vi "findmovablepath13.vi"(8 "x":dbl) -> (0 "shift":dbl, 3 "theta handle":dbl=0.15)   [LabVIEW 2012]
uses:
  G_NAV.vi
  G_VEH.vi
  G_PATH.vi
  <vilib>/Analysis/Matrix/Numeric/Conversions/Array To Matrix - RA2.vi
  <vilib>/Analysis/7linalg.llb/Real SVD Decomposition.vi
  G_SEN.vi
  <vilib>/Analysis/NI_AALPro.lvlib
  <vilib>/Analysis/Matrix/NI_Matrix.lvlib
panel:
  out "M6006 2":T1={"GPSTime"=22892800.0, "attitude[2]"=-0.6123908162117004, "lcc[0]"=-970.4720458984375, "lcc[1]"=200.52362060546875, "heading_GPS"=-0.610690712928772} {"GPSTime" format="%#_6f"}
  in  "Numeric":dbl
  out "sensor_obs":dbl[][](array[numeric])=[[-2.6493086559458767, 9.313377271515247, 0.316177936945349, -1.2], [-2.6066100840450477, 9.354542103994737, 0.3157590885476819, -1.2], [-2.579340659822815, 9.43207739327695, 0.31450254335468053, -1.2], [-2.6132527619437576, 9.439068677849818, 0.5859163050429868, 1.2000000000000006], [-2.6655003955140795, 9.41719146151926, 0.4953083793337705, 0.40000000000000013], [-2.8189313467074544, 9.344249551531279, 0.5859163050429868, 1.2000000000000006], [-2.5692189092921667, 9.480018973387281, 0.5863351534406539, 1.2000000000000006], [-2.6731933264342116, 9.434269134901442, 0.5863351534406539, 1.2000000000000006], [-2.77635346299322, 9.386711660550553, 0.5863351534406539, 1.2000000000000006], [-2.7290628288714722, 9.419794899689457, 0.5865445776394874, 1.2000000000000006], [-3.035140869949269, 9.26885391372332, 0.5865445776394874, 1.2000000000000006], [-2.550914688564252, 9.509578404068655, 0.3132459981616791, -1.2], [-2.785425991035746, 9.405948172518677, 0.495587629745689, 0.40000000000000013], [-2.7463409502228373, 9.457274042188466, 0.4957970675546278, 0.40000000000000013], [-2.90576588154835, 9.392310316924437, 0.49586688015760744, 0.40000000000000013], [-2.494747129058042, 9.597974241579312, 0.5880105470313224, 1.2000000000000006], [-2.836998990617639, 9.447892074399023, 0.4039934946364334, -0.3999999999999999], [-3.1184925197733824, 9.303796817000539, 0.5880105470313224, 1.2000000000000006], [-2.970577318209098, 9.393517402151646, 0.4960763179665463, 0.40000000000000013], [-2.9699981982750367, 9.392368449256733, 0.588219971230156, 1.2000000000000006], [-3.0729809459427746, 9.340776068194645, 0.4960763179665463, 0.40000000000000013], [-3.1996655181339673, 9.27234939560896, 0.40392368203345375, -0.3999999999999999], [-3.4973819131319495, 9.096981036828707, 0.40392368203345375, -0.3999999999999999], [-2.5289827185611418, 9.605504378157487, 0.3115706045710105, -1.2], [-3.453631348161608, 9.135814142218397, 0.4038538694304742, -0.3999999999999999], [-3.2339632015510937, 9.274656811335685, 0.5886388196278232, 1.2000000000000006], [-2.483097010676977, 9.64588076688389, 0.3111517561733434, -1.2], [-2.8803018639560647, 9.47148380231442, 0.4962857557754851, 0.40000000000000013], [-2.9317308980723027, 9.444962161904348, 0.5888482438266567, 1.2000000000000006], [-2.9582194094409178, 9.433270224287725, 0.4037142442245149, -0.3999999999999999], [-3.0350382771601945, 9.392890956174119, 0.5888482438266567, 1.2000000000000006], [-2.4599617564514022, 9.665942841266034, 0.5890576680254903, 1.2000000000000006], [-3.1930649800894275, 9.320188914278454, 0.5890576680254903, 1.2000000000000006], [-3.424919733239901, 9.200023640728578, 0.4035746190185557, -0.3999999999999999], [-3.4490855593711203, 9.183917089574846, 0.5892670922243238, 1.2000000000000006], [-2.6822275888719656, 9.595825896338217, 0.49649519358442396, 0.40000000000000013], [-3.1777999006997932, 9.352779338748892, 0.40350480641557607, -0.3999999999999999], [-3.3543988506422, 9.251882705008573, 0.5894765164231575, 1.2000000000000006], [-2.4169315260491846, 9.715129108585124, 0.589685940621991, 1.2000000000000006], [-2.4440270491484113, 9.70452412526726, 0.3103140593780091, -1.2], [-2.4445036099706936, 9.705733945395902, 0.40343499381259645, -0.3999999999999999], [-2.8187951120879293, 9.544925625371082, 0.40343499381259645, -0.3999999999999999], [-2.923864294836344, 9.494810195959495, 0.40343499381259645, -0.3999999999999999], [-3.4095769435307015, 9.230983589588824, 0.589685940621991, 1.2000000000000006], [-3.032582634559555, 9.45177853739907, 0.40336518120961684, -0.3999999999999999], [-3.2893092213922506, 9.313834366383366, 0.40336518120961684, -0.3999999999999999], [-3.313999270308597, 9.298296139668594, 0.5898953648208245, 1.2000000000000006], [-2.424651387634039, 9.734980699717582, 0.4967046313933628, 0.40000000000000013], [-2.533097518783729, 9.691715080471495, 0.4967046313933628, 0.40000000000000013], [-2.6407720438905313, 9.646563404831404, 0.4967046313933628, 0.40000000000000013], [-3.4004241638790518, 9.27277469308272, 0.4032255560036576, -0.3999999999999999], [-2.6217419806033297, 9.676437047583807, 0.403155743400678, -0.3999999999999999], [-2.6755410498513874, 9.653323143325384, 0.403155743400678, -0.3999999999999999], [-2.782523848427478, 9.605691332564723, 0.403155743400678, -0.3999999999999999], [-3.072259099823128, 9.465159649093863, 0.496844256599322, 0.40000000000000013], [-3.1500774192579093, 9.424433970288224, 0.403155743400678, -0.3999999999999999], [-3.605192513867668, 9.159018691750026, 0.403155743400678, -0.3999999999999999], [-2.5981277248582337, 9.69583138333276, 0.5907330616161588, 1.2000000000000006], [-3.102875064220138, 9.460567540591395, 0.4030859307976984, -0.3999999999999999], [-3.3599181191701257, 9.319548891673922, 0.4030859307976984, -0.3999999999999999], [-3.385278626883318, 9.304833131837459, 0.49691406920230163, 0.40000000000000013], [-2.5247869108477885, 9.749066890716904, 0.40294630559173916, -0.3999999999999999], [-2.5792234787521573, 9.726796302794572, 0.40294630559173916, -0.3999999999999999], [-3.551164984637863, 9.238618668727831, 0.5913613342126596, 1.2000000000000006], [-2.394482152160173, 9.820127604989409, 0.5915707584114931, 1.2000000000000006], [-2.7494727028492556, 9.675416799445248, 0.40280668038577994, -0.3999999999999999], [-3.681670154810481, 9.169274879714472, 0.40280668038577994, -0.3999999999999999], [-2.349619394154346, 9.868922054648976, 0.5921990310079939, 1.2000000000000006], [-2.625703441413957, 9.761592003343525, 0.497402757423159, 0.40000000000000013], [-3.2137622211581482, 9.48110235361721, 0.497402757423159, 0.40000000000000013], [-3.7275762623275384, 9.185498662423365, 0.5924084552068274, 1.2000000000000006], [-2.3569997188774257, 9.88892730018629, 0.4975423826291182, 0.40000000000000013], [-3.6331178758069624, 9.258143332791025, 0.5926178794056609, 1.2000000000000006], [-3.280263464375405, 9.479130763175284, 0.4976121952320978, 0.40000000000000013], [-2.450699178158054, 9.884289629873633, 0.30675384799783845, -1.2], [-2.4511770399787394, 9.885534502477135, 0.40224817956194303, -0.3999999999999999], [-2.5345511058394776, 9.852902522117958, 0.49775182043805705, 0.40000000000000013], [-3.824786250125524, 9.17047880734031, 0.40224817956194303, -0.3999999999999999], [-2.405397050205525, 9.933526651907876, 0.3061255754013377, -1.2], [-3.4089243051435196, 9.464380504252652, 0.4979612582469959, 0.40000000000000013], [-3.56907303823246, 9.381650335067114, 0.4980310708499755, 0.40000000000000013], [-3.532949127216187, 9.438353586460368, 0.49824050865891434, 0.40000000000000013], [-3.737313762681747, 9.3103050041449, 0.5947121213939967, 1.2000000000000006], [-2.2908474536598415, 10.059979664182297, 0.595549818189331, 1.2000000000000006], [-2.3765186719612967, 10.02943138812595, 0.3044501818106692, -1.2], [-2.462262709016492, 9.999031326649108, 0.4985197590708328, 0.40000000000000013], [-3.657097646318684, 9.409803942456133, 0.4985197590708328, 0.40000000000000013], [-3.835868568229564, 9.295365230962426, 0.40148024092916723, -0.3999999999999999], [-2.3581413988349413, 10.067967806625958, 0.5961780907858316, 1.2000000000000006], [-3.877029743260587, 9.302385055789298, 0.5961780907858316, 1.2000000000000006], [-3.9331436519651666, 9.276595165706414, 0.5963875149846652, 1.2000000000000006], [-3.425151432335213, 9.616047962173518, 0.4989386346887105, 0.40000000000000013], [-2.3143719287589564, 10.127343415537375, 0.49900844729169014, 0.40000000000000013], [-3.7975482431761254, 9.403949992407117, 0.49900844729169014, 0.40000000000000013], [-3.854407472044735, 9.378948406292697, 0.49907825989466975, 0.40000000000000013], [-2.407763132093687, 10.115274836822742, 0.4008519275023507, -0.3999999999999999], [-2.468901871015975, 10.10337801061548, 0.4007821148993711, -0.3999999999999999], [-2.3890129763037065, 10.15395227178771, 0.4993575103065882, 0.40000000000000013], [-3.777898705712374, 9.487607060347795, 0.4994273229095678, 0.40000000000000013], [-4.0346920104398265, 9.315984499311078, 0.5982723327741674, 1.2000000000000006], [-4.015722357091047, 9.342912286209264, 0.40050286448745265, -0.3999999999999999], [-2.372846250599384, 10.200711102617147, 0.30109939462933205, -1.2], [-2.3833228936159903, 10.23029622982958, 0.4001538014725545, -0.3999999999999999], [-3.9666747963375277, 9.4365483588187, 0.4998461985274455, 0.40000000000000013], [-2.30100181314674, 10.278532756817912, 0.5999477263648358, 1.2000000000000006], [-4.109576508398126, 9.423930057048132, 0.5003348867483028, 0.40000000000000013], [-2.35334151682133, 10.334600032038626, 0.2985863042433292, -1.2], [-4.074608378760497, 9.48436394539886, 0.5005443245572416, 0.40000000000000013], [-2.3368079650044735, 10.384014278769136, 0.5007537623661805, 0.40000000000000013], [-2.370078405901655, 10.38320748736416, 0.39917642503083994, -0.3999999999999999], [-4.204212822255533, 9.504238162023881, 0.3988273620159418, -0.3999999999999999], [-2.2707767805352264, 10.48873231405309, 0.2960732138573263, -1.2], [-2.3200348724405737, 10.53572713543776, 0.6051833313356751, 1.2000000000000006], [-2.245779677656643, 10.622703152908741, 0.29356012347132354, -1.2], [-2.279884830624796, 10.622358187824348, 0.6066493007275101, 1.2000000000000006], [-2.358065997017253, 10.651060149761754, 0.5025688900436505, 0.40000000000000013], [-2.206922249961846, 10.718517420078616, 0.29188472988065495, -1.2], [-2.310815072326706, 10.718984235455277, 0.5029179530585486, 0.40000000000000013], [-2.250256927274077, 10.7470116403635, 0.6089529669146794, 1.2000000000000006], [-2.4078141528407944, 10.696197951674801, 0.2910470330853207, -1.2], [-2.2625570787999116, 10.786624601979373, 0.5032670160734467, 0.40000000000000013], [-2.37319268235858, 10.803936049039782, 0.3963839209116553, -0.3999999999999999], [-2.4400133449020482, 10.792431192800741, 0.3963141083086757, -0.3999999999999999], [-2.3484550625403937, 10.948347869936686, 0.3954763570729203, -0.3999999999999999], [-2.2532005442925973, 10.986565753726355, 0.6137697234878515, 1.2000000000000006], [-2.2241527610867795, 11.130722431723722, 0.6164922380726879, 1.2000000000000006], [-2.3272220554510197, 11.112000353866012, 0.3944291680282261, -0.3999999999999999], [-2.2968682826047866, 11.131657762965752, 0.5056406445747536, 0.40000000000000013], [-2.2805508875817773, 11.32421563798276, 0.5068972714283867, 0.40000000000000013], [-2.3203488195890745, 11.3333663356091, 0.39296310336565415, -0.3999999999999999], [-2.2253235316083524, 11.390402063747686, 0.6217278430435271, 1.2000000000000006], [-2.23390046248441, 11.420813566670208, 0.5074557722522236, 0.40000000000000013], [-2.315297365324197, 11.574401473618405, 0.391357413497123, -0.3999999999999999], [-2.2168668356954866, 11.63137340411444, 0.6265445996166993, 1.2000000000000006], [-2.3994033185138965, 11.600249851280598, 0.2730365519856337, -1.2], [-2.233080590823236, 11.690844769333019, 0.5092708999296937, 0.40000000000000013], [-2.3589382981537037, 11.726595493110718, 0.27073288579846444, -1.2], [-2.3008663461775223, 11.796656013544418, 0.38989134883455107, -0.3999999999999999], [-2.209460232985442, 11.892117815907735, 0.6317802045875385, 1.2000000000000006], [-2.2516708194251622, 11.903349900014954, 0.3892630354077345, -0.3999999999999999], [-2.324463966690179, 11.881746284197003, 0.26780094701479445, -1.2], [-2.2175289279374653, 11.922764866099948, 0.5108067771952451, 0.40000000000000013], [-2.2538194745555633, 11.911368790129554, 0.2675915228159609, -1.2], [-2.178403555854863, 12.077484518563601, 0.5117841536369597, 0.40000000000000013], [-2.1829008579162608, 12.095192687788384, 0.6357592643653763, 1.2000000000000006], [-2.2383426880850124, 12.155028982889158, 0.3875875329362237, -0.3999999999999999], [-2.2804615843118747, 12.317890670472249, 0.25921455486261813, -1.2], [-2.2227746224162255, 12.415062075134333, 0.2575391612719496, -1.2], [-2.186230627716147, 12.434387153701119, 0.6426702629268841, 1.2000000000000006], [-2.196164124819029, 12.474982005763925, 0.5145068451531648, 0.40000000000000013], [-2.1425536546232067, 12.599100045840768, 0.6458116259093877, 1.2000000000000006], [-2.2643337612516414, 12.581746676789589, 0.3846554036110799, -0.3999999999999999], [-2.198573038349574, 12.65771577116447, 0.2527224046987775, -1.2], [-2.1750587039156537, 12.73714405461915, 0.5162521602276552, 0.40000000000000013], [-2.238686482838199, 12.824800292270476, 0.38304971374254876, -0.3999999999999999], [-2.1747996213790666, 12.920092091405744, 0.24748679972793824, -1.2], [-2.1535345564869504, 13.01725329936264, 0.6543980180615641, 1.2000000000000006], [-2.187058282696622, 13.165406851352257, 0.519184289552799, 0.40000000000000013], [-2.0682676188644926, 13.230434114169201, 0.24162292216059827, -1.2], [-2.249455724453499, 13.24346320074072, 0.3801873970203845, -0.3999999999999999], [-2.168249294443763, 13.280340530506738, 0.2401569527687633, -1.2], [-2.1361605605328022, 13.338559010168616, 0.6608901682254047, 1.2000000000000006], [-2.1577943406236098, 13.438198159944571, 0.520999417230269, 0.40000000000000013], [-2.1011219599138715, 13.601533356858653, 0.6661257731962439, 1.2000000000000006], [-2.2400954133839512, 13.604417430165359, 0.377743955916098, -0.3999999999999999], [-2.1622288912277443, 13.672487145254262, 0.3773948929011999, -0.3999999999999999], [-2.0809447496291567, 13.728170217410458, 0.23136113641775338, -1.2], [-2.148368119037393, 13.828678025980699, 0.5236522961434944, 0.40000000000000013], [-2.1431530665836362, 14.033933863880375, 0.37495145179691336, -0.3999999999999999], [-2.106513383233814, 14.090157922222986, 0.6761781347402553, 1.2000000000000006], [-2.116678410658171, 14.141260966031997, 0.5257466742328829, 0.40000000000000013], [-2.0736923856429295, 14.42245242291376, 0.6828797091029295, 1.2000000000000006], [-2.0946138788714483, 14.532649102029193, 0.5283995531461083, 0.40000000000000013], [-2.152273017194013, 14.572484794069997, 0.3712513838389937, -0.3999999999999999], [-2.0231688076393577, 14.688270075344283, 0.5293769295878229, 0.40000000000000013], [-2.0756120529212976, 14.699000478760663, 0.37048344520621795, -0.3999999999999999], [-2.0476810196035475, 14.823824383301131, 0.6910472528574387, 1.2000000000000006], [8.784462172926562, 11.47924364037722, 0.6985865240154472, 1.2000000000000006], [8.643867253715156, 11.631338367097312, 0.6985865240154472, 1.2000000000000006], [-2.01182307782236, 15.20812065601524, 0.5329373723397832, 0.40000000000000013], [8.86867671544905, 11.41559660678595, 0.6990053724131143, 1.2000000000000006], [8.58702381954077, 11.72028699299172, 0.6990053724131143, 1.2000000000000006], [8.952448256526495, 11.35108640713428, 0.6994242208107815, 1.2000000000000006], [8.751204607664915, 11.589530329880938, 0.699633645009615, 1.2000000000000006], [-2.0698358361213067, 15.238622346987988, 0.36678337724829835, -0.3999999999999999], [8.78228318958885, 11.618259075505645, 0.5334958731636202, 0.40000000000000013], [9.066064089233228, 11.311820599800757, 0.7006807660037829, 1.2000000000000006], [8.586576710391817, 11.864672700124274, 0.7010996144014501, 1.2000000000000006], [8.904607069385332, 11.588375580628155, 0.5339845613844775, 0.40000000000000013], [8.9823118978036, 11.517019884769494, 0.5340543739874571, 0.40000000000000013], [-2.038520846959818, 15.363492520347437, 0.7021467353956179, 1.2000000000000006], [8.791223365347536, 11.769957155305526, 0.5342638117963959, 0.40000000000000013], [8.577157812432615, 12.002632694506751, 0.7029844321909522, 1.2000000000000006], [9.089521761789143, 11.471296644949536, 0.5344034370023552, 0.40000000000000013], [8.747614402156172, 11.874019031613333, 0.5345430622083145, 0.40000000000000013], [9.196614789945517, 11.42431028033962, 0.5347525000172533, 0.40000000000000013], [8.702856524966558, 11.977947480441758, 0.5348223126202329, 0.40000000000000013], [8.551902917074258, 12.126859885849031, 0.7044504015827872, 1.2000000000000006], [9.301763328727434, 11.37452391977877, 0.7052880983781215, 1.2000000000000006], [8.546058430068586, 12.272774370500398, 0.7065446435711229, 1.2000000000000006], [8.713762205484503, 12.13805016075561, 0.5356600638559883, 0.40000000000000013], [9.379898466547676, 11.440670196564861, 0.5357996890619475, 0.40000000000000013], [8.680290014842434, 12.256372289618902, 0.536078939473866, 0.40000000000000013], [-1.9947666269032363, 15.748326418663561, 0.5366374402977029, 0.40000000000000013], [5.4033137061696035, 14.702228724352713, 0.7105237033489606, 1.2000000000000006], [5.31065139179097, 14.760192151279867, 0.5369166907096213, 0.40000000000000013], [5.318145573506214, 14.776082090179019, 0.7111519759454614, 1.2000000000000006], [5.372647557345696, 14.763989846509837, 0.36287387148143985, -0.3999999999999999], [5.430433378499369, 14.758453624273042, 0.5372657537245195, 0.40000000000000013], [5.282599535397169, 14.828571261939807, 0.3627342462754806, -0.3999999999999999], [-2.0630447970868317, 15.828269580660534, 0.3627342462754806, -0.3999999999999999], [-2.0425899368277762, 16.04197255374355, 0.7161781567174671, 1.2000000000000006], [8.986023479525567, 16.697743175440838, 0.7844504455372108, 1.2000000000000006], [8.870510744967275, 16.775657498704163, 0.7844504455372108, 1.2000000000000006], [8.776249405862337, 16.886004939029128, 0.7852881423325451, 1.2000000000000006], [9.255378545456706, 16.596057732863006, 0.7859164149290457, 1.2000000000000006], [9.146441633836046, 16.684541131912827, 0.7861258391278794, 1.2000000000000006], [9.094705994581439, 16.85736482840408, 0.5628171664150587, 0.40000000000000013], [9.445245140600367, 16.620273164434607, 0.7886389295138823, 1.2000000000000006], [8.745638718171325, 17.096618222434593, 0.7886389295138823, 1.2000000000000006], [9.250822015437112, 16.835004830220694, 0.563305854635916, 0.40000000000000013], [8.898582257650931, 17.072593546817984, 0.563305854635916, 0.40000000000000013], [9.372609476756939, 16.761935663932476, 0.5633756672388956, 0.40000000000000013], [9.022240713238299, 17.00273744358763, 0.5633756672388956, 0.40000000000000013], [9.671704217358442, 16.690540187776413, 0.79261798929172, 1.2000000000000006], [8.733353836557999, 17.341528099528503, 0.7928274134905535, 1.2000000000000006], [9.575618663038583, 16.801373411419853, 0.5644228562835899, 0.40000000000000013], [8.86635551362631, 17.284293500790973, 0.5644228562835899, 0.40000000000000013], [-11.730647795102412, 15.437193920648374, 0.09942389115260453, -1.2], [-11.753961919567294, 15.46091854606451, 0.3329242648031848, -0.3999999999999999], [-2.6376199176507695, 22.880864643377365, 0.586553451428128, 0.40000000000000013], [-2.8095170709695823, 22.87690194098971, 0.5866930766340872, 0.40000000000000013], [-2.472177558679492, 22.932903386537202, 0.5867628892370669, 0.40000000000000013], [-2.1457138125258957, 23.092372962417727, 0.5876006404728222, 0.40000000000000013], [-1.975660428365826, 23.120301035359756, 0.5876704530758019, 0.40000000000000013], [-2.830488522803034, 23.021539526550544, 0.8631939442986329, 1.2000000000000006], [-2.321307029798844, 23.112624067398425, 0.5878798908847407, 0.40000000000000013], [-2.664069979468923, 23.075216022238337, 0.8638222168951337, 1.2000000000000006], [-2.4981915740055283, 23.137390254704062, 0.864659913690468, 1.2000000000000006], [-2.3314305321547493, 23.198157106933053, 0.8654976104858023, 1.2000000000000006], [-1.8217528316749911, 23.325992950774253, 0.5889968925324145, 0.40000000000000013], [-2.1768599709453524, 23.37676650480826, 0.8688483976671393, 1.2000000000000006], [-15.001217509405912, 16.7719561296704, 0.31016535623183017, -0.3999999999999999], [-15.131558329077535, 16.65366297795977, 0.31002573102587094, -0.3999999999999999], [-14.921984448489132, 16.935815146369087, 0.30981629321693205, -0.3999999999999999], [-15.241790010790758, 16.749485916960253, 0.026963118356189475, -1.2], [-15.133075455565274, 16.88861418597005, 0.0267536941573559, -1.2], [-15.017973364486107, 17.261437164441947, 0.3077917277305232, -0.3999999999999999], [9.64601974480163, 21.452115753566822, 0.5922780848724565, 0.40000000000000013], [9.496453028675626, 21.54978831901161, 0.8772253656204823, 1.2000000000000006], [9.33857931433906, 21.631972172843444, 0.8772253656204823, 1.2000000000000006], [9.17999443103193, 21.712775206793534, 0.8772253656204823, 1.2000000000000006], [-15.156829567346312, 17.1472706411717, 0.022774634379518044, -1.2], [9.377029264437805, 21.70662736414938, 0.5929762109022526, 0.40000000000000013], [9.544865059367709, 21.641804454240944, 0.5931158361082118, 0.40000000000000013], [9.710389454590258, 21.571913609233842, 0.8797384560064849, 1.2000000000000006], [-1.8772014233671248, 23.929435618135358, 0.8797384560064849, 1.2000000000000006], [9.095883042737146, 21.944626194626313, 0.8807855770006529, 1.2000000000000006], [9.271801932592034, 21.894917952170292, 0.5938139621380081, 0.40000000000000013], [-15.236180272734178, 17.461386956855613, 0.017120181011011648, -1.2], [9.194957789557106, 22.145529906980062, 0.5951404015946207, 0.40000000000000013], [5.3379716006680615, 24.14040468850077, 0.30115953044745974, -0.3999999999999999], [5.346343602955266, 24.94301298686431, 0.29571414741504976, -0.3999999999999999], [-16.03827076279453, 20.400810973707614, 0.28733663505749585, -0.3999999999999999], [-15.917453817284267, 20.56937941691859, 0.2870573846455774, -0.3999999999999999], [-15.794914133758107, 20.737124067829413, 0.28677813423365894, -0.3999999999999999], [-14.857892347507073, 21.847969012040384, 0.2851724443651278, -0.3999999999999999], [-15.023801434595246, 21.725328510394597, 0.2851026317621482, -0.3999999999999999], [-15.339589077483758, 21.460351215716504, 0.2851026317621482, -0.3999999999999999], [-15.650704132941332, 21.189903024072276, 0.2851026317621482, -0.3999999999999999], [-15.201556508849778, 21.61650958244562, 0.28489319395320933, -0.3999999999999999], [-14.728337374906722, 22.016057756865447, 0.2848233813502297, -0.3999999999999999], [-15.626945243640977, 21.4767441096572, 0.28370637970255586, -0.3999999999999999], [9.50763508171292, 26.73975570562619, 0.6252994460818146, 0.40000000000000013], [-1.4252219468434035, 28.59895493907886, 0.6255088838907534, 0.40000000000000013], [9.725543674751258, 26.692789231824694, 0.6255786964937331, 0.40000000000000013], [9.943355423856874, 26.64378657215293, 0.6258579469056516, 0.40000000000000013], [9.334114379546264, 26.89614247546073, 0.6258579469056516, 0.40000000000000013], [9.216574706656742, 27.200382540182076, 0.6275334493771623, 0.40000000000000013], [10.040081267648652, 26.868922071117122, 0.9827751618326013, 1.2000000000000006], [-1.4946609322957394, 29.821814277404098, 1.0022516123241232, 1.2000000000000006], [9.883884675811041, 31.803099088007194, 0.6592981837328874, 0.40000000000000013], [9.665449175747526, 31.97349509801759, 0.659926497159704, 0.40000000000000013], [10.174424429491456, 31.838119222564067, 0.6602057475716224, 0.40000000000000013], [10.17244090528941, 31.83259465007272, 1.0805762626878783, 1.2000000000000006], [-1.0364518801246452, 37.42334336490329, 0.6869439745128152, 0.40000000000000013], [10.026103833352638, 36.8130958059697, 0.6928780457660825, 0.40000000000000013], [9.743408822772697, 36.92812129013003, 0.6930874835750214, 0.40000000000000013], [10.347031193921643, 36.82288619877287, 1.1808904539291583, 1.2000000000000006], [-21.069030510629236, 31.45954783569295, 0.20558607696836614, -0.3999999999999999], [-21.391355310423045, 31.377757000004777, 0.20467851312963112, -0.3999999999999999], [10.4210427571751, 41.72394225688742, 0.7265975330052368, 0.40000000000000013], [10.107451026305094, 41.89078819565647, 0.7271560338290737, 0.40000000000000013], [10.474235594988285, 41.919051326913184, 1.284136583954108, 1.2000000000000006], [10.13857155297352, 42.00899223589921, 1.284136583954108, 1.2000000000000006], [10.830210018606069, 41.90102810572798, 0.7285522858886659, 0.40000000000000013], [-0.709038750028526, 57.66347671663537, 1.5846603092802805, 1.2000000000000006], [11.120605021860856, 56.96437033164037, 0.8312466248716806, 0.40000000000000013], [-0.7151980727209852, 58.133987434462625, 0.8314560626806193, 0.40000000000000013], [1.5195348183779678, 61.52869356204023, 0.04473783970333195, -0.3999999999999999], [5.073212151726797, 61.48708023724171, 0.04362083805565814, -0.3999999999999999], [11.439817695944253, 61.011847285540675, 0.8593811038724656, 0.40000000000000013], [11.689176472740309, 65.06866600393317, 0.8875155828732506, 0.40000000000000013], [14.49832831315618, 65.07219891982305, 1.7750269060199955, 1.2000000000000006], [8.818111571073048, 72.81602044955893, 1.9136657256478184, 1.2000000000000006], [12.551831810983316, 72.91253923612891, 0.9424581014182081, 0.40000000000000013], [13.768405529858791, 72.71844886386302, 1.9283254195661683, 1.2000000000000006], [1.2476421313017925, 74.97736983119862, -0.04909029870127124, -0.3999999999999999], [0.9387629168292289, 75.21210795753403, 0.9506959885698028, 0.40000000000000013], [17.77975821366545, 76.1598746565128, 2.0169118556727685, 1.2000000000000006], [47.35648972259149, 63.571420836353425, 2.052304545275642, 1.2000000000000006], [13.031972557350265, 79.3416128979354, 2.061938058421986, 1.2000000000000006], [24.83184721270082, 81.07466865802802, 2.156178947897092, 1.2000000000000006], [13.551875448365177, 86.71163580640813, 1.0385900557211387, 0.40000000000000013], [52.872675769586, 69.37798867554798, 2.2194250559448303, 1.2000000000000006], [8.915518332671137, 92.0400907270114, 1.0712623539155988, 0.40000000000000013], [9.692181670683942, 91.99867908899289, 1.0715416043275172, 0.40000000000000013], [20.71894414488982, 95.06455786989261, 2.4164932270472192, 1.2000000000000006], [19.150342204408794, 95.56882049865551, 2.4198440142285564, 1.2000000000000006], [23.490178905085354, 95.9928006820069, 2.448953977866423, 1.2000000000000006], [26.036285319817722, 95.81770414584793, 2.4592157636092677, 1.2000000000000006], [14.717578948116746, 99.12164584891, 1.1254369338277803, 0.40000000000000013], [20.65463162219833, 155.2673630873944, 3.658378726130288, 1.2000000000000006], [12.312708261276875, 191.3556263648354, 4.393457664036117, 1.2000000000000006], [14.978259637770336, 232.0240814937235, 2.048848233439155, 0.40000000000000013], [33.73593705129936, 288.53349296533526, 2.4538311433239053, 0.40000000000000013], [8.92096999050232, 17.23708913161584, 0.3356469563193898, -0.3999999999999999], [-2.5256202703736608, 22.68399055587274, 0.31491261323444397, -0.3999999999999999], [-1.8996165215080512, 23.228271875851924, 0.3116314208944021, -0.3999999999999999], [-3.0296332585078587, 23.183843349397314, 0.8671730040764709, 1.2000000000000006], [5.104128617356655, 23.236200962780366, 0.022984058578351618, -1.2], [-1.2548826959515347, 24.01715071826592, 0.01942384719818102, -1.2], [5.221948215230284, 24.444090337557157, -0.0021468452816766903, -1.2], [-2.224688830349968, 25.593404278777417, 0.9151311456093583, 1.2000000000000006], [5.209357772395169, 25.198536731676327, -0.017434811796527283, -1.2], [-1.1725915542855405, 25.874379726198075, -0.019319629586029397, -1.2], [-15.005798944565672, 21.383214801932546, -0.039005504276384995, -1.2], [-14.976356804490646, 21.66777357175441, -0.04319398825305637, -1.2], [-14.955664951264778, 21.9687081224078, -0.04780132062739484, -1.2], [9.275033221452706, 26.45651279141699, 0.277143995022472, -0.3999999999999999], [9.363878146139614, 27.271589550954324, 0.2716287993870824, -0.3999999999999999], [9.371321144452127, 28.564736959442584, 0.26318147442654893, -0.3999999999999999], [10.747513637749273, 30.43885569655537, 1.0575396008161857, 1.2000000000000006], [11.012472531760006, 30.418068389611857, 1.0592149944068543, 1.2000000000000006], [11.266285997376329, 30.367042635463775, 1.060262115401022, 1.2000000000000006], [-20.735017036098906, 31.521767273772653, 0.20663326601306034, -0.3999999999999999], [-20.49557227262787, 31.709735125755284, 0.20656345341008076, -0.3999999999999999], [10.724864676049275, 37.00446773130826, 0.6956007372822874, 0.40000000000000013], [-21.806198041420327, 31.41066071306105, 0.20272376024620187, -0.3999999999999999], [10.97816933233072, 46.72664514439962, 0.7613642092890853, 0.40000000000000013], [-33.95444016665767, 37.454440166657676, 0.11475988049188635, -0.3999999999999999], [-33.46782468155926, 38.15694699438283, 0.11364287884421248, -0.3999999999999999], [-32.258000408687934, 39.32613895725404, 0.11343344103527364, -0.3999999999999999], [-34.39923085728631, 37.30403001674005, 0.11329381582931441, -0.3999999999999999], [11.618566184124763, 57.01187131155995, 0.8322938139163747, 0.40000000000000013], [16.615400312068406, 60.50485600252477, 1.6937703168725702, 1.2000000000000006], [13.205163345895427, 64.3192947748755, 1.7536656377389712, 1.2000000000000006], [20.538690765112868, 64.00503191176435, 1.7884300547453438, 1.2000000000000006], [13.026046392769018, 79.30712465157343, 0.9869985421192027, 0.40000000000000013], [27.29899080749756, 81.67230442986731, 2.1844512147396244, 1.2000000000000006], [33.69042505267091, 80.06731529671714, 2.2022522716404778, 1.2000000000000006], [29.157427120978678, 82.5346645544511, 2.2146082993716583, 1.2000000000000006], [27.17382907061827, 93.78874887901951, 2.425079619199396, 1.2000000000000006], [34.761055666251615, 92.88790635480824, 2.4590063394104344, 1.2000000000000006], [-2.729118001525531, 22.918683596868465, 0.31309748555697403, -0.3999999999999999], [9.124522914489708, 21.80096170236561, 0.3072332269066863, -0.3999999999999999], [-1.5170192378515415, 28.303045293335575, 0.2765156815956554, -0.3999999999999999], [-1.3900091234452605, 30.022954081648294, 0.2645777264861412, -0.3999999999999999], [4.034616118215339, 61.19769858054814, 0.04620390436590388, -0.3999999999999999], [26.121526235859253, 82.71602090547535, 2.197226090868472, 1.2000000000000006]]
  out "xplot":cluster{dbl[]}[](array[cluster])
  out "yplot":cluster{dbl[]}[](array[cluster])
  out "thetaseed":dbl[](array[numeric])
  out "center":i16
  out "right":i16
  out "left":i16
  out "XY Graph":cluster{"Y":dbl[], "Y":dbl[]}[](graph)=[{"Y"=[0.0], "Y"=[1000.0]}, {"Y"=[], "Y"=[]}, {"Y"=[], "Y"=[]}, {"Y"=[55.79381017995934], "Y"=[-143.41137512848826]}, {"Y"=[1.8243630881955273], "Y"=[-0.6091599202647308]}, {"Y"=[60.825233010671326, 56.37330625127248, 55.349089235151354, 59.801015994550255, 60.825233010671326], "Y"=[-144.72018116547483, -142.44414335187238, -144.44751039360185, -146.72354820720435, -144.72018116547483]}, {"Y"=[0.0, 2.210107140854234e-06, 8.840428449730098e-06, 1.9890964154001267e-05, 3.536171391260723e-05, 5.5252677611861145e-05, 7.956385525176302e-05, 0.00010829524660493917, 0.00014144685155770276, 0.0001790186695416196, 0.00022101070067037654, 0.00026742294460291305, 0.00031825540077079495, 0.00037350806894664856, 0.0004331809489031002, 0.0004972740399580289, 0.0005657873416566872, 0.0006387208537717015, 0.0007160745756209508, 0.0007978485066360008, 0.0008840426462484174, 0.0009746569938897665, 0.0010696915488779268, 0.0011691463105307776, 0.0012730212781661976, 0.001381316451102066, 0.0014940318285425747, 0.0016111674095782291, 0.0017327231935269083, 0.0018586991794791174, 0.001989095366525362, 0.00212391175364246, 0.002263148340148291, 0.0024068051247922995, 0.002554882106551304, 0.0027073792846294964, 0.002864296657776322, 0.003025634224741225, 0.003191391984614711, 0.0033615699362599116, 0.003536168078198898, 0.0037151864094084885, 0.003898624928524441, 0.004086483634296201, 0.004278762525359525, 0.004475461600350172, 0.0046765808579039, 0.004882120296656467, 0.0050920799150162566, 0.00530645971150534, 0.005525259684645789, 0.005748479832959674, 0.005976120154741693, 0.006208180648513917, 0.006444661312457356, 0.006685562145094082, 0.006930883144491418, 0.007180624309171435, 0.007434785636974084, 0.007693367126535122, 0.007956368775921874, 0.008223790583087975, 0.008495632546100751, 0.008771894663368585, 0.009052576932504053, 0.00933767935191554, 0.009627201919329309, 0.009921144632812684, 0.010219507490205615, 0.010522290489461739, 0.010829493628421005, 0.011141116904923365, 0.011457160316581394, 0.011777623861462416, 0.012102507536951634, 0.012431811341116372, 0.012765535271228146, 0.013103679325240591, 0.0134462435006526, 0.013793227794963059, 0.014144632205784546, 0.014500456730615952, 0.014860701366956164, 0.015225366112190386, 0.015594450963703821, 0.015967955919109045, 0.0163458809754502, 0.016728226130226176, 0.017114991380822175, 0.017506176724168654, 0.0179017821577645, 0.018301807678767545, 0.018706253284335617, 0.019115118971512857, 0.019528404737457095, 0.01994611057932616, 0.02036823649393682, 0.02079478247856059, 0.021225748530014243, 0.02166113464522823, 0.022100940821246695], "Y"=[0.0, 0.05249999993797367, 0.10499999950378934, 0.15749999832528905, 0.2099999960303148, 0.26249999224670867, 0.31499998660231265, 0.3674999787249688, 0.41999996824251923, 0.472499954782806, 0.5249999379736712, 0.577499917442957, 0.6299998928185055, 0.682499863728159, 0.7349998297997596, 0.7874997906611497, 0.8399997459401715, 0.8924996952646672, 0.9449996382624795, 0.9974995745614504, 1.0499995037894228, 1.1024994255742389, 1.1549993395437415, 1.2074992453257731, 1.2599991425481762, 1.3124990308387938, 1.3649989098254687, 1.4174987791360436, 1.4699986383983614, 1.5224984872402658, 1.574998325289599, 1.6274981521742047, 1.6799979675219257, 1.7324977709606055, 1.784997562118088, 1.837497340622216, 1.8899971061008334, 1.9424968581817836, 1.994996596492911, 2.047496320662059, 2.099996030317072, 2.152495725085793, 2.204995404596067, 2.2574950684757384, 2.309994716352652, 2.3624943478546507, 2.414993962609581, 2.467493560245286, 2.519993140389611, 2.5724927026704023, 2.6249922467155042, 2.6774917721527607, 2.7299912786100196, 2.7824907657151243, 2.834990233095921, 2.887489680380256, 2.939989107195975, 2.9924885131709242, 3.0449878979329497, 3.0974872611098974, 3.1499866023296144, 3.2024859212199472, 3.2549852174087435, 3.3074844905238483, 3.3599837401931105, 3.412482966044377, 3.464982167705495, 3.5174813448043127, 3.5699804969686775, 3.6224796238264374, 3.6749787250054404, 3.7274778001335362, 3.7799768488385714, 3.8324758707483966, 3.884974865490859, 3.9374738326938097, 3.989972771985096, 4.042471682992569, 4.094970565344078, 4.147469418667473, 4.199968242590603, 4.2524670367413195, 4.304965800747474, 4.3574645342369145, 4.409963236837495, 4.4624619081770645, 4.514960547883476, 4.567459155584579, 4.6199577309082285, 4.672456273482274, 4.724954782934569, 4.777453258892966, 4.829951700985317, 4.882450108839476, 4.934948482083297, 4.987446820344632, 5.039945123251335, 5.09244339043126, 5.144941621512262, 5.197439816122197, 5.249937973888915]}, {"Y"=[55.85492946607054, 56.300112183962334, 56.74529490185413, 57.19047761974598, 57.635660337637766, 58.08084305552956, 58.52602577342136, 58.97120849131315, 59.416391209205, 59.8615739270968, 60.306756644988596, 60.75193936288038, 61.197122080772175, 61.64230479866403, 62.087487516555825, 62.532670234447615, 62.97785295233941, 63.423035670231265, 63.86821838812306, 64.31340110601485, 64.75858382390665, 65.20376654179844, 65.64894925969023, 66.09413197758208, 66.53931469547388, 66.98449741336567, 67.42968013125746, 67.87486284914931, 68.3200455670411, 68.7652282849329, 69.2104110028247, 69.65559372071655, 70.10077643860835, 70.54595915650015, 70.99114187439193, 71.43632459228371, 71.88150731017556, 72.32669002806736, 72.77187274595916, 73.21705546385095], "Y"=[-143.26925304077835, -143.49687629901547, -143.72449955725253, -143.95212281548962, -144.17974607372668, -144.40736933196374, -144.63499259020085, -144.8626158484379, -145.090239106675, -145.3178623649121, -145.54548562314918, -145.7731088813862, -146.00073213962332, -146.22835539786038, -146.45597865609744, -146.68360191433456, -146.91122517257162, -147.1388484308087, -147.36647168904577, -147.59409494728285, -147.82171820551994, -148.04934146375703, -148.27696472199406, -148.50458798023115, -148.73221123846827, -148.9598344967053, -149.18745775494241, -149.4150810131795, -149.64270427141656, -149.87032752965362, -150.09795078789074, -150.3255740461278, -150.55319730436486, -150.78082056260195, -151.00844382083903, -151.23606707907612, -151.46369033731318, -151.6913135955503, -151.91893685378736, -152.14656011202442]}, {"Y"=[46.95734422441421, 47.0463827596022, 47.13542129479015, 47.224459829978144, 47.31349836516614, 47.40253690035408, 47.49157543554208, 47.58061397073008, 47.669652505918016, 47.75869104110601, 47.84772957629395, 47.936768111481946, 48.02580664666995, 48.11484518185789, 48.20388371704588, 48.292922252233886, 48.381960787421825, 48.47099932260982, 48.56003785779782, 48.64907639298576, 48.73811492817376, 48.827153463361746, 48.91619199854969, 49.00523053373769, 49.09426906892568, 49.18330760411363, 49.272346139301625, 49.361384674489564, 49.45042320967757, 49.53946174486556, 49.6285002800535, 49.717538815241504, 49.8065773504295, 49.89561588561743, 49.984654420805434, 50.07369295599343, 50.16273149118137, 50.251770026369364, 50.34080856155737, 50.429847096745306, 50.5188856319333, 50.607924167121304, 50.69696270230924, 50.78600123749724, 50.875039772685184, 50.96407830787318, 51.05311684306117, 51.142155378249115, 51.23119391343711, 51.320232448625106, 51.40927098381305, 51.49830951900105, 51.58734805418904, 51.67638658937698, 51.765425124564985, 51.85446365975298, 51.94350219494092, 52.03254073012892, 52.12157926531691, 52.21061780050485, 52.29965633569285, 52.38869487088079, 52.477733406068786, 52.56677194125679, 52.65581047644473, 52.74484901163272, 52.833887546820726, 52.922926082008665, 53.01196461719666, 53.10100315238466, 53.190041687572595, 53.27908022276059, 53.36811875794859, 53.45715729313653, 53.54619582832453, 53.635234363512524, 53.72427289870047, 53.813311433888465, 53.902349969076404, 53.99138850426441, 54.0804270394524, 54.16946557464034, 54.25850410982834, 54.34754264501633, 54.43658118020427, 54.525619715392274, 54.61465825058027, 54.70369678576821, 54.792735320956204, 54.88177385614421, 54.970812391332146, 55.05985092652014, 55.148889461708144, 55.23792799689608, 55.32696653208408, 55.41600506727202, 55.50504360246001, 55.59408213764801, 55.683120672835955, 55.77215920802395, 55.861197743211946, 55.95023627839994, 56.03927481358789, 56.12831334877588, 56.21735188396388, 56.306390419151825, 56.39542895433982, 56.48446748952781, 56.573506024715755, 56.66254455990375, 56.75158309509169, 56.84062163027969, 56.92966016546769, 57.01869870065563, 57.10773723584363, 57.196775771031625, 57.285814306219564, 57.37485284140757, 57.46389137659556, 57.552929911783494, 57.64196844697149, 57.73100698215949, 57.82004551734743, 57.90908405253543, 58.08716112291137, 58.176199658099364, 58.26523819328731, 58.354276728475305, 58.4433152636633, 58.53235379885125, 58.62139233403924, 58.71043086922723, 58.79946940441518, 58.88850793960317, 58.97754647479111, 59.06658500997911, 59.15562354516711, 59.24466208035505, 59.333700615543044, 59.42273915073105, 59.511777685918986, 59.60081622110698, 59.689854756294984, 59.778893291482916, 59.86793182667091, 59.956970361858914, 60.04600889704685, 60.13504743223485, 60.31312450261079, 60.402163037798786, 60.491201572986725, 60.58024010817473, 60.66927864336272, 60.75831717855066, 60.84735571373866, 60.93639424892665, 61.02543278411459, 61.114471319302595, 61.203509854490534, 61.29254838967853, 61.38158692486653, 61.47062546005447, 61.55966399524247, 61.64870253043047, 61.73774106561841, 61.826779600806404, 61.91581813599439, 62.00485667118234, 62.093895206370334, 62.18293374155833, 62.271972276746276, 62.36101081193427, 62.45004934712227, 62.53908788231021, 62.62812641749821, 62.71716495268615, 62.80620348787415, 62.895242023062146, 62.984280558250084, 63.07331909343808, 63.162357628626076, 63.251396163814015, 63.34043469900201, 63.42947323419001, 63.51851176937796, 63.60755030456595, 63.69658883975394, 63.78562737494189, 63.87466591012988, 63.96370444531783, 64.05274298050581, 64.14178151569382, 64.23082005088176, 64.31985858606976, 64.40889712125775, 64.4979356564457, 64.58697419163369, 64.76505126200964, 64.85408979719762, 64.94312833238557, 65.03216686757357, 65.12120540276156, 65.2102439379495, 65.29928247313751, 65.38832100832549, 65.47735954351344, 65.56639807870144, 65.65543661388938, 65.74447514907737, 65.83351368426537, 65.92255221945331, 66.0115907546413, 66.10062928982931, 66.18966782501724, 66.27870636020525, 66.36774489539324, 66.45678343058118, 66.54582196576918, 66.63486050095719, 66.72389903614511, 66.81293757133312, 66.9019761065211, 66.99101464170904, 67.08005317689705, 67.16909171208498, 67.25813024727299, 67.34716878246098, 67.43620731764892, 67.52524585283692, 67.61428438802493, 67.70332292321285, 67.79236145840086, 67.88139999358886, 67.97043852877678, 68.05947706396479, 68.14851559915279, 68.23755413434073, 68.32659266952872, 68.41563120471668, 68.50466973990466, 68.59370827509267, 68.6827468102806, 68.7717853454686, 68.8608238806566, 68.94986241584455, 69.03890095103253, 69.12793948622053, 69.21697802140848, 69.30601655659646, 69.39505509178447, 69.48409362697241, 69.5731321621604, 69.6621706973484, 69.75120923253635, 69.84024776772434, 69.92928630291229, 70.01832483810027, 70.10736337328828, 70.19640190847622, 70.2854404436642, 70.37447897885221, 70.46351751404015, 70.55255604922814, 70.64159458441614, 70.7306331196041, 70.81967165479207, 70.90871018998008, 70.99774872516802, 71.08678726035602, 71.17582579554401, 71.26486433073195, 71.35390286591995, 71.44294140110789, 71.5319799362959, 71.62101847148388, 71.71005700667183, 71.79909554185983, 71.88813407704782, 71.97717261223576, 72.06621114742377, 72.15524968261175, 72.2442882177997, 72.3333267529877, 72.42236528817568, 72.51140382336364, 72.60044235855163, 72.68948089373963, 72.77851942892757, 72.86755796411556, 72.9565964993035, 73.04563503449151, 73.13467356967949, 73.22371210486745, 73.31275064005544, 73.40178917524342, 73.49082771043138, 73.57986624561937], "Y"=[-138.89375124553214, -138.93927200180423, -138.98479275807625, -139.0303135143483, -139.07583427062036, -139.12135502689242, -139.16687578316444, -139.21239653943653, -139.25791729570855, -139.30343805198058, -139.34895880825266, -139.3944795645247, -139.44000032079677, -139.4855210770688, -139.53104183334085, -139.5765625896129, -139.62208334588496, -139.667604102157, -139.71312485842907, -139.7586456147011, -139.80416637097318, -139.8496871272452, -139.89520788351723, -139.9407286397893, -139.98624939606134, -140.0317701523334, -140.07729090860545, -140.1228116648775, -140.16833242114956, -140.2138531774216, -140.25937393369364, -140.30489468996572, -140.35041544623775, -140.39593620250977, -140.44145695878186, -140.48697771505388, -140.53249847132597, -140.578019227598, -140.62353998387005, -140.66906074014207, -140.71458149641416, -140.76010225268618, -140.80562300895826, -140.8511437652303, -140.89666452150234, -140.9421852777744, -140.98770603404643, -141.0332267903185, -141.07874754659053, -141.1242683028626, -141.16978905913462, -141.2153098154067, -141.26083057167872, -141.3063513279508, -141.35187208422283, -141.3973928404949, -141.44291359676694, -141.48843435303897, -141.53395510931105, -141.57947586558308, -141.62499662185516, -141.67051737812716, -141.71603813439924, -141.76155889067127, -141.80707964694335, -141.85260040321535, -141.89812115948743, -141.94364191575949, -141.9891626720315, -142.0346834283036, -142.08020418457562, -142.1257249408477, -142.1712456971197, -142.21676645339178, -142.2622872096638, -142.3078079659359, -142.3533287222079, -142.39884947847997, -142.44437023475203, -142.48989099102408, -142.53541174729614, -142.58093250356816, -142.62645325984025, -142.67197401611224, -142.71749477238433, -142.76301552865635, -142.80853628492844, -142.85405704120046, -142.89957779747255, -142.94509855374454, -142.99061931001663, -143.03614006628868, -143.0816608225607, -143.1271815788328, -143.17270233510482, -143.2182230913769, -143.2637438476489, -143.30926460392098, -143.354785360193, -143.4003061164651, -143.4458268727371, -143.4913476290092, -143.5368683852812, -143.58238914155328, -143.62790989782533, -143.67343065409736, -143.71895141036944, -143.76447216664147, -143.80999292291352, -143.85551367918555, -143.90103443545763, -143.94655519172966, -143.99207594800174, -144.03759670427374, -144.08311746054582, -144.12863821681785, -144.1741589730899, -144.21967972936199, -144.265200485634, -144.3107212419061, -144.3562419981781, -144.40176275445017, -144.4472835107222, -144.49280426699428, -144.58384577953836, -144.6293665358104, -144.67488729208247, -144.72040804835453, -144.76592880462653, -144.81144956089864, -144.85697031717064, -144.90249107344272, -144.94801182971474, -144.99353258598683, -145.03905334225882, -145.0845740985309, -145.13009485480293, -145.17561561107502, -145.22113636734704, -145.2666571236191, -145.31217787989118, -145.35769863616318, -145.40321939243526, -145.4487401487073, -145.49426090497937, -145.5397816612514, -145.58530241752348, -145.63082317379548, -145.7218646863396, -145.76738544261164, -145.8129061988837, -145.85842695515572, -145.90394771142783, -145.94946846769983, -145.9949892239719, -146.04050998024394, -146.08603073651602, -146.13155149278802, -146.1770722490601, -146.22259300533213, -146.2681137616042, -146.31363451787624, -146.3591552741483, -146.40467603042035, -146.45019678669237, -146.49571754296446, -146.54123829923648, -146.58675905550857, -146.6322798117806, -146.67780056805265, -146.72332132432467, -146.76884208059676, -146.81436283686878, -146.85988359314084, -146.9054043494129, -146.95092510568492, -146.99644586195703, -147.04196661822903, -147.0874873745011, -147.13300813077313, -147.17852888704522, -147.22404964331722, -147.2695703995893, -147.31509115586132, -147.3606119121334, -147.40613266840543, -147.4516534246775, -147.49717418094954, -147.54269493722157, -147.58821569349365, -147.63373644976568, -147.67925720603776, -147.72477796230976, -147.77029871858184, -147.81581947485387, -147.86134023112595, -147.90686098739798, -147.9979024999421, -148.0434232562141, -148.08894401248617, -148.13446476875822, -148.17998552503028, -148.22550628130233, -148.27102703757438, -148.3165477938464, -148.3620685501185, -148.40758930639052, -148.45311006266255, -148.49863081893463, -148.54415157520666, -148.58967233147874, -148.63519308775076, -148.6807138440228, -148.72623460029487, -148.77175535656693, -148.81727611283895, -148.86279686911104, -148.90831762538306, -148.95383838165512, -148.99935913792717, -149.0448798941992, -149.09040065047128, -149.1359214067433, -149.18144216301536, -149.22696291928742, -149.27248367555944, -149.31800443183153, -149.36352518810358, -149.4090459443756, -149.4545667006477, -149.50008745691972, -149.54560821319174, -149.59112896946382, -149.63664972573585, -149.68217048200793, -149.72769123827996, -149.77321199455199, -149.81873275082407, -149.86425350709612, -149.90977426336815, -149.95529501964023, -150.00081577591226, -150.0463365321843, -150.09185728845637, -150.1373780447284, -150.18289880100048, -150.2284195572725, -150.27394031354456, -150.3194610698166, -150.36498182608864, -150.4105025823607, -150.45602333863278, -150.5015440949048, -150.54706485117688, -150.5925856074489, -150.63810636372094, -150.68362711999302, -150.72914787626505, -150.7746686325371, -150.82018938880915, -150.86571014508118, -150.91123090135326, -150.9567516576253, -151.00227241389734, -151.04779317016943, -151.09331392644145, -151.13883468271348, -151.18435543898556, -151.2298761952576, -151.27539695152967, -151.3209177078017, -151.36643846407375, -151.4119592203458, -151.45747997661783, -151.5030007328899, -151.54852148916194, -151.594042245434, -151.63956300170608, -151.6850837579781, -151.73060451425013, -151.77612527052221, -151.82164602679424, -151.8671667830663, -151.91268753933835, -151.95820829561038, -152.00372905188246, -152.04924980815449, -152.09477056442654, -152.14029132069862, -152.18581207697065, -152.23133283324267, -152.27685358951476, -152.32237434578678, -152.36789510205887, -152.4134158583309, -152.45893661460295, -152.504457370875]}, {"Y"=[], "Y"=[]}, {"Y"=[], "Y"=[]}, {"Y"=[], "Y"=[]}, {"Y"=[-16.5, -15.25, -15.0, -13.5, -13.25, -13.25, -13.25, -13.0, -13.0, -12.75, -12.75, -12.75, -12.75, -12.75, -12.75, -12.75, -12.5, -12.5, -12.5, -12.5, -12.5, -12.5, -12.25, -12.25, -12.25, -12.25, -12.25, -12.25, -12.0, -12.0, -12.0, -11.75, -11.75, -11.75, -11.5, -11.5, -11.5, -11.5, -11.5, -11.25, -10.75, -10.75, -10.5, -10.5, -10.25, -10.25, -10.0, -10.0, -10.0, -10.0, -10.0, -9.75, -9.75, -9.75, -9.75, -9.75, -9.75, -9.75, -9.75, -9.75, -9.75, -9.5, -9.5, -9.5, -9.5, -9.5, -9.5, -9.5, -9.5, -9.5, -9.5, -9.5, -9.5, -9.5, -9.5, -9.5, -9.5, -9.5, -9.5, -9.5, -9.25, -9.25, -9.25, -9.25, -9.25, -9.25, -9.25, -9.25, -9.25, -9.25, -9.25, -9.25, -9.25, -9.25, -9.25, -9.25, -9.25, -9.25, -9.25, -9.25, -9.25, -9.25, -9.0, -9.0, -9.0, -9.0, -9.0, -9.0, -9.0, -9.0, -9.0, -9.0, -9.0, -9.0, -9.0, -9.0, -9.0, -9.0, -9.0, -9.0, -9.0, -9.0, -9.0, -9.0, -9.0, -9.0, -9.0, -9.0, -8.75, -8.75, -8.75, -8.75, -8.75, -8.75, -8.75, -8.75, -8.75, -8.75, -8.75, -8.75, -8.75, -8.75, -8.75, -8.75, -8.75, -8.75, -8.75, -8.75, -8.75, -8.75, -8.75, -8.75, -8.75, -8.75, -8.75, -8.75, -8.75, -8.75, -8.75, -8.75, -8.75, -8.75, -8.75, -8.75, -8.75, -8.5, -8.5, -8.5, -8.5, -8.5, -8.5, -8.5, -8.5, -8.5, -8.5, -8.5, -8.5, -8.5, -8.5, -8.5, -8.5, -8.5, -8.5, -8.5, -8.5, -8.5, -8.5, -8.5, -8.5, -8.5, -8.5, -8.5, -8.5, -8.5, -8.5, -8.5, -8.5, -8.5, -8.5, -8.5, -8.5, -8.25, -8.25, -8.25, -8.25, -8.25, -8.25, -8.25, -8.25, -8.25, -8.25, -8.25, -8.25, -8.25, -8.25, -8.25, -8.25, -8.25, -8.25, -8.25, -8.25, -8.25, -8.25, -8.25, -8.25, -8.25, -8.25, -8.25, -8.25, -8.25, -8.25, -8.25, -8.25, -8.25, -8.0, -8.0, -8.0, -8.0, -8.0, -8.0, -8.0, -8.0, -8.0, -8.0, -8.0, -8.0, -8.0, -8.0, -8.0, -8.0, -8.0, -8.0, -8.0, -8.0, -8.0, -8.0, -8.0, -8.0, -8.0, -7.75, -7.75, -7.75, -7.75, -7.75, -7.75, -7.75, -7.75, -7.75, -7.75, -7.75, -7.75, -7.75, -7.75, -7.75, -7.75, -7.75, -7.75, -7.75, -7.75, -7.75, -7.75, -7.75, -7.75, -7.75, -7.75, -7.5, -7.5, -7.5, -7.5, -7.5, -7.5, -7.5, -7.5, -7.5, -7.5, -7.5, -7.5, -7.5, -7.5, -7.5, -7.5, -7.5, -7.5, -7.5, -7.5, -7.5, -7.5, -7.5, -7.5, -7.5, -7.25, -7.25, -7.25, -7.25, -7.25, -7.25, -7.25, -7.25, -7.25, -7.25, -7.25, -7.25, -7.25, -7.25, -7.25, -7.25, -7.25, -7.25, -7.25, -7.25, -7.25, -7.25, -7.25, -7.0, -7.0, -7.0, -7.0, -7.0, -7.0, -7.0, -7.0, -7.0, -7.0, -7.0, -7.0, -7.0, -7.0, -7.0, -7.0, -7.0, -7.0, -7.0, -6.75, -6.75, -6.75, -6.75, -6.75, -6.75, -6.75, -6.75, -6.75, -6.75, -6.75, -6.75, -6.75, -6.75, -6.75, -6.75, -6.75, -6.75, -6.75, -6.75, -6.75, -6.75, -6.75, -6.5, -6.5, -6.5, -6.5, -6.5, -6.5, -6.5, -6.5, -6.5, -6.5, -6.5, -6.5, -6.5, -6.5, -6.5, -6.5, -6.5, -6.5, -6.5, -6.5, -6.5, -6.5, -6.5, -6.5, -6.5, -6.5, -6.5, -6.5, -6.5, -6.5, -6.25, -6.25, -6.25, -6.25, -6.25, -6.25, -6.25, -6.25, -6.25, -6.25, -6.25, -6.25, -6.25, -6.25, -6.25, -6.25, -6.25, -6.0, -6.0, -6.0, -6.0, -6.0, -6.0, -6.0, -6.0, -6.0, -6.0, -6.0, -5.75, -5.75, -5.75, -5.75, -5.75, -5.75, -5.75, -5.75, -5.75, -5.75, -5.5, -5.25, -5.0, -4.75, -4.5, -4.5, -4.25, -4.25, -4.0, -4.0, -3.75, -3.75, -3.5, -3.5, -3.25, -3.25, -3.25, -3.25, -3.0, -3.0, 2.0, 2.0, 2.0, 2.0, 2.0, 2.0, 2.0, 2.25, 2.25, 2.25, 2.25, 2.25, 2.25, 2.25, 2.25, 2.25, 2.25, 2.25, 2.25, 2.25, 2.25, 2.25, 2.25, 2.25, 2.25, 2.25, 2.25, 2.25, 2.25, 2.5, 2.5, 2.5, 2.5, 2.5, 2.5, 2.5, 2.5, 2.5, 2.5, 2.5, 2.5, 2.5, 2.5, 2.5, 2.5, 2.5, 2.5, 2.5, 2.5, 2.5, 2.5, 2.5, 2.5, 2.5, 2.5, 2.5, 2.5, 2.5, 2.5, 2.5, 2.5, 2.5, 2.5, 2.5, 2.5, 2.5, 2.5, 2.5, 2.5, 2.5, 2.5, 2.75, 2.75, 2.75, 2.75, 2.75, 2.75, 2.75, 2.75, 2.75, 2.75, 2.75, 2.75, 2.75, 2.75, 2.75, 2.75, 2.75, 2.75, 2.75, 2.75, 2.75, 2.75, 2.75, 2.75, 2.75, 2.75, 2.75, 2.75, 2.75, 2.75, 2.75, 2.75, 2.75, 2.75, 2.75, 2.75, 2.75, 2.75, 2.75, 2.75, 2.75, 2.75, 2.75, 2.75, 2.75, 2.75, 2.75, 2.75, 2.75, 2.75, 3.0, 3.0, 3.0, 3.0, 3.0, 3.0, 3.0, 3.0, 3.0, 3.0, 3.0, 3.0, 3.0, 3.0, 3.0, 3.0, 3.0, 3.0, 3.0, 3.0, 3.0, 3.0, 3.0, 3.0, 3.0, 3.0, 3.0, 3.0, 3.0, 3.0, 3.0, 3.0, 3.0, 3.0, 3.0, 3.0, 3.0, 3.0, 3.0, 3.0, 3.0, 3.0, 3.0, 3.0, 3.0, 3.0, 3.0, 3.25, 3.25, 3.25, 3.25, 3.25, 3.25, 3.25, 3.25, 3.25, 3.25, 3.25, 3.25, 3.25, 3.25, 3.25, 3.25, 3.25, 3.25, 3.25, 3.25, 3.25, 3.25, 3.25, 3.25, 3.25, 3.25, 3.25, 3.25, 3.25, 3.25, 3.25, 3.25, 3.25, 3.25, 3.25, 3.25, 3.25, 3.25, 3.25, 3.25, 3.25, 3.25, 3.25, 3.25, 3.25, 3.25, 3.25, 3.25, 3.25, 3.25, 3.25, 3.25, 3.25, 3.5, 3.5, 3.5, 3.5, 3.5, 3.5, 3.5, 3.5, 3.5, 3.5, 3.5, 3.5, 3.5, 3.5, 3.5, 3.5, 3.5, 3.5, 3.5, 3.5, 3.5, 3.5, 3.5, 3.5, 3.5, 3.5, 3.5, 3.5, 3.5, 3.5, 3.5, 3.5, 3.5, 3.5, 3.5, 3.5, 3.5, 3.5, 3.5, 3.5, 3.5, 3.5, 3.5, 3.5, 3.5, 3.5, 3.5, 3.5, 3.5, 3.5, 3.5, 3.5, 3.5, 3.5, 3.5, 3.5, 3.5, 3.75, 3.75, 3.75, 3.75, 3.75, 3.75, 3.75, 3.75, 3.75, 3.75, 3.75, 3.75, 3.75, 3.75, 3.75, 3.75, 3.75, 3.75, 3.75, 3.75, 3.75, 3.75, 3.75, 3.75, 3.75, 3.75, 3.75, 3.75, 3.75, 3.75, 3.75, 3.75, 3.75, 3.75, 3.75, 3.75, 3.75, 4.0, 4.0, 4.0, 4.0, 4.0, 4.0, 4.0, 4.0, 4.0, 4.0, 4.0, 4.0, 4.0, 4.0, 4.0, 4.0, 4.0, 4.0, 4.0, 4.0, 4.0, 4.0, 4.0, 4.0, 4.0, 4.0, 4.0, 4.0, 4.0, 4.0, 4.0, 4.0, 4.0, 4.0, 4.0, 4.0, 4.25, 4.25, 4.25, 4.25, 4.25, 4.25, 4.25, 4.25, 4.25, 4.25, 4.25, 4.25, 4.25, 4.25, 4.25, 4.25, 4.25, 4.25, 4.25, 4.25, 4.25, 4.25, 4.25, 4.25, 4.25, 4.25, 4.25, 4.25, 4.25, 4.25, 4.25, 4.25, 4.25, 4.25, 4.25, 4.25, 4.25, 4.25, 4.25, 4.25, 4.25, 4.25, 4.25, 4.5, 4.5, 4.5, 4.5, 4.5, 4.5, 4.5, 4.5, 4.5, 4.5, 4.5, 4.5, 4.5, 4.5, 4.5, 4.5, 4.5, 4.5, 4.5, 4.5, 4.5, 4.5, 4.5, 4.5, 4.5, 4.5, 4.5, 4.75, 4.75, 4.75, 4.75, 4.75, 4.75, 4.75, 4.75, 4.75, 4.75, 4.75, 4.75, 4.75, 4.75, 4.75, 4.75, 4.75, 4.75, 4.75, 4.75, 4.75, 4.75, 4.75, 4.75, 4.75, 4.75, 4.75, 4.75, 4.75, 5.0, 5.0, 5.0, 5.0, 5.0, 5.0, 5.0, 5.0, 5.0, 5.0, 5.0, 5.0, 5.0, 5.0, 5.0, 5.0, 5.0, 5.0, 5.0, 5.0, 5.0, 5.25, 5.25, 5.25, 5.25, 5.25, 5.25, 5.25, 5.25, 5.25, 5.25, 5.25, 5.25, 5.25, 5.25, 5.5, 5.5, 5.5, 5.5, 5.5, 5.5, 5.5, 5.5, 5.5, 5.5, 5.5, 5.5, 5.75, 5.75, 5.75, 5.75, 5.75, 5.75, 5.75, 5.75, 5.75, 5.75, 5.75, 5.75, 5.75, 5.75, 5.75, 5.75, 5.75, 6.0, 6.0, 6.0, 6.0, 6.0, 6.0, 6.0, 6.0, 6.0, 6.0, 6.0, 6.25, 6.25, 6.25, 6.25, 6.25, 6.25, 6.25, 6.25, 6.5, 6.5, 6.5, 6.5, 6.5, 6.5, 6.5, 6.5, 6.5, 6.75, 6.75, 6.75, 6.75, 7.0, 7.0, 7.0, 7.25, 7.25, 7.25, 7.25, 7.25, 7.25, 7.25, 7.5, 7.5, 8.0, 8.0, 8.0, 8.0, 8.0, 8.25, 8.25, 8.5, 8.5, 8.5, 8.75, 8.75, 8.75, 8.75, 8.75, 9.0, 9.0, 9.0, 9.0, 9.0, 9.0, 9.25, 9.25, 9.25, 9.25, 9.25, 9.25, 9.5, 9.5, 9.5, 9.5, 9.5, 9.5, 9.75, 9.75, 9.75, 10.0, 10.0, 10.0, 10.0, 10.25, 10.25, 10.5, 10.5, 10.5, 10.75, 10.75, 10.75, 10.75, 11.0, 11.0, 11.0, 11.0, 11.0, 11.25, 11.25, 11.25, 11.25, 11.25, 11.25, 11.25, 11.25, 11.25, 11.25, 11.5, 11.5, 11.5, 11.5, 11.5, 11.5, 11.5, 11.5, 11.5, 11.5, 11.5, 11.5, 11.5, 11.5, 11.5, 11.75, 11.75, 11.75, 11.75, 11.75, 11.75, 11.75, 11.75, 11.75, 11.75, 11.75, 11.75, 11.75, 11.75, 11.75, 11.75, 11.75, 11.75, 11.75, 11.75, 12.0, 12.0, 12.0, 12.0, 12.0, 12.0, 12.0, 12.0, 12.0, 12.0, 12.0, 12.0, 12.0, 12.0, 12.0, 12.0, 12.0, 12.0, 12.0, 12.0, 12.0, 12.0, 12.0, 12.0, 12.0, 12.0, 12.0, 12.25, 12.25, 12.25, 12.25, 12.25, 12.25, 12.25, 12.25, 12.25, 12.25, 12.25, 12.25, 12.25, 12.25, 12.25, 12.25, 12.5, 12.5, 12.5, 12.5, 12.5, 12.5, 12.5, 12.5, 12.5, 12.5, 12.5, 12.5, 12.5, 12.75, 12.75, 12.75, 12.75, 12.75, 12.75, 12.75, 12.75, 12.75, 12.75, 13.0, 13.0, 13.0, 13.0, 13.0, 13.0, 13.0, 13.0, 13.0, 13.0, 13.0, 13.0, 13.0, 13.0, 13.0, 13.0, 13.0, 13.0, 13.0, 13.0, 13.0, 13.0, 13.0, 13.25, 13.25, 13.25, 13.25, 13.25, 13.25, 13.25, 13.25, 13.25, 13.25, 13.25, 13.25, 13.25, 13.25, 13.25, 13.25, 13.25, 13.25, 13.25, 13.5, 13.5, 13.5, 13.5, 13.5, 13.5, 13.5, 13.5, 13.5, 13.5, 13.75, 13.75, 13.75, 13.75, 13.75, 13.75, 13.75, 13.75, 13.75, 14.0, 14.0, 14.0, 14.0, 14.5, 14.75, 15.5, 15.75, 16.0, 19.25, 19.25, 19.25, 19.5, 19.5, 19.75, 22.25, 22.25, 22.25, 22.5, 22.5, 22.5, 22.75, 22.75, 22.75, 22.75, 23.0, 23.0, 23.0, 23.25, 23.25, 23.25, 23.5, 23.5, 23.5, 23.5, 23.5, 23.5, 23.75, 23.75, 23.75, 23.75, 23.75, 23.75, 23.75, 23.75, 23.75, 23.75, 23.75, 24.0, 24.0, 24.0, 24.0, 24.0, 24.0, 24.0, 24.25, 24.25, 24.5], "Y"=[46.5, 46.5, 46.5, 2.75, 0.5, 2.75, 17.0, 0.75, 17.25, -6.5, -2.25, -1.75, 0.5, 0.75, 1.0, 3.75, -6.5, 0.75, 4.0, 4.25, 17.25, 21.5, -6.75, -6.5, -1.75, 17.25, 21.5, 22.25, -6.75, 21.75, 22.0, -6.5, 11.25, 22.0, 10.5, 10.75, 11.0, 11.5, 11.75, -6.0, 3.75, 8.25, -1.0, 8.25, -1.25, -1.0, -7.0, -1.25, 2.75, 3.0, 3.5, -10.75, -10.5, -10.0, -9.5, -9.25, -8.25, -6.75, -1.25, 3.0, 3.25, -20.5, -15.5, -15.25, -14.75, -10.5, -10.25, -10.0, -9.75, -9.25, -9.0, -8.75, -8.25, -8.0, -7.75, -7.5, -1.0, 0.5, 1.5, 2.75, -20.25, -18.25, -17.75, -17.5, -17.0, -15.75, -15.5, -10.75, -10.25, -9.5, -9.0, -8.75, -8.25, -8.0, -7.75, 0.75, 1.0, 1.25, 2.25, 3.5, 7.25, 7.5, -19.0, -17.5, -17.25, -10.5, -10.25, -10.0, -9.25, -9.0, -8.75, -8.25, -8.0, -7.25, -7.0, -6.75, -4.75, -4.5, -4.25, 0.75, 1.0, 1.25, 1.75, 2.25, 2.5, 2.75, 3.5, 7.5, -17.5, -12.75, -12.0, -11.75, -10.5, -9.75, -9.5, -9.25, -9.0, -8.75, -8.5, -8.25, -8.0, -7.75, -7.5, -7.0, -6.75, -4.75, -4.5, -3.75, -3.25, -3.0, -1.5, -0.5, -0.25, 0.0, 0.25, 1.75, 2.5, 2.75, 4.25, 4.75, 5.5, 5.75, 6.25, 7.5, 7.75, -13.25, -13.0, -12.75, -12.0, -11.75, -8.25, -8.0, -7.0, -6.75, -5.5, -5.0, -4.75, -4.5, -4.0, -3.75, -3.25, -3.0, -2.75, -2.0, -1.75, -1.5, -1.0, -0.5, -0.25, 0.0, 0.25, 0.5, 0.75, 1.75, 2.0, 4.0, 4.25, 4.75, 5.75, 6.0, 6.25, -17.5, -12.75, -12.0, -11.5, -10.25, -8.25, -8.0, -7.75, -5.5, -4.75, -4.0, -3.75, -3.5, -3.25, -3.0, -2.75, -2.5, -2.25, -2.0, -1.75, -1.5, -0.75, -0.5, -0.25, 0.0, 0.25, 0.5, 2.25, 4.5, 4.75, 5.75, 6.0, 6.25, -13.5, -13.25, -13.0, -7.75, -5.75, -5.5, -5.25, -5.0, -4.75, -4.5, -3.75, -3.5, -3.25, -2.25, -2.0, -1.75, -1.5, -1.25, -0.75, -0.5, -0.25, 0.0, 0.25, 0.5, 0.75, -13.25, -12.5, -6.0, -5.75, -5.25, -5.0, -4.75, -4.5, -4.25, -3.25, -2.5, -2.25, -2.0, -1.75, -1.5, -1.25, -0.75, -0.5, -0.25, 0.0, 0.25, 0.5, 4.0, 4.25, 7.75, 8.0, -14.0, -13.25, -13.0, -8.0, -5.25, -5.0, -4.75, -3.75, -3.0, -2.0, -1.75, -1.5, -1.25, -0.5, -0.25, 0.25, 0.5, 0.75, 1.0, 1.25, 1.5, 2.25, 2.5, 3.75, 9.25, -7.75, -7.25, -7.0, -6.75, -6.5, -6.25, -6.0, -5.75, -5.5, -5.25, -5.0, -3.5, -1.75, -1.5, -1.25, -0.5, -0.25, 1.0, 1.25, 1.75, 2.5, 5.75, 8.5, -9.0, -8.0, -7.75, -7.0, -6.75, -6.5, -5.5, -5.25, -5.0, -2.0, -1.75, 1.25, 1.5, 2.5, 4.0, 4.25, 4.5, 6.0, 8.5, -9.25, -9.0, -7.5, -7.25, -5.75, -5.5, -2.75, -2.5, -1.0, -0.75, -0.5, -0.25, 0.0, 1.0, 1.25, 1.75, 2.75, 3.0, 4.5, 4.75, 5.75, 6.0, 6.25, -20.0, -8.0, -7.5, -7.25, -4.5, -4.25, -3.25, -3.0, -2.75, -2.5, -1.25, -1.0, -0.75, -0.5, 2.25, 2.5, 2.75, 3.0, 3.25, 3.5, 3.75, 4.0, 4.25, 4.5, 4.75, 5.0, 5.25, 5.5, 5.75, 6.0, -20.25, -20.0, -14.0, -13.75, -8.0, -7.75, -7.25, -5.0, -4.75, -4.5, -3.5, -3.25, -3.0, -2.0, -1.75, -1.5, 3.0, -20.0, -14.0, -13.75, -8.0, -7.75, -7.5, -7.25, -5.0, -2.0, -1.75, -1.5, -20.5, -20.25, -14.25, -8.0, -7.75, -7.5, -2.0, -1.75, -1.5, 3.0, 3.0, 3.0, 3.0, 3.0, 3.0, 20.75, 3.0, 20.75, 3.0, 20.75, 3.0, 20.75, 3.0, 20.75, 3.0, 21.0, 22.0, 22.25, 3.0, 22.25, -8.25, -8.0, -7.25, -2.75, -2.5, -2.25, -2.0, -20.5, -14.5, -14.25, -8.5, -8.25, -8.0, -7.75, -7.25, -4.5, -4.0, -3.5, -3.25, -3.0, -2.5, -2.25, -2.0, -1.5, -1.25, -1.0, 4.75, 6.0, 6.25, -20.5, -20.25, -14.25, -8.25, -8.0, -7.75, -5.0, -4.5, -4.25, -4.0, -3.75, -3.5, -3.25, -3.0, -2.75, -2.5, -2.25, -2.0, -1.75, -1.5, -1.25, -1.0, -0.75, 0.75, 1.75, 2.0, 2.25, 2.5, 2.75, 3.0, 3.25, 3.5, 3.75, 4.0, 5.0, 5.25, 5.5, 5.75, 6.25, 6.5, 6.75, 7.0, -20.5, -20.25, -14.25, -8.25, -7.75, -4.75, -4.5, -4.25, -4.0, -3.75, -3.5, -3.25, -3.0, -2.75, -2.5, -2.0, -1.75, -1.5, -1.25, -1.0, -0.75, -0.5, 0.25, 0.5, 0.75, 1.0, 1.25, 1.5, 1.75, 2.0, 2.25, 2.5, 2.75, 3.25, 3.5, 3.75, 4.0, 4.25, 4.5, 4.75, 5.0, 5.25, 5.5, 5.75, 6.0, 6.25, 6.5, 6.75, 7.0, 7.25, -20.25, -7.75, -5.25, -4.5, -4.25, -4.0, -3.75, -3.5, -3.25, -2.75, -2.5, -2.25, -2.0, -1.75, -1.5, -1.25, -1.0, -0.75, -0.5, -0.25, 0.0, 0.25, 0.5, 0.75, 1.0, 1.25, 1.5, 1.75, 2.0, 2.25, 2.5, 2.75, 4.25, 4.5, 4.75, 5.0, 5.25, 5.5, 5.75, 6.0, 6.25, 6.5, 6.75, 7.0, 7.5, 9.5, 10.75, -20.5, -7.5, -6.75, -6.0, -5.75, -5.0, -4.75, -4.5, -4.25, -4.0, -3.25, -3.0, -2.75, -2.5, -2.0, -1.75, -1.5, -1.25, -1.0, -0.75, -0.5, -0.25, 0.0, 0.25, 0.5, 0.75, 1.0, 1.25, 1.5, 1.75, 2.0, 2.25, 2.5, 2.75, 3.0, 4.5, 4.75, 5.0, 5.25, 5.5, 5.75, 6.0, 6.25, 6.5, 6.75, 7.0, 7.25, 9.25, 9.5, 10.75, 11.0, 12.25, 12.75, -7.75, -7.5, -6.75, -6.5, -5.75, -5.5, -5.25, -4.75, -4.25, -4.0, -3.5, -3.0, -2.75, -2.25, -2.0, -1.75, -1.5, -1.25, -1.0, -0.75, -0.5, -0.25, 0.0, 0.25, 0.5, 0.75, 1.0, 1.25, 1.5, 1.75, 2.0, 2.25, 2.5, 2.75, 3.0, 4.75, 5.0, 5.25, 5.5, 5.75, 6.0, 6.5, 6.75, 7.0, 8.75, 9.0, 9.25, 10.25, 10.75, 11.0, 11.25, 12.25, 12.5, 12.75, 13.0, 13.25, 13.75, -8.75, -7.5, -6.5, -6.25, -5.5, -5.0, -4.75, -4.5, -4.25, -4.0, -2.25, -1.75, -1.5, -1.25, -1.0, -0.75, -0.5, -0.25, 0.0, 0.25, 0.5, 1.0, 1.25, 1.5, 1.75, 2.0, 2.25, 2.5, 2.75, 3.0, 3.25, 9.75, 11.0, 11.25, 12.25, 12.5, 13.0, -8.5, -7.5, -6.75, -6.5, -5.5, -5.25, -4.25, -4.0, -3.25, -3.0, -2.75, -2.5, -2.25, -1.75, -1.5, -1.25, -1.0, -0.75, -0.5, -0.25, 0.0, 0.25, 0.5, 0.75, 1.0, 1.25, 1.5, 1.75, 2.0, 2.25, 2.5, 2.75, 3.0, 12.5, 13.0, 13.25, -9.75, -9.5, -9.25, -8.75, -8.5, -8.25, -7.75, -7.5, -7.25, -7.0, -6.75, -6.5, -6.25, -6.0, -5.75, -5.0, -4.25, -3.0, -2.75, -2.5, -2.25, -1.75, -1.5, 0.0, 0.25, 0.5, 0.75, 1.0, 1.25, 1.5, 1.75, 2.0, 2.5, 2.75, 3.0, 3.25, 11.0, 11.25, 11.5, 12.0, 12.25, 12.5, 13.0, -10.0, -9.0, -8.75, -8.5, -8.25, -7.5, -7.25, -6.5, -6.0, -5.75, -4.5, -4.25, -4.0, -3.0, 0.25, 0.5, 0.75, 1.0, 2.5, 2.75, 3.0, 3.5, 11.5, 11.75, 12.0, 12.25, 12.75, -11.25, -10.75, -10.0, -9.5, -9.25, -9.0, -8.75, -8.0, -7.25, -7.0, -6.5, -6.25, -6.0, -5.75, -5.5, -4.75, -4.5, -4.25, -4.0, -3.75, 2.25, 2.5, 2.75, 3.0, 3.5, 6.75, 11.25, 11.5, 12.0, -12.25, -9.0, -8.75, -6.5, -6.25, -6.0, -5.75, -5.5, -5.25, -5.0, -4.75, -4.25, -4.0, -3.75, -3.5, 1.25, 2.5, 2.75, 3.25, 6.75, 12.0, -9.0, -8.75, -8.5, -7.0, -5.75, -5.5, -4.25, -3.5, -3.25, -3.0, -0.75, 2.0, 2.25, 12.0, -10.75, -9.0, -8.25, -3.25, -3.0, 2.0, 2.25, 2.5, 4.25, 5.75, 12.0, 13.0, -9.0, -3.5, 1.0, 1.25, 1.5, 1.75, 2.25, 2.5, 2.75, 3.25, 5.5, 5.75, 8.25, 8.5, 8.75, 9.0, 9.25, -9.0, -8.75, 1.5, 1.75, 3.25, 3.5, 5.5, 5.75, 6.25, 8.25, 9.0, -9.0, -8.75, 1.75, 3.25, 3.75, 5.75, 9.0, 9.5, -17.25, 1.5, 1.75, 3.25, 4.75, 5.5, 6.0, 6.25, 6.75, 4.5, 4.75, 5.5, 6.25, 4.5, 4.75, 5.75, 4.5, 6.25, 8.75, 9.0, 10.25, 10.5, 17.0, 4.0, 17.0, 1.5, 6.75, 10.75, 11.0, 17.5, 0.0, 17.5, 3.25, 17.25, 17.5, 0.25, 3.0, 3.25, 11.25, 11.5, -0.5, 6.75, 11.25, 11.5, 12.25, 35.5, -11.25, 12.0, 12.25, 12.75, 17.0, 35.5, -13.0, -12.25, -10.75, 12.0, 12.25, 17.0, 16.5, 16.75, 28.5, 16.25, 16.5, 28.25, 28.75, 28.0, 28.5, 2.25, 28.0, 28.25, 2.0, 2.5, 3.25, 8.0, 2.75, 3.25, 8.0, 8.25, 15.75, -7.75, -7.5, -5.25, -4.75, -2.25, 5.25, 8.0, 8.25, 15.25, 15.5, -9.25, -7.25, -4.75, -3.5, -3.0, -2.5, 2.5, 4.0, 4.25, 4.5, 4.75, 7.0, 7.75, 8.75, 9.0, -7.75, 1.0, 1.5, 2.25, 2.5, 2.75, 3.0, 3.25, 3.5, 3.75, 4.0, 4.25, 4.5, 4.75, 5.0, 5.25, 6.25, 8.0, 10.5, 28.75, -11.25, -7.25, 1.5, 1.75, 2.0, 2.25, 2.5, 2.75, 3.0, 3.25, 3.5, 3.75, 4.0, 4.25, 4.75, 5.0, 5.25, 5.5, 5.75, 6.0, 6.25, 6.5, 7.0, 7.25, 7.5, 7.75, 14.25, 1.75, 2.0, 2.5, 3.25, 3.75, 4.0, 5.75, 6.0, 6.25, 6.5, 6.75, 7.5, 9.25, 13.0, 13.25, 14.0, 1.75, 2.0, 2.5, 3.0, 3.25, 3.5, 6.0, 8.0, 8.25, 9.25, 10.25, 13.5, 13.75, -1.75, -1.5, -1.25, 3.25, 3.5, 4.0, 7.0, 8.0, 9.0, 13.0, -9.5, -5.0, -4.5, -4.25, -4.0, -3.75, -2.0, -1.75, -1.5, -1.25, -1.0, -0.75, -0.5, -0.25, 0.0, 0.25, 6.0, 7.5, 8.75, 9.5, 10.25, 12.25, 12.5, -5.5, -5.25, -5.0, -4.75, -4.5, -4.0, -3.75, -3.5, -2.0, -1.75, -1.0, -0.25, 0.25, 1.0, 1.25, 1.5, 7.5, 10.5, 10.75, -6.75, -6.5, -6.25, -6.0, -5.75, -5.5, 1.0, 1.25, 5.75, 10.5, -7.5, -7.25, -7.0, -6.75, -6.5, -3.5, -3.25, 1.25, 10.25, -7.0, -6.75, -3.5, 9.0, -4.0, -4.25, 17.25, 17.0, 17.0, 3.0, 3.25, 16.5, 16.5, 16.75, 3.0, 13.0, 13.25, 13.5, 13.75, 14.0, 14.25, 14.5, 14.75, 15.0, 15.25, 15.25, 15.5, 15.75, 16.0, 16.25, 16.5, 4.75, 5.0, 10.25, 16.75, 17.0, 17.25, 4.25, 4.5, 4.75, 5.0, 5.25, 5.5, 5.75, 6.0, 6.25, 6.5, 10.25, 4.25, 6.5, 6.75, 7.0, 7.25, 7.5, 7.75, 8.0, 10.0, 10.0]}, {"Y"=[-1.75], "Y"=[8.75]}, {"Y"=[-23.75, -23.5, -23.5, -22.0, -21.75, -17.5, -13.0, -13.0, -12.75, -12.5, -12.25, -11.5, -10.75, -10.75, -10.5, -10.5, -10.5, -10.5, -10.25, -10.25, -10.25, -10.0, -9.75, -9.5, -9.5, -9.5, -9.25, -9.25, -9.0, -9.0, -9.0, -9.0, -8.75, -8.75, -8.75, -8.75, -8.75, -8.75, -8.75, -8.75, -8.75, -8.5, -8.5, -8.5, -8.5, -8.5, -8.5, -8.5, -8.25, -8.25, -8.25, -8.25, -8.25, -8.25, -8.25, -8.25, -8.25, -8.25, -8.25, -8.0, -8.0, -8.0, -8.0, -7.75, -7.75, -7.75, -7.75, -7.75, -7.75, -7.75, -7.75, -7.75, -7.5, -7.5, -7.5, -7.5, -7.5, -7.5, -7.5, -7.5, -7.5, -7.5, -7.5, -7.5, -7.25, -7.25, -7.25, -7.25, -7.25, -7.25, -7.25, -7.25, -7.25, -7.25, -7.25, -7.25, -7.25, -7.25, -7.0, -7.0, -7.0, -7.0, -7.0, -7.0, -7.0, -7.0, -7.0, -7.0, -6.75, -6.75, -6.75, -6.75, -6.75, -6.75, -6.75, -6.75, -6.75, -6.75, -6.75, -6.5, -6.5, -6.5, -6.5, -6.5, -6.25, -6.25, -6.25, -6.25, -6.25, -6.25, -6.25, -6.25, -6.25, -6.25, -6.25, -6.25, -6.0, -6.0, -5.75, -5.75, -5.75, -5.75, -5.75, -5.75, -5.75, -5.75, -5.75, -5.75, -5.75, -5.75, -5.75, -5.75, -5.75, -2.25, -2.25, -2.25, -2.25, -2.25, -2.25, -2.25, -2.25, -2.25, -2.25, -2.25, -2.25, -2.25, -2.25, -2.25, -2.25, -2.25, -2.25, -2.0, -2.0, -2.0, -2.0, -2.0, -2.0, -2.0, -2.0, -2.0, -2.0, -2.0, -2.0, -2.0, -2.0, -2.0, -2.0, -2.0, -2.0, -2.0, -2.0, -2.0, -2.0, -2.0, -2.0, -1.75, -1.75, -1.75, -1.75, -1.75, -1.75, -1.75, -1.75, -1.75, -1.75, -1.75, -1.75, -1.75, -1.75, -1.75, -1.75, -1.75, -1.5, -1.5, -1.5, -1.5, -1.5, -1.5, -1.5, -1.5, -1.5, -1.5, -1.5, -1.5, -1.5, -1.25, -1.25, 1.75, 1.75, 1.75, 1.75, 1.75, 1.75, 1.75, 1.75, 1.75, 1.75, 1.75, 1.75, 1.75, 2.0, 2.0, 2.0, 2.0, 2.0, 2.0, 2.0, 2.0, 2.0, 2.0, 2.25, 2.25, 2.5, 2.5, 2.5, 2.5, 2.5, 2.5, 2.75, 2.75, 2.75, 2.75, 2.75, 2.75, 2.75, 2.75, 2.75, 3.0, 3.0, 3.0, 3.0, 3.0, 3.0, 3.0, 3.0, 3.25, 3.25, 3.25, 3.25, 3.25, 3.25, 3.25, 3.25, 3.5, 3.5, 3.5, 3.5, 3.5, 3.75, 4.0, 4.0, 4.0, 4.0, 4.25, 4.25, 4.25, 4.5, 4.5, 4.5, 4.5, 4.75, 4.75, 4.75, 5.0, 5.0, 5.5, 6.5, 7.0, 7.0, 7.25, 7.5, 7.5, 7.75, 7.75, 8.0, 8.25, 8.5, 8.75, 8.75, 10.5, 10.75, 11.0, 11.0, 11.0, 11.0, 11.0, 11.0, 11.25, 11.25, 11.25, 11.25, 11.25, 11.25, 11.25, 11.25, 11.5, 11.5, 11.5, 11.5, 11.5, 11.5, 11.5, 11.5, 11.5, 11.5, 11.5, 11.5, 11.75, 11.75, 11.75, 11.75, 11.75, 12.0, 12.0, 12.0, 12.0, 12.0, 12.0, 12.0, 12.25, 12.25, 12.5, 12.75, 13.5, 13.5, 13.5, 13.5, 13.5, -2.25, -2.25, -1.75], "Y"=[24.75, 24.75, 25.0, 24.75, 24.75, 15.25, 1.0, 4.5, 20.0, 19.75, 0.5, 14.25, 14.25, 14.5, 6.0, 14.5, 14.75, 15.5, 14.75, 15.0, 15.25, 9.5, 3.5, -3.0, 3.0, 3.25, 8.25, 16.75, 0.5, 1.5, 8.25, 12.25, 1.0, 1.25, 1.5, 2.0, 2.25, 6.0, 8.0, 8.5, 12.75, -11.5, -5.75, 1.0, 2.25, 3.0, 9.0, 12.75, -13.25, -11.0, -4.5, -1.25, 3.0, 3.25, 4.0, 6.5, 8.75, 9.0, 9.25, -15.0, 8.75, 9.0, 9.25, -13.5, -8.0, -6.25, -3.0, -2.75, 1.75, 2.0, 2.25, 9.75, -11.5, -4.5, -2.75, -1.0, -0.75, 0.0, 2.0, 2.75, 3.0, 7.0, 7.25, 7.5, -14.25, -11.5, -8.5, -8.0, -4.75, -4.25, -3.25, -3.0, -0.75, 0.25, 0.75, 2.75, 3.0, 7.75, -14.75, -14.5, -11.5, -8.25, -1.5, -1.25, 1.0, 8.0, 8.25, 10.5, -11.75, 0.25, 0.5, 0.75, 1.5, 2.0, 2.25, 2.5, 6.5, 6.75, 8.25, -19.0, 0.25, 0.5, 0.75, 6.25, -5.75, -2.5, -0.25, 0.0, 0.25, 0.5, 0.75, 1.0, 1.25, 1.5, 1.75, 2.0, 5.0, 6.25, -12.25, -10.0, -5.25, -4.25, -4.0, -3.0, -0.75, -0.5, -0.25, 2.0, 2.25, 2.5, 3.75, 4.0, 5.0, -3.25, -3.0, -2.5, -2.25, 3.0, 3.25, 3.5, 3.75, 4.0, 4.25, 4.5, 4.75, 5.0, 5.25, 5.5, 6.0, 6.5, 7.25, -12.75, -10.75, -9.25, -9.0, -8.0, -7.0, -6.25, -5.5, -5.0, -4.5, -4.0, -3.5, -3.25, -3.0, -2.75, -2.5, -2.25, 3.0, 3.25, 3.5, 3.75, 4.25, 4.5, 15.25, -15.5, -12.75, -10.75, 3.5, 3.75, 4.0, 4.25, 4.5, 4.75, 5.0, 5.25, 5.75, 6.25, 6.75, 7.25, 8.0, 15.25, -12.75, -10.75, -9.25, -8.0, -7.0, -6.25, -5.75, -5.25, -5.0, -4.5, -4.25, -3.75, -3.5, -15.75, -12.75, 3.25, 3.5, 3.75, 4.0, 4.25, 4.5, 4.75, 5.0, 5.25, 5.75, 6.25, 6.75, 7.25, -13.0, -4.5, -4.25, -3.75, 6.0, 6.25, 6.75, 7.25, 8.0, 8.75, 3.75, 10.0, 4.25, 4.5, 4.75, 6.0, 7.75, 11.25, -7.0, -6.0, -5.25, 7.5, 7.75, 8.5, 9.5, 9.75, 12.75, -12.5, -12.25, -6.75, -6.0, -5.75, 8.25, 8.5, 9.25, -10.5, -8.75, -8.5, 9.0, 10.25, 10.5, 12.5, 15.25, -15.5, -15.0, -10.5, -8.75, 10.5, -3.25, -12.5, -12.25, -10.0, -6.25, -8.0, -5.5, 2.25, -9.75, -8.0, -6.25, -4.75, -12.75, -5.25, -5.0, -12.5, 1.5, 1.5, 3.75, 1.25, 5.5, 5.5, 3.5, 5.75, 1.75, 3.5, 3.5, 8.0, 3.75, -1.5, 8.25, 3.5, 3.0, 2.5, 4.0, 4.25, 4.75, 5.25, 9.25, -5.5, -3.75, -2.0, 1.75, 3.25, 3.5, 8.5, 10.75, -7.5, -5.25, 1.25, 3.0, 3.25, 3.5, 8.0, 8.5, 9.5, 9.75, 10.25, 10.5, -7.5, -5.25, 1.75, 2.0, 7.5, -4.5, -4.25, -3.75, 6.75, 8.0, 13.75, 14.0, -3.5, 13.5, 12.25, 12.5, -0.75, -0.5, -0.25, 0.0, 0.25, 8.75, 12.75, 8.75]}, {"Y"=[0.85, 0.95, 0.95, 0.6, 0.6, 0.85, 0.85, -0.85, -0.85, -0.95, -0.95, -0.6, -0.6, -0.85, -0.6, -0.6, -0.85, -0.85, 0.85, 0.85], "Y"=[-0.6, -0.6, -1.4, -1.4, -0.6, -0.6, 2.4, 2.4, -0.6, -0.6, -1.4, -1.4, -0.6, -0.6, -0.6, -1.4, -1.4, -1.6, -1.6, -1.4]}]
  out "rd":dbl
  out "bb":dbl
  out "aa":dbl
  out "xx":dbl[](array[numeric])
  out "yy":dbl[](array[numeric])
  in  "a":dbl=0.7
  out "stack":bool=TRUE
  out "track_shift":dbl[][](array[numeric])
  out "R":dbl[](array[numeric])
  out "theta":dbl[](array[numeric])
  out "RXY":dbl[](array[numeric])=[73.97207949000635, 12.402968176654849, 69.25942811748455]
  out "lw":dbl=0.4
  out "tic":u32=313769281
  out "reverse":bool
  out "map_track":dbl[][](array[numeric])=[[-0.6687401515638595, -3.551350516814976], [-1.1601880006125764, -3.4580278333550782], [-1.6512488590649952, -3.3629580799680854], [-2.1418835557610314, -3.265964418362822], [-2.6320529195405924, -3.1668700102479344], [-3.12171777924361, -3.0654980173321356], [-3.6108389637099756, -2.961671601324125], [-4.250355012057505, -2.8217269001890974], [-4.733554194697693, -2.693195492254268]]
  out "track":dbl[][](array[numeric])=[[-0.6687401515638595, -3.551350516814976], [-1.1601880006125764, -3.4580278333550782], [-1.6512488590649952, -3.3629580799680854], [-2.1418835557610314, -3.265964418362822], [-2.6320529195405924, -3.1668700102479344], [-3.12171777924361, -3.0654980173321356], [-3.6108389637099756, -2.961671601324125], [-4.250355012057505, -2.8217269001890974], [-4.733554194697693, -2.693195492254268], [-5.215089885143842, -2.558342659026822], [-5.693483406062963, -2.4115492889016945], [-6.167256080122039, -2.24719627027381], [-6.634929229988109, -2.059664491538052], [-7.095024178328142, -1.8433348410893422], [-7.546062247809149, -1.5925882073226139], [-7.98656476109811, -1.301805478632852], [-8.415053040862054, -0.9653675434148765], [-8.830048409767974, -0.5776552900636165], [-9.230072190482858, -0.133049606974057], [-9.61364570567371, 0.3740686174589265], [-9.97929027800753, 0.949318494840405], [-10.386059580111024, 1.7242186788508236], [-10.53357405922493, 2.2019628347040774], [-10.66851200140239, 2.6835902739278463], [-10.772007434080049, 3.1749262819640283], [-10.825194384694537, 3.6817961442544633], [-10.809206880682517, 4.210025146240928], [-10.705178949480636, 4.765438573365376], [-10.494244618525542, 5.353861711069529], [-10.157537915253862, 5.981119844795286], [-9.676192867102248, 6.653038259984428], [-8.946295802610212, 7.461572105302583], [-8.539313408094966, 7.752602995705581], [-8.110420661696207, 8.015244834208291], [-7.660232732059987, 8.25029468946181], [-7.189364787832295, 8.458549630117131], [-6.698431997659123, 8.640806724825243], [-6.188049530186491, 8.797863042237132], [-5.658832554060375, 8.930515651003796], [-5.11139623792681, 9.039561619776274], [-4.546355750431802, 9.12579801720561], [-3.9643262602213256, 9.190021911942688], [-3.3659229359414162, 9.233030372638604], [-2.7517609462380523, 9.25562046794435], [-2.122455459757251, 9.258589266510917], [-1.4786216451450183, 9.242733836989292], [-0.8208746710473604, 9.208851248030518], [-0.1498297061102689, 9.157738568285591], [0.5338980810202378, 9.090192866405497], [1.229693521698167, 9.007011211041284], [1.9369414472775146, 8.908990670843883], [2.6550266891122614, 8.796928314464337], [3.383334078556428, 8.671621210553642], [4.121248446963983, 8.53386642776284], [4.868154625688948, 8.384461034742866], [5.623437446085289, 8.224202100144819], [6.386481739507029, 8.053886692619635], [7.156672337308164, 7.874311880818305], [7.838146127104554, 7.70968069378327], [8.321781606815595, 7.582803343212244], [8.805290536895978, 7.45544776805299], [9.287663918083021, 7.323801011645703], [9.76789275111402, 7.18405011733063], [10.244968036726283, 7.032382128447967], [10.717880775657084, 6.864984088337955], [11.18562196864372, 6.678043040340844], [11.647182616423507, 6.4677460277968315], [12.101553719733744, 6.230280094046104], [12.547726279311707, 5.961832282428966], [12.984691295894704, 5.658589636285609], [13.411439770220039, 5.3167391989562285], [13.939637565704926, 4.818324597988705], [14.177469695018669, 4.377621822306417], [14.370305638929839, 3.9092831916317614], [14.522185803389362, 3.415790251277338], [14.637150594348116, 2.8996245465557346], [14.719240417757044, 2.363267622779441], [14.77249567956704, 1.8092010252611073], [14.800956785728996, 1.2399062993133256], [14.808664142193827, 0.6578649902486369], [14.799658154912459, 0.06555864337958095], [14.777979229835777, -0.5345311959811911]]
  out "xyhc":T2={"c_idx"=71, "xc"=-91.48037348905598, "yc"=-434.27857700428615, "hc"=-0.4484199308552679, "xc_path"=12.43286899562552}
  in  "margin":dbl
  out "vr":dbl=0.75
  out "vf":dbl=3.5
  out "vw":dbl=0.9025
  out "ymax":dbl=12.0
  out "ymin":dbl=-6.0
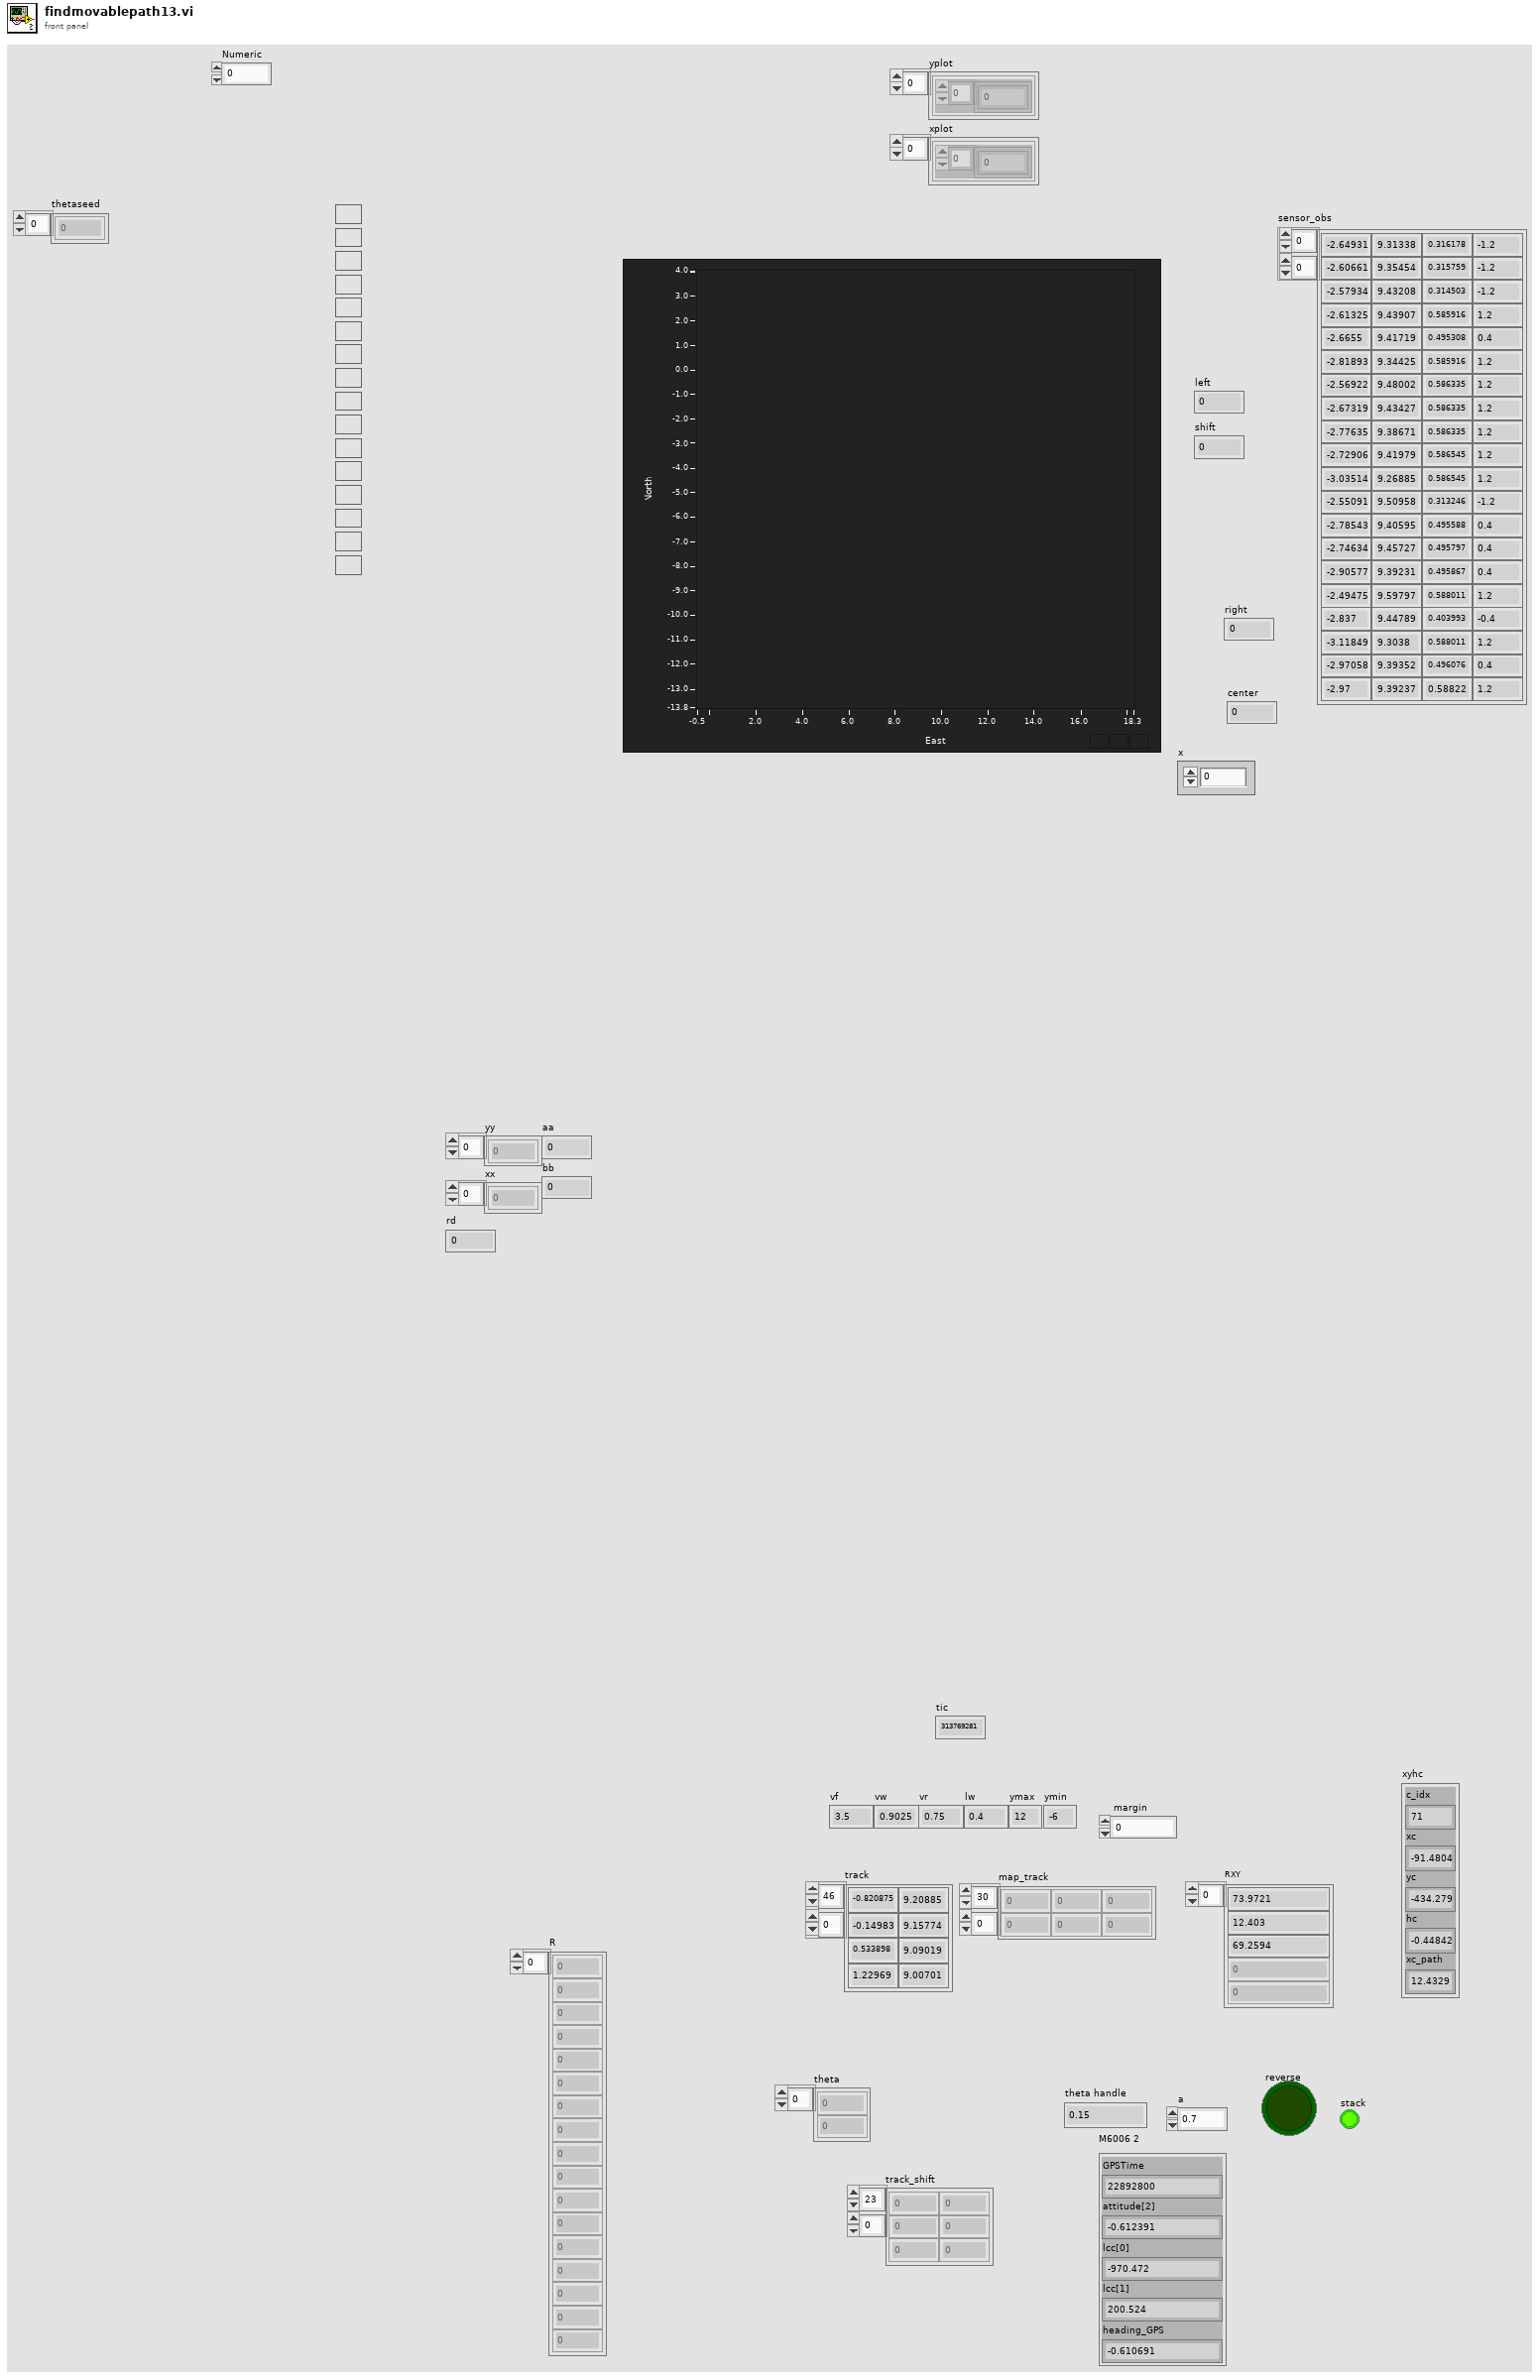
[diagram p1: front panel]
types:
  T1 = cluster{"GPSTime":dbl, "attitude[2]":dbl, "lcc[0]":dbl, "lcc[1]":dbl, "heading_GPS":dbl}
  T2 = cluster{"c_idx":i32, "xc":dbl, "yc":dbl, "hc":dbl, "xc_path":dbl}
  T3 = cluster{"Steer_input":dbl, "Steer_output":dbl, "VS_des":dbl, "VS_can":dbl, "heading":dbl, "auto":bool, "run":bool, "x":dbl, "y":dbl}
  T4 = cluster{"idx":i32, "x":dbl, "y":dbl, "h":dbl, "x_path":dbl}
  T5 = typedef "NI_Matrix.lvlib/RealMatrix.ctl" = dbl[][]
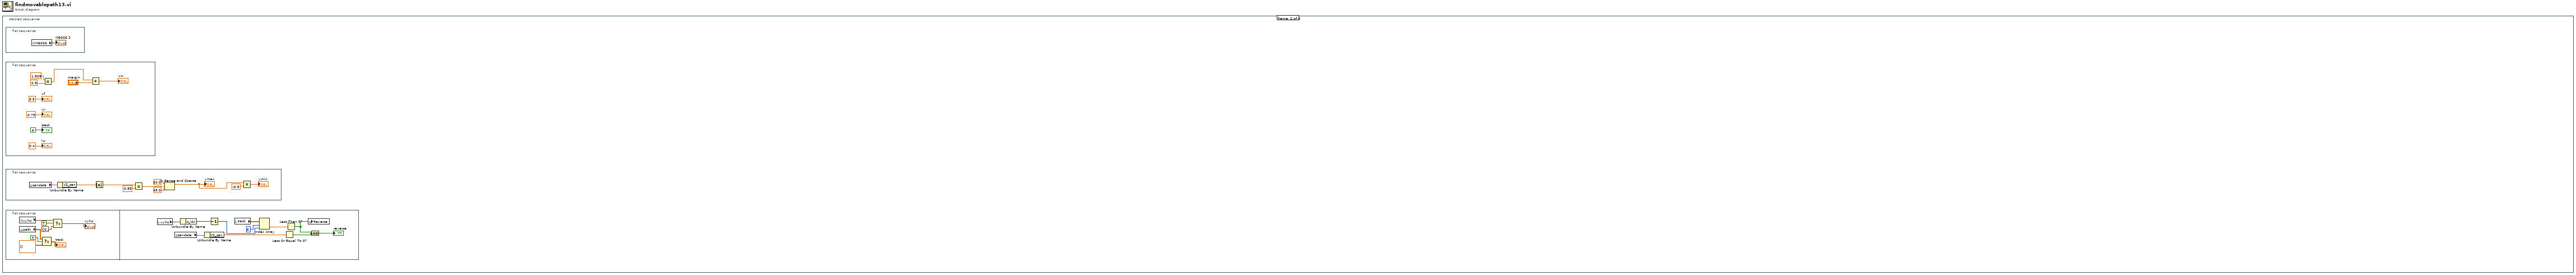
[diagram p0: block diagram]
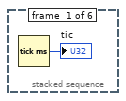
[diagram p2: hidden frame]
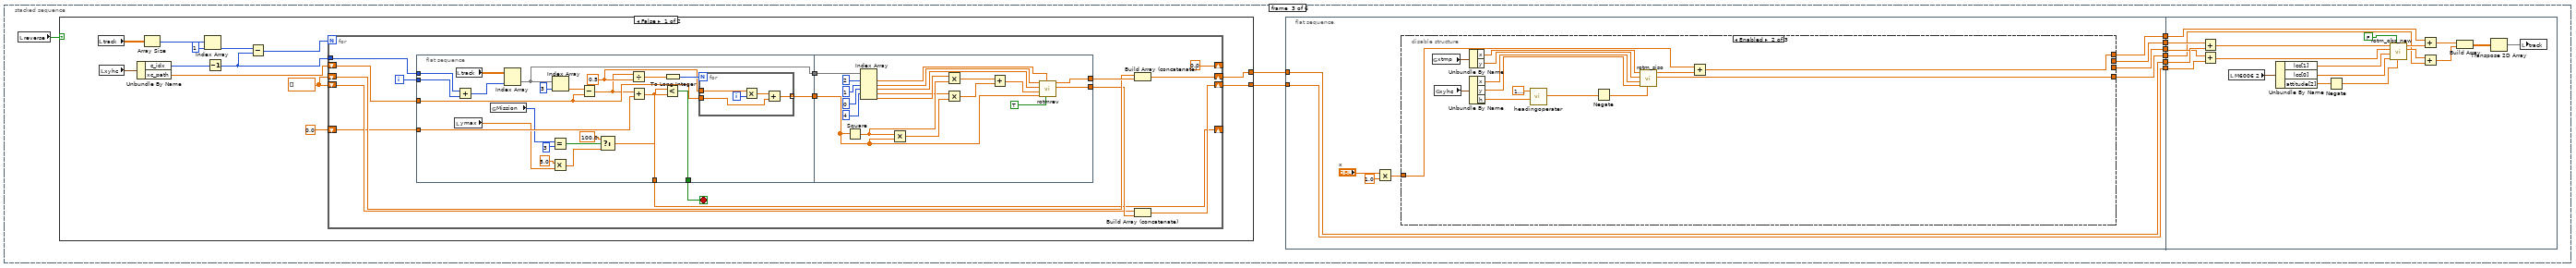
[diagram p3: hidden frame]
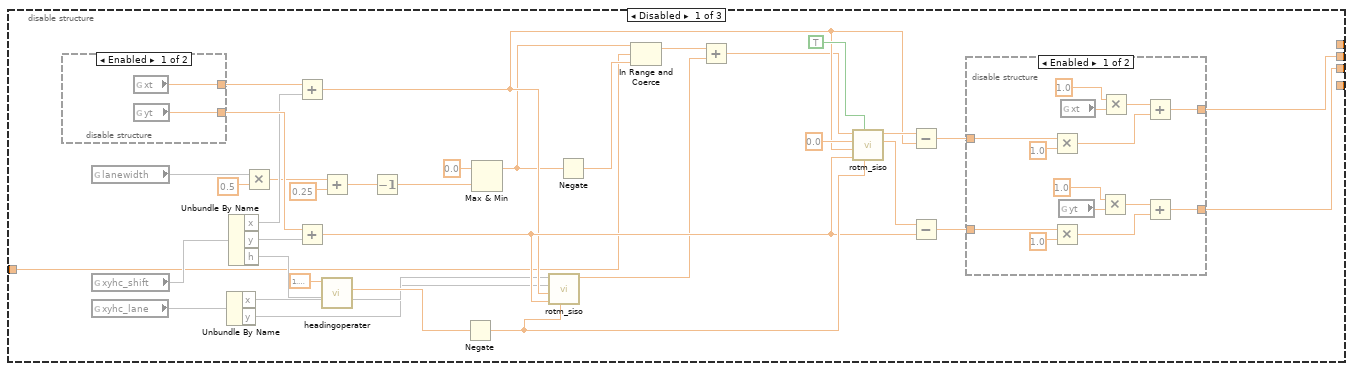
[diagram p4: hidden frame]
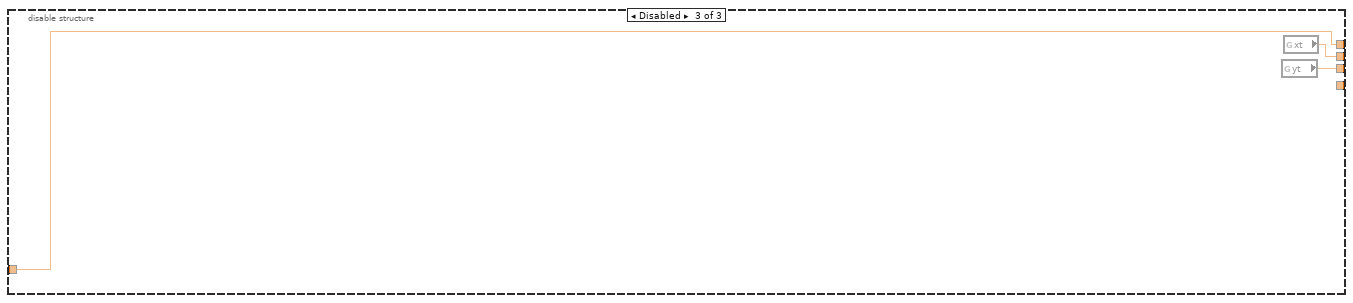
[diagram p7: hidden frame]
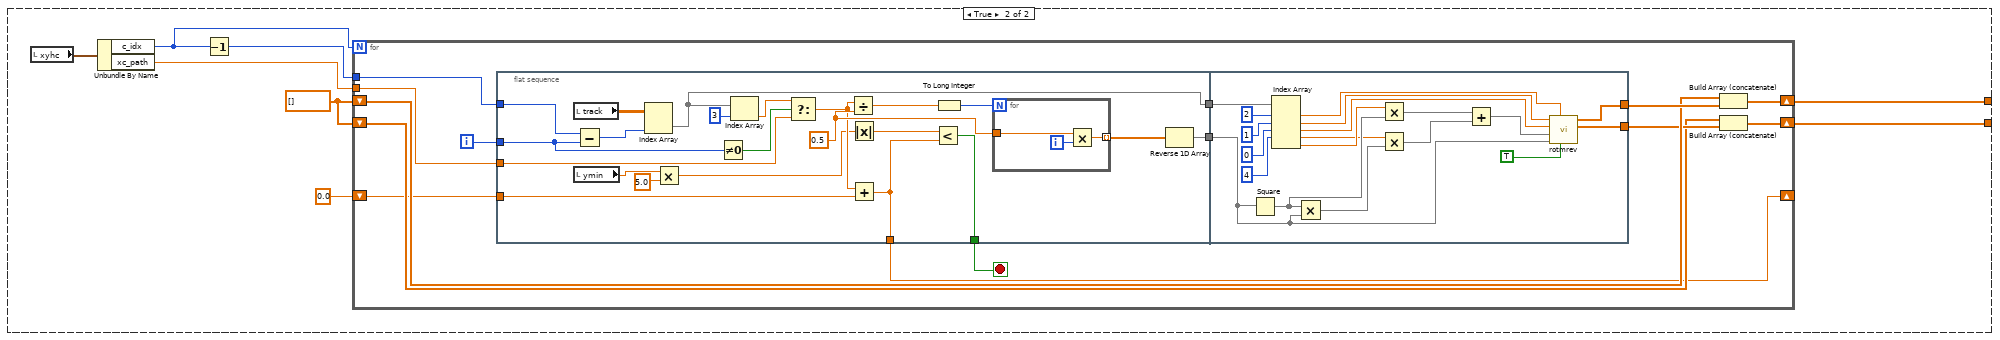
[diagram p8: hidden frame]
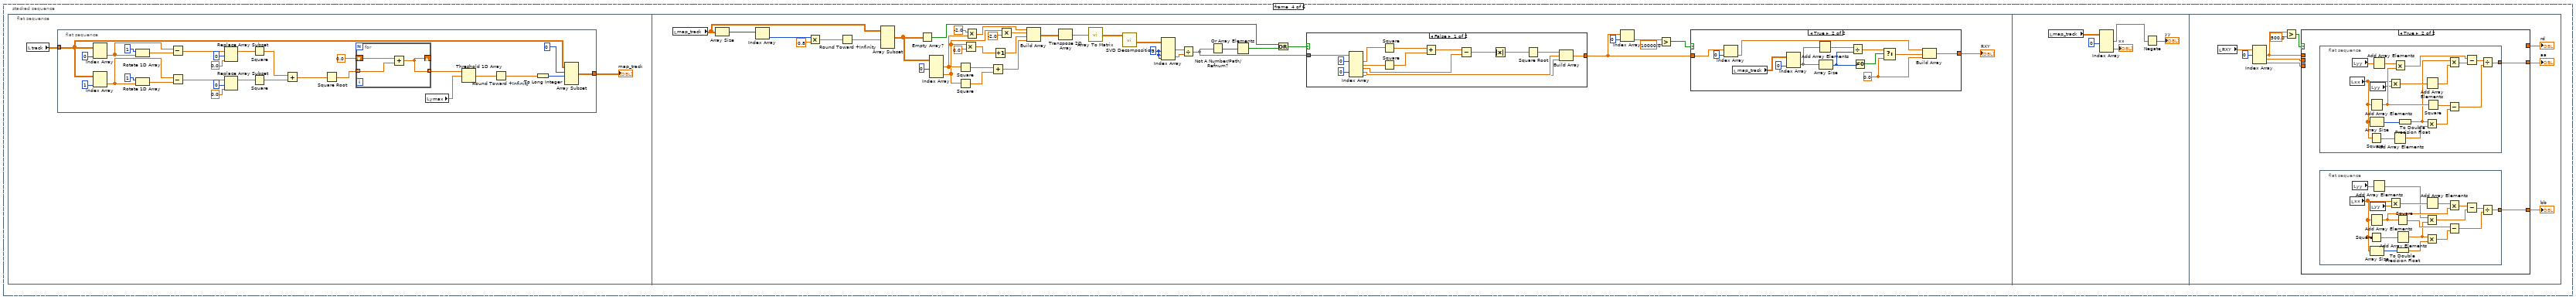
[diagram p9: hidden frame]
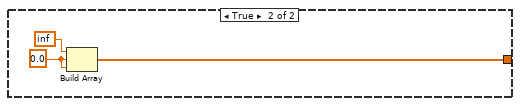
[diagram p10: hidden frame]
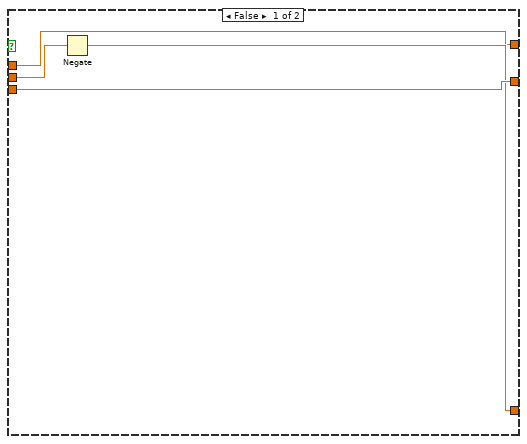
[diagram p12: hidden frame]
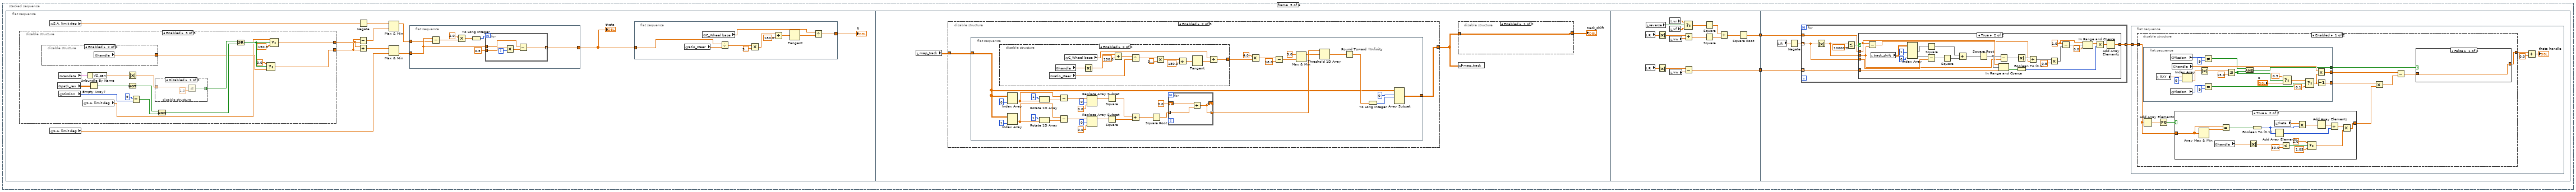
[diagram p13: hidden frame]
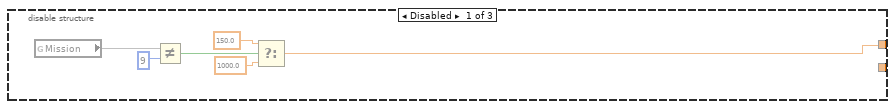
[diagram p14: hidden frame]
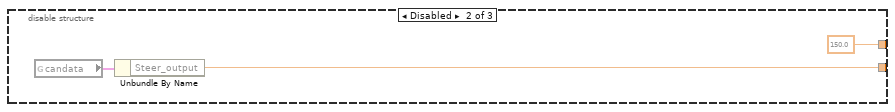
[diagram p15: hidden frame]
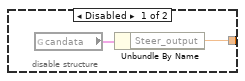
[diagram p16: hidden frame]
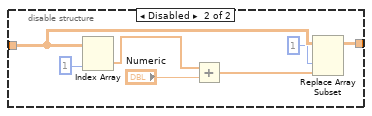
[diagram p18: hidden frame]
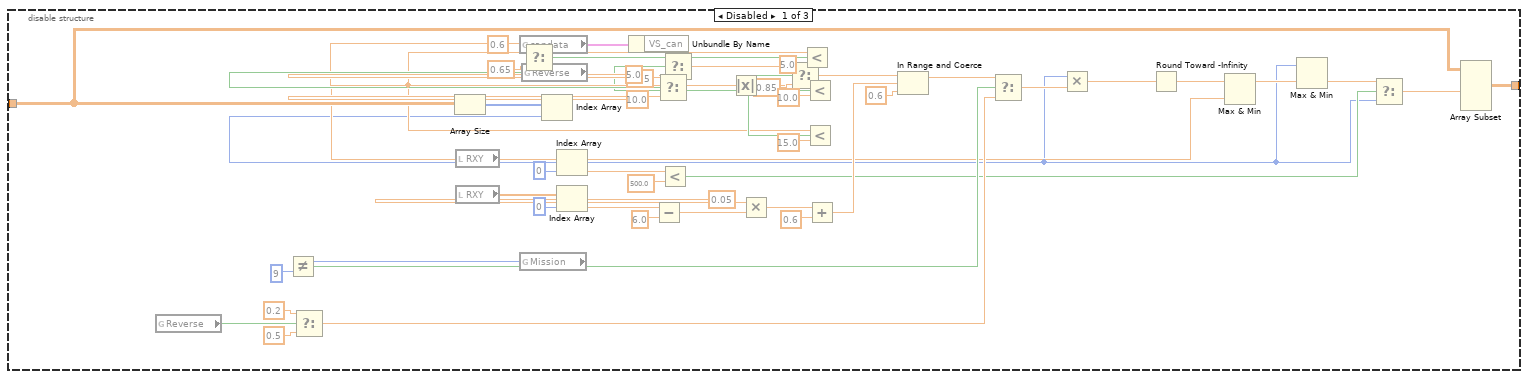
[diagram p19: hidden frame]
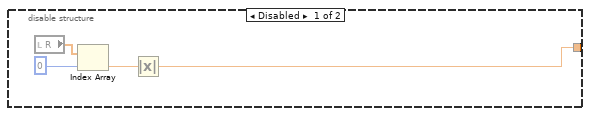
[diagram p20: hidden frame]
diagram:
  n1 = stacked-sequence {
    frame #0 {
      n2 = Tick Count (ms)() -> (millisecond timer value=→"tic":u32)
    }
    frame #1 {
      n3 = flat-sequence {
        frame #0 {
          n4 = global read "G_NAV.vi" "M6006"() -> (→"M6006 2":T1)
        }
      }
      n5 = flat-sequence {
        frame #0 {
          n6 = Multiply(x=1.805 ("width"), y=0.5) -> (x*y=w22:dbl)
          n7 = Add(x=w22, y="margin") -> (x+y=→"vw":dbl)
          "lw" <- 0.4 ("width")
          "vf" <- 3.5 ("af")
          "vr" <- 0.75 ("ar")
          "stack" <- FALSE
        }
      }
      n8 = flat-sequence {
        frame #0 {
          n9 = global read "G_VEH.vi" "candata"() -> (w39:T3)
          n10 = Unbundle By Name(w39) -> ("VS_can"=w36:dbl)
          n11 = Absolute Value(x=w36) -> (abs(x)=w32:dbl)
          n12 = Multiply(x=w32, y=0.85 ("vgain")) -> (x*y=w31:dbl)
          n13 = In Range and Coerce(upper limit=60.0, x=w31, lower limit=45.0 ("y")) -> (coerced(x)=w35:dbl)  [unwired: 1 out]
          "ymax" <- w35
          n14 = Multiply(x=w35, y=-0.5) -> (x*y=→"ymin":dbl)
        }
      }
      n15 = flat-sequence {
        frame #0 {
          n16 = global read "G_VEH.vi" "xyhc"() -> (w7:T4)
          n17 = global read "G_PATH.vi" "path"() -> (w2:dbl[][])
          n18 = Select(t=w2, s=TRUE ("B_track"), f=dbl[][] []) -> (s? t:f=→"track":dbl[][])
          n19 = Select(t=w7, s=TRUE ("B_track"), f=T2 {"c_idx"=0, "xc"=0.0, "yc"=0.0, "hc"=0.0, "xc_path"=0.0}) -> (s? t:f=→"xyhc":T2)
        }
        frame #1 {
          n20 = local read "xyhc"() -> (w19:T2)
          n21 = global read "G_VEH.vi" "candata"() -> (w13:T3)
          n22 = Unbundle By Name(w19) -> ("c_idx"=w17:i32)
          n23 = Unbundle By Name(w13) -> ("VS_can"=w14:dbl)
          n24 = Decrement(x=w17) -> (x-1=w18:i32)
          n25 = local read "track"() -> (w20:dbl[][])
          n26 = Index Array(array=w20, index (row)=6, index (col)=w18) -> (element=w15:dbl)
          n27 = Less Or Equal To 0?(x=w14) -> (x <= 0?=w11:bool)
          n28 = Less Than 0?(x=w15) -> (x < 0?=w12:bool)
          n29 = global write "G_VEH.vi" "Reverse"(w12) -> ()
          n30 = And(x=w12, y=w11) -> (x .and. y?=→"reverse":bool)
        }
      }
    }
    frame #2 {
      n31 = local read "reverse"() -> (w47:bool)
      n32 = case shown="False" w47 {
        tunnel: [w151 w227] -> w49
        tunnel: [w150 w226] -> w48
        frame False {
          w153 = dbl[] [] ("x")
          n33 = local read "track"() -> (w148:dbl[][])
          n34 = local read "xyhc"() -> (w147:T2)
          n35 = Unbundle By Name(w147) -> ("c_idx"=w159:i32, "xc_path"=w154:dbl)
          n36 = Array Size(array=w148) -> (size(s)=w158:i32[])
          n37 = Index Array(array=w158, index=1) -> (element=w156:i32)
          n38 = Decrement(x=w159) -> (x-1=w155:i32)
          n39 = Subtract(x=w156, y=w155) -> (x-y=w152:i32)
          n40 = for {
            N: w152 -> [_]
            tunnel: w155 -> [w173]
            shift-right: [0.0 ("xc_path")] -> _
            shift-left: w154 -> [w171]
            shift-right: [w166] -> w151
            shift-left: w153 -> [w167]
            shift-right: [w163] -> w150
            shift-left: w153 -> [w164]
            shift-right: [w161] -> _
            shift-left: 0.0 -> [w162]
            i -> [w174]
            stop <- w160 stop-if-true
            n41 = flat-sequence {
              tunnel: w174 -> [w198]
              tunnel: w173 -> [w197]
              tunnel: w171 -> [w191]
              tunnel: [w189] -> w170
              tunnel: [w188] -> w169
              tunnel: w162 -> [w186]
              tunnel: [w185] -> w161
              tunnel: [w184] -> w160
              tunnel: w170 -> [w214]
              tunnel: w169 -> [w215]
              tunnel: [w206] -> w168
              tunnel: [w205] -> w165
              frame #0 {
                w190 = 0.5 ("y")
                n42 = local read "ymax"() -> (w182:dbl)
                n43 = local read "track"() -> (w183:dbl[][])
                n44 = Add(x=w197, y=w198) -> (x+y=w196:i32)
                n45 = global read "G_PATH.vi" "Mission"() -> (w175:i32)
                n46 = Index Array(array=w183, index (col)=w196) -> (element=w188:dbl[])  [unwired: 1 in]
                n47 = Equal?(x=w175, y=3) -> (x = y?=w180:bool)
                n48 = Multiply(x=5.0 ("f"), y=w182) -> (x*y=w177:dbl)
                n49 = Index Array(array=w188, index=3) -> (element=w194:dbl)
                n50 = Subtract(x=w194, y=w191) -> (x-y=w187:dbl)
                n51 = Select(t=100.0 ("x"), s=w180, f=w177) -> (s? t:f=w176:dbl)
                n52 = Divide(x=w187, y=w190) -> (x/y=w193:dbl)
                n53 = Add(x=w187, y=w186) -> (x+y=w185:dbl)
                n54 = Less?(x=w176, y=w185) -> (x < y?=w184:bool)
                n55 = To Long Integer(number=w193) -> (32bit integer=w192:i32)
                n56 = for {
                  N: w192 -> [_]
                  tunnel: w191 -> [w199]
                  tunnel: w190 -> [w202]
                  tunnel: [w201] -> w189 mode=indexing
                  i -> [w203]
                  n57 = Multiply(x=w202, y=w203) -> (x*y=w200:dbl)
                  n58 = Add(x=w200, y=w199) -> (x+y=w201:dbl)
                }
              }
              frame #1 {
                n59 = Square(x=w214) -> (x^2=w220:dbl[])
                n60 = Index Array(array=w215, index #1=2 ("index"), index #2=1 ("index"), index #3=0 ("index"), index #4=4 ("index")) -> (element #1=w209:dbl, element #2=w208:dbl, element #3=w207:dbl, element #4=w219:dbl, element #5=w221:dbl)  [unwired: 1 in]
                n61 = Multiply(x=w220, y=w214) -> (x*y=w218:dbl[])
                n62 = Multiply(x=w221, y=w220) -> (x*y=w217:dbl[])
                n63 = Multiply(x=w219, y=w218) -> (x*y=w216:dbl[])
                n64 = Add(x=w217, y=w216) -> (x+y=w213:dbl[])
                n65 = call "rotmrev.vi"("reverse"=TRUE, "angle[rad]"=w209, "x"=w214, "y"=w213, "x0"=w207, "y0"=w208) -> ("y"=w205:dbl[], "x"=w206:dbl[])  [unwired: 4 in]
              }
            }
            n66 = Build Array (concatenate)(w167, w168) -> (w166:dbl[])
            n67 = Build Array (concatenate)(w164, w165) -> (w163:dbl[])
          }
        }
        frame True {
          w228 = dbl[] [] ("x")
          n68 = local read "xyhc"() -> (w223:T2)
          n69 = Unbundle By Name(w223) -> ("c_idx"=w225:i32, "xc_path"=w229:dbl)
          n70 = Decrement(x=w225) -> (x-1=w230:i32)
          n71 = for {
            N: w225 -> [_]
            tunnel: w230 -> [w243]
            shift-right: [w237] -> w227
            shift-left: w228 -> [w238]
            shift-right: [w234] -> w226
            shift-left: w228 -> [w235]
            tunnel: w229 -> [w242]
            shift-right: [w232] -> _
            shift-left: 0.0 -> [w233]
            i -> [w244]
            stop <- w231 stop-if-true
            n72 = flat-sequence {
              tunnel: w244 -> [w259]
              tunnel: w243 -> [w266]
              tunnel: w242 -> [w256]
              tunnel: [w254] -> w241
              tunnel: [w260] -> w240
              tunnel: w233 -> [w252]
              tunnel: [w251] -> w232
              tunnel: [w250] -> w231
              tunnel: w241 -> [w280]
              tunnel: w240 -> [w281]
              tunnel: [w272] -> w239
              tunnel: [w271] -> w236
              frame #0 {
                w261 = 0.5 ("y")
                n73 = local read "track"() -> (w249:dbl[][])
                n74 = local read "ymin"() -> (w247:dbl)
                n75 = Subtract(x=w266, y=w259) -> (x-y=w265:i32)
                n76 = Index Array(array=w249, index (col)=w265) -> (element=w260:dbl[])  [unwired: 1 in]
                n77 = Multiply(x=w247, y=5.0) -> (x*y=w246:dbl)
                n78 = Not Equal To 0?(x=w259) -> (x != 0?=w258:bool)
                n79 = Index Array(array=w260, index=3) -> (element=w257:dbl)
                n80 = Select(t=w257, s=w258, f=w256) -> (s? t:f=w253:dbl)
                n81 = Divide(x=w253, y=w261) -> (x/y=w263:dbl)
                n82 = Absolute Value(x=w246) -> (abs(x)=w248:dbl)
                n83 = Add(x=w253, y=w252) -> (x+y=w251:dbl)
                n84 = Less?(x=w248, y=w251) -> (x < y?=w250:bool)
                n85 = To Long Integer(number=w263) -> (32bit integer=w262:i32)
                n86 = for {
                  N: w262 -> [_]
                  tunnel: w261 -> [w268]
                  tunnel: [w267] -> w255 mode=indexing
                  i -> [w269]
                  n87 = Multiply(x=w268, y=w269) -> (x*y=w267:dbl)
                }
                n88 = Reverse 1D Array(array=w255) -> (reversed array=w254:dbl[])
              }
              frame #1 {
                n89 = Square(x=w280) -> (x^2=w286:dbl[])
                n90 = Index Array(array=w281, index #1=2 ("index"), index #2=1 ("index"), index #3=0 ("index"), index #4=4 ("index")) -> (element #1=w275:dbl, element #2=w274:dbl, element #3=w273:dbl, element #4=w285:dbl, element #5=w287:dbl)  [unwired: 1 in]
                n91 = Multiply(x=w286, y=w280) -> (x*y=w284:dbl[])
                n92 = Multiply(x=w287, y=w286) -> (x*y=w283:dbl[])
                n93 = Multiply(x=w285, y=w284) -> (x*y=w282:dbl[])
                n94 = Add(x=w283, y=w282) -> (x+y=w279:dbl[])
                n95 = call "rotmrev.vi"("reverse"=TRUE, "angle[rad]"=w275, "x"=w280, "y"=w279, "x0"=w273, "y0"=w274) -> ("y"=w271:dbl[], "x"=w272:dbl[])  [unwired: 4 in]
              }
            }
            n96 = Build Array (concatenate)(w238, w239) -> (w237:dbl[])
            n97 = Build Array (concatenate)(w235, w236) -> (w234:dbl[])
          }
        }
      }
      n98 = flat-sequence {
        tunnel: w48 -> [w57]
        tunnel: w49 -> [w58]
        tunnel: [w58] -> w46
        tunnel: [w57] -> w45
        tunnel: [w56] -> w44
        tunnel: [w55] -> w43
        tunnel: [w51] -> w42
        tunnel: [w50] -> w41
        tunnel: w46 -> [w138]
        tunnel: w45 -> [w136]
        tunnel: w44 -> [w134]
        tunnel: w43 -> [w133]
        tunnel: w42 -> [w131]
        tunnel: w41 -> [w127]
        frame #0 {
          n99 = Multiply(x="x", y=1.0) -> (x*y=w52:dbl)
          n100 = disable-structure shown="Enabled" {
            disable-tunnel: [w65 _ w126] -> w56
            disable-tunnel: [w64 _ w125] -> w55
            disable-tunnel: w52 -> [w60 w119 w124]
            disable-tunnel: [_ w118 w124] -> w51
            disable-tunnel: [_ w117 _] -> w50
            frame Disabled {
              n101 = disable-structure shown="Enabled" {
                disable-tunnel: [w109 _] -> w78
                disable-tunnel: [w108 _] -> w80
                frame Enabled {
                  n102 = global read "G_PATH.vi" "xt"() -> (w109:dbl)
                  n103 = global read "G_PATH.vi" "yt"() -> (w108:dbl)
                }
                frame Disabled {
                }
              }
              n104 = global read "G_PATH.vi" "lanewidth"() -> (w71)
              n105 = global read "G_VEH.vi" "xyhc_shift"() -> (w74)
              n106 = global read "G_VEH.vi" "xyhc_lane"() -> (w93)
              n107 = Unbundle By Name(w93) -> ("x"=w76, "y"=w75)
              n108 = Unbundle By Name(w74) -> ("x"=w77, "y"=w79, "h"=w83)
              n109 = Multiply(x=w71, y=0.5) -> (x*y=w63:dbl)
              n110 = Add(x=w78, y=w77) -> (x+y=w85:dbl)
              n111 = Add(x=w80, y=w79) -> (x+y=w86:dbl)
              n112 = Add(x=w63, y=0.25) -> (x+y=w61:dbl)
              n113 = call "headingoperater.vi"("h1"=w83, "h2"=1.5707963267948966) -> ("h2-h1"=w91:dbl)  [unwired: 8 in, 1 out]
              n114 = Decrement(x=w61) -> (x-1=w68:dbl)
              n115 = Negate(x=w91) -> (-x=w92:dbl)
              n116 = Max & Min(x=0.0, y=w68) -> (max(x,y)=w67:dbl)  [unwired: 1 out]
              n117 = call "rotm_siso.vi"("angle[rad]"=w92, "y0"=w86, "x0"=w85, "y"=w75, "x"=w76) -> ("x'"=w73:dbl)  [unwired: 5 in, 1 out]
              n118 = Negate(x=w67) -> (-x=w66:dbl)
              n119 = In Range and Coerce(upper limit=w67, x=w60, lower limit=w66) -> (coerced(x)=w59:dbl)  [unwired: 1 out]
              n120 = Add(x=w59, y=w73) -> (x+y=w72:dbl)
              n121 = call "rotm_siso.vi"("angle[rad]"=w92, "reverse"=TRUE, "y0"=w86, "x0"=w85, "y"=0.0, "x"=w72) -> ("y'"=w89:dbl, "x'"=w88:dbl)  [unwired: 4 in]
              n122 = Subtract(x=w88, y=w85) -> (x-y=w81:dbl)
              n123 = Subtract(x=w89, y=w86) -> (x-y=w82:dbl)
              n124 = disable-structure shown="Enabled" {
                disable-tunnel: w81 -> [w103 _]
                disable-tunnel: w82 -> [w97 _]
                disable-tunnel: [w95 _] -> w65
                disable-tunnel: [w94 _] -> w64
                frame Enabled {
                  n125 = Multiply(x=w103, y=1.0 ("x")) -> (x*y=w102:dbl)
                  n126 = Multiply(x=w97, y=1.0 ("x")) -> (x*y=w96:dbl)
                  n127 = global read "G_PATH.vi" "yt"() -> (w100:dbl)
                  n128 = global read "G_PATH.vi" "xt"() -> (w107:dbl)
                  n129 = Multiply(x=1.0, y=w100) -> (x*y=w99:dbl)
                  n130 = Multiply(x=1.0, y=w107) -> (x*y=w105:dbl)
                  n131 = Add(x=w105, y=w102) -> (x+y=w95:dbl)
                  n132 = Add(x=w99, y=w96) -> (x+y=w94:dbl)
                }
                frame Disabled {
                }
              }
            }
            frame Enabled {
              n133 = global read "G_VEH.vi" "xtmp"() -> (w123:T4)
              n134 = global read "G_VEH.vi" "xyhc"() -> (w113:T4)
              n135 = Unbundle By Name(w123) -> ("x"=w116:dbl, "y"=w115:dbl)
              n136 = Unbundle By Name(w113) -> ("x"=w122:dbl, "y"=w121:dbl, "h"=w111:dbl)
              n137 = call "headingoperater.vi"("h1"=w111, "h2"=1.5707963267948966) -> ("h2-h1"=w110:dbl)  [unwired: 8 in, 1 out]
              n138 = Negate(x=w110) -> (-x=w120:dbl)
              n139 = call "rotm_siso.vi"("angle[rad]"=w120, "y0"=w121, "x0"=w122, "y"=w115, "x"=w116) -> ("y'"=w117:dbl, "x'"=w114:dbl)  [unwired: 5 in]
              n140 = Add(x=w119, y=w114) -> (x+y=w118:dbl)
            }
            frame Disabled {
              n141 = global read "G_PATH.vi" "yt"() -> (w125:dbl)
              n142 = global read "G_PATH.vi" "xt"() -> (w126:dbl)
            }
          }
        }
        frame #1 {
          n143 = Add(x=w134, y=w138) -> (x+y=w137:dbl[])
          n144 = Add(x=w133, y=w136) -> (x+y=w135:dbl[])
          n145 = local read "M6006 2"() -> (w140:T1)
          n146 = Unbundle By Name(w140) -> ("lcc[1]"=w144:dbl, "lcc[0]"=w143:dbl, "attitude[2]"=w139:dbl)
          n147 = Negate(x=w139) -> (-x=w141:dbl)
          n148 = call "rotm_obs_new.vi"("angle[rad]"=w141, "reverse"=FALSE, "y0"=w143, "x0"=w144, "y"=w135, "x"=w137) -> ("rot*(y-y0) 2"=w129:dbl[], "rot*(x-x0)"=w132:dbl[])  [unwired: 2 in, 2 out]
          n149 = Add(x=w131, y=w132) -> (x+y=w130:dbl[])
          n150 = Add(x=w129, y=w127) -> (x+y=w128:dbl[])
          n151 = Build Array(w130, w128) -> (w145:dbl[][])
          n152 = Transpose 2D Array(2D array=w145) -> (transposed array=w146:dbl[][])
          n153 = local write "track"(w146) -> ()
        }
      }
    }
    frame #3 {
      n154 = flat-sequence {
        frame #0 {
          n155 = local read "track"() -> (w290:dbl[][])
          n156 = flat-sequence {
            tunnel: w290 -> [w292]
            tunnel: [w291] -> w289
            frame #0 {
              n157 = Index Array(array=w292, index (col)=0 ("disabled index (col)")) -> (element=w316:dbl[])  [unwired: 1 in]
              n158 = Index Array(array=w292, index (col)=1 ("disabled index (col)")) -> (element=w305:dbl[])  [unwired: 1 in]
              n159 = Rotate 1D Array(1:w316, 2:1 ("n")) -> (0:w315:dbl[])
              n160 = Rotate 1D Array(1:w305, 2:1 ("n")) -> (0:w306:dbl[])
              n161 = Subtract(x=w316, y=w315) -> (x-y=w314:dbl[])
              n162 = Subtract(x=w305, y=w306) -> (x-y=w307:dbl[])
              n163 = Replace Array Subset(array=w314, new element=0.0 ("new element/subarray"), index=0) -> (w311:dbl[])
              n164 = Replace Array Subset(array=w307, new element=0.0 ("new element/subarray"), index=0) -> (w310:dbl[])
              n165 = Square(x=w311) -> (x^2=w302:dbl[])
              n166 = Square(x=w310) -> (x^2=w301:dbl[])
              n167 = Add(x=w302, y=w301) -> (x+y=w300:dbl[])
              n168 = Square Root(x=w300) -> (sqrt(x)=w299:dbl[])
              n169 = for {
                tunnel: w299 -> [w322] mode=indexing
                shift-right: [w320] -> _
                shift-left: 0.0 -> [w321]
                tunnel: [w320] -> w293 mode=indexing
                n170 = Add(x=w321, y=w322) -> (x+y=w320:dbl)
              }
              n171 = local read "ymax"() -> (w297:dbl)
              n172 = Threshold 1D Array(2:w297, 3:w293) -> (0:w296:dbl)  [unwired: 1 in]
              n173 = Round Toward +Infinity(x=w296) -> (ceil(x): smallest int >= x=w295:dbl)
              n174 = To Long Integer(number=w295) -> (32bit integer=w319:i32)
              n175 = Array Subset(array=w292, index (row)=0 ("index"), length (row)=w319) -> (w291:dbl[][])  [unwired: 2 in]
            }
          }
          "map_track" <- w289
        }
        frame #1 {
          w337 = 3 ("disabled index (col)")
          n176 = local read "map_track"() -> (w323:dbl[][])
          n177 = Array Size(array=w323) -> (size(s)=w328:i32[])
          n178 = Index Array(array=w328) -> (element=w327:i32)  [unwired: 1 in]
          n179 = Multiply(x=w327, y=0.8) -> (x*y=w325:dbl)
          n180 = Round Toward +Infinity(x=w325) -> (ceil(x): smallest int >= x=w324:dbl)
          n181 = Array Subset(array=w323, length (row)=w324) -> (w329:dbl[][])  [unwired: 3 in]
          n182 = Empty Array?(array=w329) -> (empty?=w331:bool)
          n183 = Index Array(array=w329, index (col) #1=0 ("disabled index (col)")) -> (element #1=w346:dbl[], element #2=w345:dbl[])  [unwired: 3 in]
          n184 = Square(x=w346) -> (x^2=w344:dbl[])
          n185 = Square(x=w345) -> (x^2=w343:dbl[])
          n186 = Multiply(x=w345, y=0.0) -> (x*y=w348:dbl[])
          n187 = Multiply(x=-2.0, y=w346) -> (x*y=w351:dbl[])
          n188 = Add(x=w344, y=w343) -> (x+y=w342:dbl[])
          n189 = Increment(x=w348) -> (x+1=w347:dbl[])
          n190 = Multiply(x=w345, y=-2.0) -> (x*y=w350:dbl[])
          n191 = Build Array(w351, w350, w347, w342) -> (w341:dbl[][])
          n192 = Transpose 2D Array(2D array=w341) -> (transposed array=w340:dbl[][])
          n193 = call-poly <vilib>:"Array To Matrix.vi"("Real 2D Array"=w340) -> ("Real Matrix"=w339:T5)
          n194 = call-poly <vilib>:"SVD Decomposition.vi"("A"=w339) -> ("Matrix V"=w338:T5)  [unwired: 6 in, 4 out]
          n195 = Index Array(array=w338, index (col) #1=w337, index (row) #2=w337, index (col) #2=w337) -> (element #1=w336:dbl[], element #2=w335:dbl)  [unwired: 1 in]
          n196 = Divide(x=w336, y=w335) -> (x/y=w334:dbl[])
          n197 = Not A Number/Path/Refnum?(number/path/refnum=w334) -> (NaN/Path/Refnum?=w333:bool[])
          n198 = Or Array Elements(Boolean array=w333) -> (logical OR=w332:bool)
          n199 = Or(x=w331, y=w332) -> (x .or. y?=w330:bool)
          n200 = case shown="False" w330 {
            tunnel: [w365 w376] -> w355
            tunnel: w334 -> [w361 _]
            frame False {
              n201 = Index Array(array=w361, index #1=0 ("index"), index #4=0 ("index")) -> (element #1=w374:dbl, element #2=w373:dbl, element #3=w366:dbl, element #4=w363:dbl, element #5=w362:dbl)  [unwired: 3 in]
              n202 = Square(x=w374) -> (x^2=w372:dbl)
              n203 = Square(x=w373) -> (x^2=w371:dbl)
              n204 = Add(x=w372, y=w371) -> (x+y=w367:dbl)
              n205 = Subtract(x=w367, y=w366) -> (x-y=w369:dbl)
              n206 = Absolute Value(x=w369) -> (abs(x)=w370:dbl)
              n207 = Square Root(x=w370) -> (sqrt(x)=w368:dbl)
              n208 = Build Array(w368, w363, w362) -> (w365:dbl[])
            }
            frame True {
              w378 = 0.0 ("element")
              n209 = Build Array(inf, w378, w378) -> (w376:dbl[])
            }
          }
          n210 = Index Array(array=w355, index=0) -> (element=w359:dbl)
          n211 = Greater?(x=w359, y=10000.0) -> (0:w357:bool)
          n212 = case shown="True" w357 {
            tunnel: [w379 w385] -> w356
            tunnel: w355 -> [w379 w388]
            frame False {
            }
            frame True {
              w380 = 0.0 ("element")
              n213 = Index Array(array=w388, index=0) -> (element=w386:dbl)
              n214 = local read "map_track"() -> (w392:dbl[][])
              n215 = Index Array(array=w392, index (col)=0 ("disabled index (col)")) -> (element=w390:dbl[])  [unwired: 1 in]
              n216 = Add Array Elements(numeric array=w390) -> (sum=w389:dbl)
              n217 = Array Size(array=w390) -> (size(s)=w384:i32)
              n218 = Divide(x=w389, y=w384) -> (x/y=w382:dbl)
              n219 = Not Equal To 0?(x=w384) -> (x != 0?=w383:bool)
              n220 = Select(t=w382, s=w383, f=w380) -> (s? t:f=w381:dbl)
              n221 = Build Array(w386, w381, w380) -> (w385:dbl[])
            }
          }
          "RXY" <- w356
        }
        frame #2 {
          n222 = local read "map_track"() -> (w397:dbl[][])
          n223 = Index Array(array=w397, index (col) #1=0 ("disabled index (col)")) -> (element #1=w395:dbl[], element #2=→"xx":dbl[])  [unwired: 3 in]
          n224 = Negate(x=w395) -> (-x=→"yy":dbl[])
        }
        frame #3 {
          n225 = local read "RXY"() -> (w407:dbl[])
          n226 = Index Array(array=w407, index #1=0 ("index")) -> (element #1=w398:dbl, element #2=w403:dbl, element #3=w401:dbl)  [unwired: 2 in]
          n227 = Greater?(x=w398, y=500.0) -> (0:w404:bool)
          n228 = case shown="True" w404 {
            tunnel: w403 -> [w411 _]
            tunnel: [w410 w413] -> w402
            tunnel: w401 -> [w410 _]
            tunnel: [w409 w412] -> w400
            tunnel: [w408 _] -> w399
            tunnel: w398 -> [w408 _]
            frame False {
              n229 = Negate(x=w411) -> (-x=w409:dbl)
            }
            frame True {
              n230 = flat-sequence {
                tunnel: [w416] -> w413
                frame #0 {
                  n231 = local read "xx"() -> (w417:dbl[])
                  n232 = local read "yy"() -> (w419:dbl[])
                  n233 = Square(x=w417) -> (x^2=w420:dbl[])
                  n234 = local read "yy"() -> (w418:dbl[])
                  n235 = Add Array Elements(numeric array=w417) -> (sum=w425:dbl)
                  n236 = Array Size(array=w417) -> (size(s)=w421:i32)
                  n237 = Add Array Elements(numeric array=w419) -> (sum=w424:dbl)
                  n238 = Multiply(x=w417, y=w418) -> (x*y=w426:dbl[])
                  n239 = Multiply(x=w424, y=w425) -> (x*y=w428:dbl)
                  n240 = Add Array Elements(numeric array=w420) -> (sum=w415:dbl)
                  n241 = To Double Precision Float(number=w421) -> (double precision float=w414:dbl)
                  n242 = Add Array Elements(numeric array=w426) -> (sum=w427:dbl)
                  n243 = Multiply(x=w414, y=w415) -> (x*y=w422:dbl)
                  n244 = Square(x=w425) -> (x^2=w423:dbl)
                  n245 = Multiply(x=w414, y=w427) -> (x*y=w429:dbl)
                  n246 = Subtract(x=w423, y=w422) -> (x-y=w431:dbl)
                  n247 = Subtract(x=w428, y=w429) -> (x-y=w430:dbl)
                  n248 = Divide(x=w430, y=w431) -> (x/y=w416:dbl)
                }
              }
              n249 = flat-sequence {
                tunnel: [w432] -> w412
                frame #0 {
                  n250 = local read "xx"() -> (w449:dbl[])
                  n251 = local read "yy"() -> (w447:dbl[])
                  n252 = Square(x=w449) -> (x^2=w446:dbl[])
                  n253 = local read "yy"() -> (w448:dbl[])
                  n254 = Add Array Elements(numeric array=w449) -> (sum=w442:dbl)
                  n255 = Array Size(array=w449) -> (size(s)=w445:i32)
                  n256 = Add Array Elements(numeric array=w447) -> (sum=w434:dbl)
                  n257 = Multiply(x=w449, y=w448) -> (x*y=w440:dbl[])
                  n258 = Square(x=w442) -> (x^2=w443:dbl)
                  n259 = Add Array Elements(numeric array=w446) -> (sum=w433:dbl)
                  n260 = To Double Precision Float(number=w445) -> (double precision float=w441:dbl)
                  n261 = Add Array Elements(numeric array=w440) -> (sum=w435:dbl)
                  n262 = Multiply(x=w434, y=w433) -> (x*y=w438:dbl)
                  n263 = Multiply(x=w433, y=w441) -> (x*y=w444:dbl)
                  n264 = Multiply(x=w435, y=w442) -> (x*y=w439:dbl)
                  n265 = Subtract(x=w443, y=w444) -> (x-y=w436:dbl)
                  n266 = Subtract(x=w439, y=w438) -> (x-y=w437:dbl)
                  n267 = Divide(x=w437, y=w436) -> (x/y=w432:dbl)
                }
              }
            }
          }
          "aa" <- w402
          "bb" <- w400
          "rd" <- w399
        }
      }
    }
    frame #4 {
      n268 = flat-sequence {
        tunnel: [w654] -> w451
        tunnel: [w655] -> w450
        tunnel: w451 -> [w658]
        tunnel: w450 -> [w657]
        frame #0 {
          n269 = disable-structure shown="Enabled" {
            disable-tunnel: [w464 150.0 ("t") w488] -> w453
            disable-tunnel: [_ w469 w487] -> w452
            frame Disabled {
              n270 = global read "G_VEH.vi" "Mission"() -> (w467)
              n271 = Not Equal?(x=w467, y=9) -> (x != y?=w466:bool)
              n272 = Select(t=150.0 ("x"), s=w466, f=1000.0) -> (s? t:f=w464:dbl)
            }
            frame Disabled {
              n273 = global read "G_VEH.vi" "candata"() -> (w471:T3)
              n274 = Unbundle By Name(w471) -> ("Steer_output"=w469:dbl)
            }
            frame Enabled {
              n275 = disable-structure shown="Enabled" {
                disable-tunnel: [w490 w492] -> w473
                frame Disabled {
                  n276 = global read "G_VEH.vi" "candata"() -> (w491:T3)
                  n277 = Unbundle By Name(w491) -> ("Steer_output"=w490:dbl)
                }
                frame Enabled {
                  n278 = global read "G_VEH.vi" "handle"() -> (w492:dbl)
                }
              }
              n279 = global read "G_PATH.vi" "path_rev"() -> (w483:dbl[][])
              n280 = global read "G_VEH.vi" "candata"() -> (w489:T3)
              n281 = global read "G_PATH.vi" "Mission"() -> (w472:i32)
              n282 = global read "G_VEH.vi" "S.A. limit deg"() -> (w475:dbl)
              n283 = Unbundle By Name(w489) -> ("VS_can"=w486:dbl)
              n284 = Empty Array?(array=w483) -> (empty?=w482:bool)
              n285 = Absolute Value(x=w486) -> (abs(x)=w485:dbl)
              n286 = Not(x=w482) -> (.not. x?=w481:bool)
              n287 = Equal?(x=9 ("y"), y=w472) -> (x = y?=w480:bool)
              n288 = disable-structure shown="Disabled" {
                disable-tunnel: w485 -> [w495 _]
                disable-tunnel: [w493 _] -> w478
                frame Disabled {
                  n289 = Less Or Equal?(x=w495, y=1.0) -> (x <= y?=w493:bool)
                }
                frame Enabled {
                }
              }
              n290 = And(x=w481, y=w480) -> (x .and. y?=w479:bool)
              n291 = Or(x=w478, y=w479) -> (x .or. y?=w477:bool)
              n292 = Select(t=0.0 ("f"), s=w477, f=w473) -> (s? t:f=w487:dbl)
              n293 = Select(t=w475, s=w477, f=150.0 ("t")) -> (s? t:f=w488:dbl)
            }
          }
          n294 = global read "G_VEH.vi" "S.A. limit deg"() -> (w462:dbl)
          n295 = global read "G_VEH.vi" "S.A. limit deg"() -> (w456:dbl)
          n296 = Subtract(x=w452, y=w453) -> (x-y=w454:dbl)
          n297 = Add(x=w453, y=w452) -> (x+y=w457:dbl)
          n298 = Negate(x=w462) -> (-x=w455:dbl)
          n299 = Max & Min(x=w455, y=w454) -> (max(x,y)=w458:dbl)  [unwired: 1 out]
          n300 = Max & Min(x=w457, y=w456) -> (min(x,y)=w461:dbl)  [unwired: 1 out]
          n301 = flat-sequence {
            tunnel: w461 -> [w508]
            tunnel: [w507] -> w459
            tunnel: w458 -> [w506]
            frame #0 {
              n302 = Subtract(x=w508, y=w506) -> (x-y=w513:dbl)
              n303 = Multiply(x=2.0, y=w513) -> (x*y=w511:dbl)
              n304 = To Long Integer(number=w511) -> (32bit integer=w510:i32)
              n305 = for {
                N: w510 -> [_]
                tunnel: [w517] -> w507 mode=indexing
                tunnel: 0.5 ("x") -> [w516]
                tunnel: w508 -> [w515]
                i -> [w514]
                n306 = Multiply(x=w516, y=w514) -> (x*y=w518:dbl)
                n307 = Subtract(x=w515, y=w518) -> (x-y=w517:dbl)
              }
            }
          }
          n308 = flat-sequence {
            tunnel: w459 -> [w497]
            tunnel: [w496] -> w460
            frame #0 {
              n309 = global read "G_VEH.vi" "ratio_steer"() -> (w499:dbl)
              n310 = global read "G_VEH.vi" "C_Wheel base"() -> (w504:dbl)
              n311 = Divide(x=w497, y=w499) -> (x/y=w503:dbl[])
              n312 = Multiply(x=w503, y=3.141592653589793) -> (x*y=w501:dbl[])
              n313 = Divide(x=w501, y=180.0) -> (x/y=w498:dbl[])
              n314 = Tangent(1:w498) -> (0:w505:dbl[])
              n315 = Divide(x=w504, y=w505) -> (x/y=w496:dbl[])
            }
          }
          "theta" <- w459
          "R" <- w460
        }
        frame #1 {
          n316 = local read "map_track"() -> (w520:dbl[][])
          n317 = disable-structure shown="Enabled" {
            disable-tunnel: [w582 w583 _] -> w519
            disable-tunnel: w520 -> [w581 w584 _]
            frame Disabled {
              n318 = global read "G_VEH.vi" "Reverse"() -> (w563:bool)
              n319 = Select(t=0.2, s=w563, f=0.5) -> (s? t:f=w560:dbl)
              n320 = Array Size(array=w581) -> (size(s)=w580:i32[])
              n321 = local read "RXY"() -> (w537:dbl[])
              n322 = local read "RXY"() -> (w574:dbl[])
              n323 = global read "G_VEH.vi" "candata"() -> (w555:T3)
              n324 = global read "G_PATH.vi" "Mission"() -> (w530:i32)
              n325 = Not Equal?(x=w530, y=9) -> (x != y?=w564:bool)
              n326 = global read "G_VEH.vi" "Reverse"() -> (w559:bool)
              n327 = Index Array(array=w580) -> (element=w531:i32)  [unwired: 1 in]
              n328 = Index Array(array=w537, index=0) -> (element=w536:dbl)
              n329 = Index Array(array=w574, index=0) -> (element=w571:dbl)
              n330 = Unbundle By Name(w555) -> ("VS_can"=w554:dbl)
              n331 = Subtract(x=w571, y=6.0) -> (x-y=w569:dbl)
              n332 = Select(t=5.0 ("y"), s=w559, f=10.0 ("y")) -> (s? t:f=w556:dbl)
              n333 = Less?(x=w536, y=500.0) -> (x < y?=w534:bool)
              n334 = Absolute Value(x=w554) -> (abs(x)=w544:dbl)
              n335 = Multiply(x=0.05, y=w569) -> (x*y=w567:dbl)
              n336 = Less?(x=w544, y=5.0) -> (x < y?=w543:bool)
              n337 = Select(t=0.6, s=w543, f=0.65 ("t")) -> (s? t:f=w540:dbl)
              n338 = Less?(x=w544, y=10.0) -> (x < y?=w548:bool)
              n339 = Select(t=w540, s=w548, f=0.75) -> (s? t:f=w547:dbl)
              n340 = Less?(x=w544, y=15.0) -> (x < y?=w552:bool)
              n341 = Select(t=w547, s=w552, f=0.85 ("upper limit")) -> (s? t:f=w550:dbl)
              n342 = Add(x=w567, y=0.6 ("lower limit")) -> (x+y=w565:dbl)
              n343 = In Range and Coerce(upper limit=w550, x=w565, lower limit=0.6) -> (coerced(x)=w539:dbl)  [unwired: 1 out]
              n344 = Select(t=w539, s=w564, f=w560) -> (s? t:f=w577:dbl)
              n345 = Multiply(x=w531, y=w577) -> (x*y=w579:dbl)
              n346 = Round Toward -Infinity(1:w579) -> (0:w576:dbl)
              n347 = Max & Min(x=w576, y=w556) -> (max(x,y)=w575:dbl)  [unwired: 1 out]
              n348 = Max & Min(x=w531, y=w575) -> (min(x,y)=w533:dbl)  [unwired: 1 out]
              n349 = Select(t=w533, s=w534, f=w531) -> (s? t:f=w532:dbl)
              n350 = Array Subset(array=w581, length (row)=w532) -> (w582:dbl[][])  [unwired: 3 in]
            }
            frame Enabled {
              n351 = flat-sequence {
                tunnel: w584 -> [w593]
                tunnel: [w592] -> w583
                frame #0 {
                  n352 = disable-structure shown="Enabled" {
                    disable-tunnel: [w620 w624] -> w589
                    frame Disabled {
                      n353 = local read "R"() -> (w622:dbl[])
                      n354 = Index Array(array=w622, index=0) -> (element=w621:dbl)
                      n355 = Absolute Value(x=w621) -> (abs(x)=w620:dbl)
                    }
                    frame Enabled {
                      n356 = global read "G_VEH.vi" "ratio_steer"() -> (w635:dbl)
                      n357 = global read "G_VEH.vi" "handle"() -> (w628:dbl)
                      n358 = global read "G_VEH.vi" "C_Wheel base"() -> (w630:dbl)
                      n359 = Absolute Value(x=w628) -> (abs(x)=w627:dbl)
                      n360 = Add(x=w627, y=150.0 ("t")) -> (x+y=w625:dbl)
                      n361 = Divide(x=w625, y=w635) -> (x/y=w631:dbl)
                      n362 = Multiply(x=w631, y=3.141592653589793) -> (x*y=w633:dbl)
                      n363 = Divide(x=w633, y=180.0) -> (x/y=w636:dbl)
                      n364 = Tangent(1:w636) -> (0:w629:dbl)
                      n365 = Divide(x=w630, y=w629) -> (x/y=w624:dbl)
                    }
                  }
                  n366 = Index Array(array=w593, index (col)=0 ("disabled index (col)")) -> (element=w616:dbl[])  [unwired: 1 in]
                  n367 = Index Array(array=w593, index (col)=1 ("disabled index (col)")) -> (element=w605:dbl[])  [unwired: 1 in]
                  n368 = Rotate 1D Array(1:w616, 2:1 ("n")) -> (0:w615:dbl[])
                  n369 = Rotate 1D Array(1:w605, 2:1 ("n")) -> (0:w606:dbl[])
                  n370 = Subtract(x=w616, y=w615) -> (x-y=w614:dbl[])
                  n371 = Subtract(x=w605, y=w606) -> (x-y=w607:dbl[])
                  n372 = Replace Array Subset(array=w614, new element=0.0 ("new element/subarray"), index=0) -> (w611:dbl[])
                  n373 = Replace Array Subset(array=w607, new element=0.0 ("new element/subarray"), index=0) -> (w610:dbl[])
                  n374 = Square(x=w611) -> (x^2=w602:dbl[])
                  n375 = Square(x=w610) -> (x^2=w601:dbl[])
                  n376 = Add(x=w602, y=w601) -> (x+y=w600:dbl[])
                  n377 = Square Root(x=w600) -> (sqrt(x)=w599:dbl[])
                  n378 = for {
                    tunnel: w599 -> [w639] mode=indexing
                    shift-right: [w637] -> _
                    shift-left: 0.0 -> [w638]
                    tunnel: [w637] -> w594 mode=indexing
                    n379 = Add(x=w638, y=w639) -> (x+y=w637:dbl)
                  }
                  n380 = Multiply(x=4.0, y=w589) -> (x*y=w587:dbl)
                  n381 = Subtract(x=w587, y=18.0) -> (x-y=w585:dbl)
                  n382 = Max & Min(x=9.0, y=w585) -> (max(x,y)=w590:dbl)  [unwired: 1 out]
                  n383 = Threshold 1D Array(2:w590, 3:w594) -> (0:w597:dbl)  [unwired: 1 in]
                  n384 = Round Toward +Infinity(x=w597) -> (ceil(x): smallest int >= x=w596:dbl)
                  n385 = To Long Integer(number=w596) -> (32bit integer=w619:i32)
                  n386 = Array Subset(array=w593, index (row)=0 ("index"), length (row)=w619) -> (w592:dbl[][])  [unwired: 2 in]
                }
              }
            }
            frame Disabled {
            }
          }
          n387 = disable-structure shown="Enabled" {
            disable-tunnel: [w522 w523] -> w521
            disable-tunnel: w519 -> [w522 w526]
            frame Enabled {
            }
            frame Disabled {
              n388 = Index Array(array=w526, index (col)=1 ("disabled index (col)")) -> (element=w528:dbl[])  [unwired: 1 in]
              n389 = Add(x=w528, y="Numeric") -> (x+y=w524:dbl[])
              n390 = Replace Array Subset(array=w526, new element=w524, index (col)=1 ("disabled index (col)")) -> (w523:dbl[][])  [unwired: 1 in]
            }
          }
          "track_shift" <- w521
          n391 = global write "G_PATH.vi" "map_track"(w519) -> ()
        }
        frame #2 {
          n392 = local read "R"() -> (w653:dbl[])
          n393 = local read "R"() -> (w642:dbl[])
          n394 = local read "reverse"() -> (w650:bool)
          n395 = Absolute Value(x=w653) -> (abs(x)=w652:dbl[])
          n396 = Absolute Value(x=w642) -> (abs(x)=w643:dbl[])
          n397 = local read "vr"() -> (w649:dbl)
          n398 = local read "vf"() -> (w648:dbl)
          n399 = local read "vw"() -> (w641:dbl)
          n400 = local read "vw"() -> (w640:dbl)
          n401 = Select(t=w649, s=w650, f=w648) -> (s? t:f=w647:dbl)
          n402 = Add(x=w652, y=w641) -> (x+y=w651:dbl[])
          n403 = Subtract(x=w643, y=w640) -> (x-y=w655:dbl[])
          n404 = Square(x=w647) -> (x^2=w646:dbl)
          n405 = Square(x=w651) -> (x^2=w645:dbl[])
          n406 = Add(x=w646, y=w645) -> (x+y=w644:dbl[])
          n407 = Square Root(x=w644) -> (sqrt(x)=w654:dbl[])
        }
        frame #3 {
          n408 = local read "R"() -> (w660:dbl[])
          n409 = Negate(x=w660) -> (-x=w659:dbl[])
          n410 = for {
            tunnel: w659 -> [w752] mode=indexing
            tunnel: [w755] -> w656 mode=indexing
            tunnel: w658 -> [w754] mode=indexing
            tunnel: w657 -> [w753] mode=indexing
            n411 = Absolute Value(x=w752) -> (abs(x)=w751:dbl)
            n412 = Less Or Equal?(x=w751, y=10000.0) -> (x <= y?=w756:bool)
            n413 = case shown="True" w756 {
              tunnel: [w761 w776] -> w755
              tunnel: w754 -> [_ w788]
              tunnel: w753 -> [_ w793]
              tunnel: w752 -> [_ w800]
              tunnel: w751 -> [_ w787]
              frame False {
                w766 = 1.0
                n414 = local read "track_shift"() -> (w775:dbl[][])
                n415 = local read "vw"() -> (w758:dbl)
                n416 = Negate(x=w758) -> (-x=w760:dbl)
                n417 = local read "vw"() -> (w759:dbl)
                n418 = Index Array(array=w775, index (col)=0 ("disabled index (col)")) -> (element=w772:dbl[])  [unwired: 1 in]
                n419 = In Range and Coerce(upper limit=w759, x=w772, lower limit=w760) -> (In Range?=w773:bool[])  [unwired: 1 out]
                n420 = Absolute Value(x=w772) -> (abs(x)=w771:dbl[])
                n421 = Divide(x=w771, y=w759) -> (x/y=w770:dbl[])
                n422 = Boolean To (0,1)(Boolean=w773) -> (0, 1=w763:i16[])
                n423 = Multiply(x=w770, y=0.5) -> (x*y=w768:dbl[])
                n424 = Subtract(x=w766, y=w768) -> (x-y=w767:dbl[])
                n425 = In Range and Coerce(upper limit=w766, x=w767, lower limit=0.0) -> (coerced(x)=w764:dbl[])  [unwired: 1 out]
                n426 = Multiply(x=w764, y=w763) -> (x*y=w762:dbl[])
                n427 = Add Array Elements(numeric array=w762) -> (sum=w761:dbl)
              }
              frame True {
                w781 = 1.0
                n428 = Subtract(x=w788, y=w787) -> (x-y=w786:dbl)
                n429 = local read "track_shift"() -> (w803:dbl[][])
                n430 = Index Array(array=w803, index (col) #1=1 ("disabled index (col)"), index (col) #2=0 ("disabled index (col)")) -> (element #1=w797:dbl[], element #2=w801:dbl[])  [unwired: 2 in]
                n431 = Subtract(x=w801, y=w800) -> (x-y=w799:dbl[])
                n432 = Square(x=w797) -> (x^2=w796:dbl[])
                n433 = Square(x=w799) -> (x^2=w795:dbl[])
                n434 = Add(x=w796, y=w795) -> (x+y=w794:dbl[])
                n435 = Square Root(x=w794) -> (sqrt(x)=w791:dbl[])
                n436 = Subtract(x=w791, y=w787) -> (x-y=w790:dbl[])
                n437 = In Range and Coerce(upper limit=w788, x=w791, lower limit=w793) -> (In Range?=w792:bool[])  [unwired: 1 out]
                n438 = Absolute Value(x=w790) -> (abs(x)=w789:dbl[])
                n439 = Boolean To (0,1)(Boolean=w792) -> (0, 1=w778:i16[])
                n440 = Divide(x=w789, y=w786) -> (x/y=w785:dbl[])
                n441 = Multiply(x=w785, y=0.5) -> (x*y=w783:dbl[])
                n442 = Subtract(x=w781, y=w783) -> (x-y=w782:dbl[])
                n443 = In Range and Coerce(upper limit=w781, x=w782, lower limit=0.0) -> (coerced(x)=w779:dbl[])  [unwired: 1 out]
                n444 = Multiply(x=w779, y=w778) -> (x*y=w777:dbl[])
                n445 = Add Array Elements(numeric array=w777) -> (sum=w776:dbl)
              }
            }
          }
          n446 = flat-sequence {
            tunnel: w656 -> [w664]
            frame #0 {
              n447 = disable-structure shown="Enabled" {
                disable-tunnel: w664 -> [w672 _]
                disable-tunnel: [w665 w727] -> w663
                frame Enabled {
                  n448 = Add Array Elements(numeric array=w672) -> (sum=w674:dbl)
                  n449 = flat-sequence {
                    tunnel: [w693] -> w671
                    tunnel: [w692] -> w669
                    tunnel: [w684] -> w666
                    frame #0 {
                      n450 = local read "RXY"() -> (w690:dbl[])
                      n451 = global read "G_PATH.vi" "Mission"() -> (w676:i32)
                      n452 = global read "G_PATH.vi" "Mission"() -> (w675:i32)
                      n453 = global read "G_VEH.vi" "handle"() -> (w694:dbl)
                      n454 = Index Array(array=w690, index=0) -> (element=w688:dbl)
                      n455 = Absolute Value(x=w688) -> (abs(x)=w687:dbl)
                      n456 = Not Equal?(x=w676, y=9) -> (x != y?=w678:bool)
                      n457 = Equal?(x=w675, y=9) -> (x = y?=w682:bool)
                      n458 = Less Or Equal?(x=w687, y=15.0) -> (x <= y?=w677:bool)
                      n459 = And(x=w678, y=w677) -> (x .and. y?=w684:bool)
                      n460 = Select(t=0.5, s=w677, f="a") -> (s? t:f=w679:dbl)
                      n461 = Select(t=w679, s=w682, f=0.1) -> (s? t:f=w691:dbl)
                      n462 = Multiply(x=w694, y=w691) -> (x*y=w692:dbl)
                      n463 = Decrement(x=w691) -> (x-1=w693:dbl)
                    }
                  }
                  n464 = Not Equal To 0?(x=w674) -> (x != 0?=w673:bool)
                  n465 = case shown="True" w673 {
                    tunnel: [w707 w716] -> w670
                    tunnel: w672 -> [_ w724]
                    frame False {
                      n466 = global read "G_VEH.vi" "candata"() -> (w708:T3)
                      n467 = Unbundle By Name(w708) -> ("Steer_output"=w707:dbl)
                    }
                    frame True {
                      n468 = Array Max & Min(array=w724) -> (max value=w718:dbl)  [unwired: 3 out]
                      n469 = global read "G_VEH.vi" "handle"() -> (w715:dbl)
                      n470 = Equal?(x=w724, y=w718) -> (x = y?=w725:bool[])
                      n471 = Absolute Value(x=w715) -> (abs(x)=w714:dbl)
                      n472 = Boolean To (0,1)(Boolean=w725) -> (0, 1=w720:i16[])
                      n473 = local read "theta"() -> (w719:dbl[])
                      n474 = Add Array Elements(numeric array=w720) -> (sum=w723:i16)
                      n475 = Less?(x=w714, y=30.0) -> (x < y?=w712:bool)
                      n476 = Multiply(x=w719, y=w720) -> (x*y=w721:dbl[])
                      n477 = Select(t=1.0, s=w712, f=1.05 ("y")) -> (s? t:f=w710:dbl)
                      n478 = Add Array Elements(numeric array=w721) -> (sum=w722:dbl)
                      n479 = Divide(x=w722, y=w723) -> (x/y=w717:dbl)
                      n480 = Multiply(x=w717, y=w710) -> (x*y=w716:dbl)
                    }
                  }
                  n481 = Multiply(x=w671, y=w670) -> (x*y=w668:dbl)
                  n482 = Subtract(x=w669, y=w668) -> (x-y=w667:dbl)
                  n483 = case shown="False" w666 {
                    tunnel: [w696 w701] -> w665
                    tunnel: w667 -> [w696 w700]
                    frame False {
                    }
                    frame True {
                      n484 = local read "RXY"() -> (w705:dbl[])
                      n485 = Sign(1:w700) -> (0:w703:dbl)
                      n486 = Index Array(array=w705, index=1) -> (element=w704:dbl)
                      n487 = Sign(1:w704) -> (0:w699:dbl)
                      n488 = Equal?(x=w703, y=w699) -> (x = y?=w702:bool)
                      n489 = Multiply(x=-0.01, y=w699) -> (x*y=w697:dbl)
                      n490 = Select(t=w697, s=w702, f=w700) -> (s? t:f=w701:dbl)
                    }
                  }
                }
                frame Disabled {
                  n491 = global read "G_VEH.vi" "ratio_steer"() -> (w734:dbl)
                  n492 = global read "G_VEH.vi" "C_Wheel base"() -> (w737:dbl)
                  n493 = global read "G_SEN.vi" "lane_center 2"() -> (w749)
                  n494 = local read item#-1() -> (w747)
                  n495 = local read item#-1() -> (w746)
                  n496 = local read item#-1() -> (w745)
                  n497 = call "rotm_siso.vi"("angle[rad]"=w745, "reverse"=TRUE, "y0"=w746, "x0"=w747, "y"=4.5, "x"=w749) -> ("y'"=w744:dbl, "x'"=w741:dbl)  [unwired: 4 in]
                  n498 = Square(x=w741) -> (x^2=w743:dbl)
                  n499 = Square(x=w744) -> (x^2=w742:dbl)
                  n500 = Multiply(x=w741, y=-2.0) -> (x*y=w738:dbl)
                  n501 = Add(x=w743, y=w742) -> (x+y=w739:dbl)
                  n502 = Divide(x=w739, y=w738) -> (x/y=w736:dbl)
                  n503 = Divide(x=w737, y=w736) -> (x/y=w735:dbl)
                  n504 = Inverse Tangent(1:w735) -> (0:w733:dbl)
                  n505 = Multiply(x=w734, y=w733) -> (x*y=w732:dbl)
                  n506 = Divide(x=w732, y=3.141592653589793) -> (x/y=w730:dbl)
                  n507 = Multiply(x=w730, y=180.0) -> (x*y=w728:dbl)
                  n508 = Multiply(x=w728, y=0.97) -> (x*y=w727:dbl)
                }
              }
              n509 = Add(x=w663, y=0.0) -> (x+y=→"theta handle":dbl)
            }
          }
        }
      }
    }
    frame #5 {
      n510 = flat-sequence {
        frame #0 {
          n511 = global read "G_PATH.vi" "RXY"() -> (w808:dbl[])
          n512 = global read "G_NAV.vi" "M6006"() -> (w813:T1)
          n513 = Index Array(array=w808) -> (element=w807:dbl)  [unwired: 1 in]
          n514 = Unbundle By Name(w813) -> ("lcc[1]"=w818:dbl, "lcc[0]"=w817:dbl, "attitude[2]"=w819:dbl)
          n515 = Greater?(x=w807, y=75.0) -> (0:w805:bool)
          n516 = case shown="False" w805 {
            tunnel: [w822 w824] -> w804
            frame False {
              n517 = global read "G_SEN.vi" "sensor_obs_log"() -> (w823:dbl[][])
              n518 = Build Array (concatenate)(w823) -> (w822:dbl[][])
            }
            frame True {
              n519 = global read "G_SEN.vi" "sensor_obs_log"() -> (w824:dbl[][])
            }
          }
          n520 = Negate(x=w819) -> (-x=w816:dbl)
          n521 = Index Array(array=w804, index (col) #1=0 ("disabled index (col)")) -> (element #1=w820:dbl[], element #2=w821:dbl[])  [unwired: 3 in]
          n522 = call "rotm_obs_new.vi"("angle[rad]"=w816, "reverse"=FALSE, "y0"=w817, "x0"=w818, "y"=w821, "x"=w820) -> ("rot*(y-y0) 2"=w811:dbl[], "rot*(x-x0)"=w812:dbl[])  [unwired: 2 in, 2 out]
          n523 = Build Array(w812, w811) -> (w810:dbl[][])
          n524 = Transpose 2D Array(2D array=w810) -> (transposed array=→"sensor_obs":dbl[][])
        }
        frame #1 {
          n525 = local read "rd"() -> (w831:dbl)
          n526 = Equal To 0?(x=w831) -> (x = 0?=w830:bool)
          n527 = case shown="False" w830 {
            tunnel: [w843 w984] -> w829
            tunnel: [w845 w983] -> w828
            tunnel: [w841 w982] -> w827
            tunnel: [w835 w978] -> w825
            tunnel: [w834 w979] -> w826
            frame False {
              n528 = flat-sequence {
                tunnel: [w924] -> w836
                tunnel: w836 -> [w956]
                tunnel: [w955] -> w834
                tunnel: [w954] -> w835
                frame #0 {
                  n529 = global read "G_PATH.vi" "map_track"() -> (w909:dbl[][])
                  n530 = Index Array(array=w909, index (col) #1=1 ("disabled index (col)"), index (col) #2=0 ("index (col)")) -> (element #1=w911:dbl[], element #2=w917:dbl[])  [unwired: 2 in]
                  n531 = local read "aa"() -> (w910:dbl)
                  n532 = Negate(x=w917) -> (-x=w915:dbl[])
                  n533 = Subtract(x=w911, y=w910) -> (x-y=w914:dbl[])
                  n534 = local read "bb"() -> (w916:dbl)
                  n535 = Subtract(x=w915, y=w916) -> (x-y=w913:dbl[])
                  n536 = Re/Im To Polar(2:w913, 3:w914) -> (0:→"thetaseed":dbl[])  [unwired: 1 out]
                }
                frame #1 {
                  n537 = global read "G_PATH.vi" "lane_width"() -> (w948:dbl)
                  n538 = global read "G_PATH.vi" "lane_width"() -> (w935:dbl)
                  n539 = local read "rd"() -> (w929:dbl)
                  n540 = local read "vw"() -> (w930:dbl)
                  n541 = local read "rd"() -> (w932:dbl)
                  n542 = local read "vw"() -> (w933:dbl)
                  n543 = local read "vf"() -> (w927:dbl)
                  n544 = Add(x=w929, y=w930) -> (x+y=w928:dbl)
                  n545 = Square(x=w927) -> (x^2=w925:dbl)
                  n546 = Subtract(x=w932, y=w933) -> (x-y=w921:dbl)
                  n547 = Square(x=w928) -> (x^2=w926:dbl)
                  n548 = Multiply(x=w935, y=0.5) -> (x*y=w938:dbl)
                  n549 = Multiply(x=w948, y=-0.5) -> (x*y=w945:dbl)
                  n550 = local read "rd"() -> (w946:dbl)
                  n551 = local read "rd"() -> (w937:dbl)
                  n552 = Add(x=w926, y=w925) -> (x+y=w931:dbl)
                  n553 = Add(x=w946, y=w945) -> (x+y=w942:dbl)
                  n554 = Add(x=w937, y=w938) -> (x+y=w941:dbl)
                  n555 = Square Root(x=w931) -> (sqrt(x)=w934:dbl)
                  n556 = Subtract(x=w942, y=0.25) -> (x-y=w949:dbl)
                  n557 = Add(x=w942, y=0.25) -> (x+y=w950:dbl)
                  n558 = Subtract(x=w941, y=0.25) -> (x-y=w922:dbl)
                  n559 = Add(x=w941, y=0.25) -> (x+y=w923:dbl)
                  n560 = local read "rd"() -> (w920:dbl)
                  n561 = Build Array(w949, w950, w934, w920, w921, w922, w923) -> (w924:dbl[])
                }
                frame #2 {
                  n562 = local read "thetaseed"() -> (w953:dbl[])
                  n563 = Sine & Cosine(0:w953) -> (1:w952:dbl[], 2:w951:dbl[])
                  n564 = for {
                    tunnel: w956 -> [w967] mode=indexing
                    tunnel: [w963] -> w955 mode=indexing
                    tunnel: [w959] -> w954 mode=indexing
                    tunnel: w952 -> [w958]
                    tunnel: w951 -> [w957]
                    n565 = Multiply(x=w967, y=w958) -> (x*y=w969:dbl[])
                    n566 = Multiply(x=w967, y=w957) -> (x*y=w971:dbl[])
                    n567 = local read "bb"() -> (w968:dbl)
                    n568 = local read "aa"() -> (w970:dbl)
                    n569 = Add(x=w971, y=w970) -> (x+y=w961:dbl[])
                    n570 = Add(x=w968, y=w969) -> (x+y=w966:dbl[])
                    n571 = Build Cluster Array(w966) -> (w965:cluster{dbl[]}[])
                    n572 = Build Cluster Array(w961) -> (w960:cluster{dbl[]}[])
                    n573 = Index Array(array=w965, index=0) -> (element=w963:cluster{dbl[]})
                    n574 = Index Array(array=w960, index=0) -> (element=w959:cluster{dbl[]})
                  }
                }
              }
              n575 = global read "G_PATH.vi" "lane_width"() -> (w897:dbl)
              n576 = global read "G_PATH.vi" "lane_width"() -> (w871:dbl)
              n577 = local read "sensor_obs"() -> (w833:dbl[][])
              n578 = global read "G_PATH.vi" "map_track"() -> (w832:dbl[][])
              n579 = local read "rd"() -> (w856:dbl)
              n580 = local read "vw"() -> (w857:dbl)
              n581 = local read "rd"() -> (w860:dbl)
              n582 = local read "vw"() -> (w858:dbl)
              n583 = local read "bb"() -> (w844:dbl)
              n584 = local read "vf"() -> (w854:dbl)
              n585 = Square(x=w854) -> (x^2=w852:dbl)
              n586 = Greater Than 0?(x=w844) -> (x > 0?=w839:bool)
              n587 = Add(x=w856, y=w857) -> (x+y=w855:dbl)
              n588 = Subtract(x=w860, y=w858) -> (x-y=w859:dbl)
              n589 = Square(x=w855) -> (x^2=w853:dbl)
              n590 = Index Array(array=w833, index (col) #1=1 ("disabled index (col)"), index (col) #2=0 ("index (col)")) -> (element #1=w838:dbl[], element #2=w866:dbl[])  [unwired: 2 in]
              n591 = Index Array(array=w832, index (col) #1=1 ("disabled index (col)"), index (col) #2=0 ("index (col)")) -> (element #1=w888:dbl[], element #2=w887:dbl[])  [unwired: 2 in]
              n592 = Multiply(x=w871, y=0.5) -> (x*y=w874:dbl)
              n593 = Multiply(x=w897, y=-0.5) -> (x*y=w894:dbl)
              n594 = local read "aa"() -> (w837:dbl)
              n595 = local read "rd"() -> (w895:dbl)
              n596 = local read "rd"() -> (w873:dbl)
              n597 = Add(x=w853, y=w852) -> (x+y=w851:dbl)
              n598 = Square(x=w838) -> (x^2=w864:dbl[])
              n599 = Square(x=w866) -> (x^2=w863:dbl[])
              n600 = Square(x=w888) -> (x^2=w886:dbl[])
              n601 = Square(x=w887) -> (x^2=w885:dbl[])
              n602 = Negate(x=w866) -> (-x=w906:dbl[])
              n603 = Add(x=w895, y=w894) -> (x+y=w893:dbl)
              n604 = Add(x=w873, y=w874) -> (x+y=w875:dbl)
              n605 = Subtract(x=w838, y=w837) -> (x-y=w904:dbl[])
              n606 = local read "bb"() -> (w905:dbl)
              n607 = Add(x=w864, y=w863) -> (x+y=w865:dbl[])
              n608 = Add(x=w886, y=w885) -> (x+y=w884:dbl[])
              n609 = Subtract(x=w906, y=w905) -> (x-y=w903:dbl[])
              n610 = Square Root(x=w865) -> (sqrt(x)=w862:dbl[])
              n611 = Square Root(x=w884) -> (sqrt(x)=w883:dbl[])
              n612 = Add(x=0.25, y=w893) -> (x+y=w892:dbl)
              n613 = Subtract(x=w893, y=0.25) -> (x-y=w891:dbl)
              n614 = Add(x=0.25, y=w875) -> (x+y=w876:dbl)
              n615 = Subtract(x=w875, y=0.25) -> (x-y=w877:dbl)
              n616 = Array Max & Min(array=w883) -> (max value=w882:dbl)  [unwired: 3 out]
              n617 = Square(x=w904) -> (x^2=w902:dbl[])
              n618 = Square(x=w903) -> (x^2=w901:dbl[])
              n619 = Add(x=w902, y=w901) -> (x+y=w900:dbl[])
              n620 = Less?(x=w862, y=w882) -> (x < y?=w846:bool[])
              n621 = Square Root(x=w851) -> (sqrt(x)=w850:dbl)
              n622 = Square Root(x=w900) -> (sqrt(x)=w861:dbl[])
              n623 = In Range and Coerce(upper limit=w850, x=w861, lower limit=w859) -> (In Range?=w847:bool[])  [unwired: 1 out]
              n624 = In Range and Coerce(upper limit=w892, x=w861, lower limit=w891) -> (In Range?=w881:bool[])  [unwired: 1 out]
              n625 = In Range and Coerce(upper limit=w876, x=w861, lower limit=w877) -> (In Range?=w878:bool[])  [unwired: 1 out]
              n626 = And(x=w847, y=w846) -> (x .and. y?=w848:bool[])
              n627 = And(x=w881, y=w846) -> (x .and. y?=w880:bool[])
              n628 = And(x=w878, y=w846) -> (x .and. y?=w867:bool[])
              n629 = Boolean To (0,1)(Boolean=w848) -> (0, 1=w849:i16[])
              n630 = Boolean To (0,1)(Boolean=w880) -> (0, 1=w879:i16[])
              n631 = Boolean To (0,1)(Boolean=w867) -> (0, 1=w868:i16[])
              n632 = Add Array Elements(numeric array=w849) -> (sum=w845:i16)
              n633 = Add Array Elements(numeric array=w879) -> (sum=w842:i16)
              n634 = Add Array Elements(numeric array=w868) -> (sum=w840:i16)
              n635 = case shown="True" w839 {
                tunnel: [w972 w975] -> w843
                tunnel: w842 -> [w973 w975]
                tunnel: [w973 w974] -> w841
                tunnel: w840 -> [w972 w974]
                frame False {
                }
                frame True {
                }
              }
            }
            frame True {
              n636 = flat-sequence {
                tunnel: [w1026] -> w979
                tunnel: [w1025] -> w978
                frame #0 {
                  n637 = local read "vw"() -> (w1040:dbl)
                  n638 = global read "G_PATH.vi" "lane_width"() -> (w1045:dbl)
                  n639 = global read "G_PATH.vi" "lane_width"() -> (w1035:dbl)
                  n640 = global read "G_PATH.vi" "map_track"() -> (w1022:dbl[][])
                  n641 = Index Array(array=w1022, index (col)=1 ("disabled index (col)")) -> (element=w1023:dbl[])  [unwired: 1 in]
                  n642 = Multiply(x=w1045, y=0.5) -> (x*y=w1044:dbl)
                  n643 = Multiply(x=w1035, y=-0.5) -> (x*y=w1036:dbl)
                  n644 = local read "aa"() -> (w1028:dbl)
                  n645 = Negate(x=w1040) -> (-x=w1039:dbl)
                  n646 = Add(x=0.25, y=w1044) -> (x+y=w1043:dbl)
                  n647 = Subtract(x=w1044, y=0.25) -> (x-y=w1042:dbl)
                  n648 = Add(x=0.25, y=w1036) -> (x+y=w1031:dbl)
                  n649 = Subtract(x=w1036, y=0.25) -> (x-y=w1030:dbl)
                  n650 = Multiply(x=w1023, y=w1028) -> (x*y=w1024:dbl[])
                  n651 = Build Array(w1043, w1042, w1040, 0.0 ("element"), w1039, w1031, w1030) -> (w1038:dbl[])
                  n652 = local read "bb"() -> (w1037:dbl)
                  n653 = Add(x=w1038, y=w1037) -> (x+y=w1027:dbl[])
                  n654 = for {
                    tunnel: w1027 -> [w1051] mode=indexing
                    tunnel: [w1055] -> w1026 mode=indexing
                    tunnel: [w1052] -> w1025 mode=indexing
                    tunnel: w1024 -> [w1050]
                    tunnel: w1023 -> [w1049]
                    n655 = Add(x=w1050, y=w1051) -> (x+y=w1058:dbl[])
                    n656 = Build Cluster Array(w1049) -> (w1053:cluster{"map_track":dbl[]}[])
                    n657 = Build Cluster Array(w1058) -> (w1057:cluster{dbl[]}[])
                    n658 = Index Array(array=w1053, index=0) -> (element=w1052:cluster{"map_track":dbl[]})
                    n659 = Index Array(array=w1057, index=0) -> (element=w1055:cluster{dbl[]})
                  }
                }
              }
              n660 = local read "vw"() -> (w980:dbl)
              n661 = local read "aa"() -> (w1017:dbl)
              n662 = global read "G_PATH.vi" "lane_width"() -> (w1014:dbl)
              n663 = local read "sensor_obs"() -> (w977:dbl[][])
              n664 = global read "G_PATH.vi" "map_track"() -> (w976:dbl[][])
              n665 = Square(x=w1017) -> (x^2=w1010:dbl)
              n666 = Increment(x=w1010) -> (x+1=w1009:dbl)
              n667 = Index Array(array=w977, index (col) #1=0 ("disabled index (col)")) -> (element #1=w1019:dbl[], element #2=w1002:dbl[])  [unwired: 3 in]
              n668 = Index Array(array=w976, index (col)=1 ("disabled index (col)")) -> (element=w1004:dbl[])  [unwired: 1 in]
              n669 = Multiply(x=w1014, y=0.5) -> (x*y=w995:dbl)
              n670 = Multiply(x=w1002, y=w1017) -> (x*y=w1018:dbl[])
              n671 = Array Max & Min(array=w1004) -> (max value=w1003:dbl)  [unwired: 3 out]
              n672 = Square Root(x=w1009) -> (sqrt(x)=w1015:dbl)
              n673 = Negate(x=w995) -> (-x=w996:dbl)
              n674 = local read "bb"() -> (w1016:dbl)
              n675 = Compound Arithmetic op=ADD(w1019, w1018, w1016) -> (w1020:dbl[])
              n676 = Divide(x=w1020, y=w1015) -> (x/y=w1011:dbl[])
              n677 = Negate(x=w980) -> (-x=w981:dbl)
              n678 = Negate(x=w1011) -> (-x=w989:dbl[])
              n679 = Add(x=0.25, y=w995) -> (x+y=w1006:dbl)
              n680 = Subtract(x=w995, y=0.25) -> (x-y=w991:dbl)
              n681 = Add(x=0.25, y=w996) -> (x+y=w990:dbl)
              n682 = Subtract(x=w996, y=0.25) -> (x-y=w999:dbl)
              n683 = In Range and Coerce(upper limit=w980, x=w989, lower limit=w981) -> (In Range?=w988:bool[])  [unwired: 1 out]
              n684 = In Range and Coerce(upper limit=w1006, x=w989, lower limit=w991) -> (In Range?=w1001:bool[])  [unwired: 1 out]
              n685 = In Range and Coerce(upper limit=w990, x=w989, lower limit=w999) -> (In Range?=w994:bool[])  [unwired: 1 out]
              n686 = Less?(x=w1002, y=w1003) -> (x < y?=w987:bool[])
              n687 = And(x=w988, y=w987) -> (x .and. y?=w985:bool[])
              n688 = And(x=w1001, y=w987) -> (x .and. y?=w1000:bool[])
              n689 = And(x=w994, y=w987) -> (x .and. y?=w992:bool[])
              n690 = Boolean To (0,1)(Boolean=w985) -> (0, 1=w986:i16[])
              n691 = Boolean To (0,1)(Boolean=w1000) -> (0, 1=w1012:i16[])
              n692 = Boolean To (0,1)(Boolean=w992) -> (0, 1=w993:i16[])
              n693 = Add Array Elements(numeric array=w986) -> (sum=w983:i16)
              n694 = Add Array Elements(numeric array=w1012) -> (sum=w984:i16)
              n695 = Add Array Elements(numeric array=w993) -> (sum=w982:i16)
            }
          }
          "left" <- w829
          "right" <- w827
          "center" <- w828
          "yplot" <- w826
          "xplot" <- w825
        }
        frame #2 {
          n696 = disable-structure shown="Disabled" {
            frame Disabled {
              n697 = flat-sequence {
                tunnel: [w1100] -> w1062
                frame #0 {
                  n698 = local read "xplot"() -> (w1098:cluster{dbl[]}[])
                  n699 = Array Size(array=w1098) -> (size(s)=w1099:i32)
                  n700 = Decrement(x=w1099) -> (x-1=w1094:i32)
                  n701 = Index Array(array=w1098, index=w1094) -> (element=w1097:cluster{dbl[]})
                  n702 = Unbundle(w1097) -> (w1096:dbl[])
                  n703 = call "Convert to Dynamic Data5"("Array"=w1096) -> ("Dynamic Data Type"=w1095:dynamicdata)  [unwired: 3 in]
                  n704 = for {
                    N: w1094 -> [_]
                    tunnel: w1098 -> [w1105] mode=indexing
                    shift-right: [w1102] -> w1100
                    shift-left: w1095 -> [w1101]
                    n705 = Unbundle(w1105) -> (w1104:dbl[])
                    n706 = call "Convert to Dynamic Data7"("Array"=w1104) -> ("Dynamic Data Type"=w1103:dynamicdata)  [unwired: 3 in]
                    n707 = Merge Signals(w1101, w1103) -> (w1102:dynamicdata)
                  }
                }
              }
              n708 = flat-sequence {
                tunnel: [w1088] -> w1061
                frame #0 {
                  n709 = local read "yplot"() -> (w1086:cluster{dbl[]}[])
                  n710 = Array Size(array=w1086) -> (size(s)=w1087:i32)
                  n711 = Decrement(x=w1087) -> (x-1=w1082:i32)
                  n712 = Index Array(array=w1086, index=w1082) -> (element=w1085:cluster{dbl[]})
                  n713 = Unbundle(w1085) -> (w1084:dbl[])
                  n714 = call "Convert to Dynamic Data9"("Array"=w1084) -> ("Dynamic Data Type"=w1083:dynamicdata)  [unwired: 3 in]
                  n715 = for {
                    N: w1082 -> [_]
                    tunnel: w1086 -> [w1093] mode=indexing
                    shift-right: [w1090] -> w1088
                    shift-left: w1083 -> [w1089]
                    n716 = Unbundle(w1093) -> (w1092:dbl[])
                    n717 = call "Convert to Dynamic Data6"("Array"=w1092) -> ("Dynamic Data Type"=w1091:dynamicdata)  [unwired: 3 in]
                    n718 = Merge Signals(w1089, w1091) -> (w1090:dynamicdata)
                  }
                }
              }
              n719 = local read "sensor_obs"() -> (w1060:dbl[][])
              n720 = global read "G_PATH.vi" "map_track"() -> (w1059:dbl[][])
              n721 = Index Array(array=w1060, index (col) #1=1 ("disabled index (col)"), index (col) #2=0 ("index (col)")) -> (element #1=w1070:dbl[], element #2=w1071:dbl[])  [unwired: 4 in, 1 out]
              n722 = Index Array(array=w1059, index (col) #1=1 ("disabled index (col)"), index (col) #2=0 ("index (col)")) -> (element #1=w1080:dbl[], element #2=w1075:dbl[])  [unwired: 2 in]
              n723 = Negate(x=w1071) -> (-x=w1072:dbl[])
              n724 = Negate(x=w1075) -> (-x=w1077:dbl[])
              n725 = call "Convert to Dynamic Data"("Array"=w1070) -> ("Dynamic Data Type"=w1066:dynamicdata)  [unwired: 3 in]
              n726 = call "Convert to Dynamic Data4"("Array"=w1080) -> ("Dynamic Data Type"=w1081:dynamicdata)  [unwired: 3 in]
              n727 = call "Convert to Dynamic Data2"("Array"=w1072) -> ("Dynamic Data Type"=w1067:dynamicdata)  [unwired: 3 in]
              n728 = Merge Signals(w1066, w1081) -> (w1079:dynamicdata)
              n729 = call "Convert to Dynamic Data3"("Array"=w1077) -> ("Dynamic Data Type"=w1078:dynamicdata)  [unwired: 3 in]
              n730 = Merge Signals(w1067, w1078) -> (w1076:dynamicdata)
              n731 = Merge Signals(w1079, w1062) -> (w1063:dynamicdata)
              n732 = Merge Signals(w1076, w1061) -> (w1064:dynamicdata)
              n733 = call "Build XY Graph"("Y Input"=w1064, "X Input"=w1063) -> ("XY Graph"=→"XY Graph":cluster{"Y":dbl[], "Y":dbl[]}[])  [unwired: 3 in, 6 out]
            }
            frame Enabled {
            }
          }
        }
        frame #3 {
          n734 = local read "center"() -> (w1109:i16)
          n735 = disable-structure shown="Enabled" {
            disable-tunnel: [w1110 TRUE] -> w1106
            frame Disabled {
              n736 = global read "G_VEH.vi" "candata"() -> (w1113:T3)
              n737 = Unbundle By Name(w1113) -> ("VS_can"=w1112:dbl)
              n738 = Greater?(x=w1112, y=5.0) -> (0:w1110:bool)
            }
            frame Enabled {
            }
          }
          n739 = Equal To 0?(x=w1109) -> (x = 0?=w1107:bool)
          n740 = And(x=w1107, y=w1106) -> ()  [unwired: 1 out]
          n741 = case shown="True" w1106 {
            tunnel: [_ w1115] -> w1108
            frame False {
            }
            frame True {
              n742 = local read "right"() -> (w1119:i16)
              n743 = local read "left"() -> (w1120:i16)
              n744 = Not Equal To 0?(x=w1120) -> (x != 0?=w1118:bool)
              n745 = Not Equal To 0?(x=w1119) -> (x != 0?=w1117:bool)
              n746 = And(x=w1118, y=w1117) -> (x .and. y?=w1116:bool)
              n747 = case shown="False" w1116 {
                tunnel: [w1121 _] -> w1115
                frame False {
                  n748 = local read "left"() -> (w1123:i16)
                  n749 = Not Equal To 0?(x=w1123) -> (x != 0?=w1122:bool)
                  n750 = case shown="True" w1122 {
                    tunnel: [w1130 w1134] -> w1121
                    frame False {
                      n751 = local read "right"() -> (w1132:i16)
                      n752 = local read "rd"() -> (w1128:dbl)
                      n753 = Not Equal To 0?(x=w1132) -> (x != 0?=w1131:bool)
                      n754 = Equal To 0?(x=w1128) -> (x = 0?=w1127:bool)
                      n755 = Select(t=-0.025, s=w1127, f=-0.075) -> (s? t:f=w1124:dbl)
                      n756 = Select(t=w1124, s=w1131, f=0.0) -> (s? t:f=w1130:dbl)
                    }
                    frame True {
                      n757 = local read "rd"() -> (w1137:dbl)
                      n758 = Equal To 0?(x=w1137) -> (x = 0?=w1136:bool)
                      n759 = Select(t=0.025, s=w1136, f=0.075) -> (s? t:f=w1134:dbl)
                    }
                  }
                }
                frame True {
                }
              }
            }
          }
          "shift" <- w1108
        }
      }
    }
  }
